vi "Auto_New.vi"() -> ()   [LabVIEW 2017]
uses:
  Control/Saurabh/prosucer_consumer_enum1.ctl
  Control/OUTPUT Cluster Indicator.ctl
  <vilib>/Utility/error.llb/DialogType.ctl
  <vilib>/addons/database/Connection.llb/DB Tools Open Connec (String).vi
  Global/DATA LOG.vi
  Global/Global 1.vi
  <vilib>/addons/database/NI_Database_API.lvlib
panel:
  out "SHIFT":string
  in  "BARCODE RECIPE":string(combo)
  out "PLC COM.":bool
  out "SHIFT_DATA":string[](array[string])
  out "stop":bool
  out "error out 2":errorcluster
  out "Shift 4":i32
  out "Time Stamp Out":timestamp[](array[timestamp]) format="%<%X>T"
  out "Time Stamp Out 4":timestamp[](array[timestamp]) format="%<%X>T"
  out "Shift_change":bool
  out "appended array":string[][](array[string])
  out "SHIFT_DATA 2":string[](array[string])
  in  "error in (no error)":errorcluster
  in  "Tab Control":T1(tab)
  out "OP 50":bool
  out "OP 40":bool
  out "OP 30":bool
  out "OP - 50":T2 {"RH Motor Screw" format="%#.2g N-m"; "LH Motor Screw" format="%#.2g N-m"; "Nut Torque" format="%#.2g N-m"}
  out "OP - 40":T3 {"Stack Load" format="%.2f kg"; "Dispalcement" format="%#.2g mm"; "LH Screw" format="%#.2g N-m"; "RH Screw" format="%#.2g N-m"}
  out "OP - 30":T4 {"Shaft Press Load" format="%#.2g kg"; "Displacement" format="%#.2g mm"}
  in  "stop 2":bool
  out "OP - 10":T5 {"Leak Rate" format="%#.2g SCCM"}
  in  "SIMULATE INPUT":bool[](array[boolean])=[FALSE, FALSE, FALSE, FALSE]
  out "OP - 20":T6 {"Top Load" format="%#.2g kg"; "Top Displace" format="%#.2g mm"; "Bottom Load" format="%#.2g kg"; "Bottom Displace" format="%#.2g mm"}
  out "OP 10 & 20":bool
  out "OP - 60":T7 {"Screw 6" format="%#.2g N-m"; "Screw 5" format="%#.2g N-m"; "Screw 4" format="%#.2g N-m"; "Screw 3" format="%#.2g N-m"; "Screw 2" format="%#.2g N-m"; "Screw 1" format="%#.2g N-m"}
  out "OP - 70":T8 {"Full Open" format="%#.4g V"; "Full Close" format="%#.4g V"}
  out "OP - 110":T9
  out "OP - 80":T10 {"Plug Press Load" format="%#.2f kg"}
  out "OP - 90":T11 {"Steam Leak" format="%#_g sccm"; "Seat Leak" format="%#_g LPM"}
  out "OP - 100":T12 {"Response Time REV" format="%#_g msec"; "Response time FWD" format="%#_g msec"; "Motor Full Open" format="%#.2f V"; "Motor Start Back" format="%#.2f V"; "Motor Full Close" format="%#.2f V"; "Motor Start Of Close" format="%#.2f V"; "Motor Peak" format="%#.2f A"; "Sensor O/P Full Close" format="%#.2f V"; "Sensor O/P Start Of Close" format="%#.2f V"; "Sensor O/P Open" format="%#.2f V"}
  out "OP 60":bool
  out "OP 70 & 80":bool
  out "OP 90 -100":bool
  out "OP 110":bool
  out "OP110 STATUS":dbl[](array[numeric])
  out "SCAN OP110":string[](array[string])
  out "OP100 STATUS":dbl[](array[numeric])
  out "SCAN OP100":string[](array[string])
  out "OP50 STATUS":dbl[](array[numeric])
  out "SCAN OP50":string[](array[string])
  out "OP90 STATUS":dbl[](array[numeric])
  out "SCAN OP90":string[](array[string])
  out "OP80 STATUS":dbl[](array[numeric])
  out "SCAN OP80":string[](array[string])
  out "OP70 STATUS":dbl[](array[numeric])
  out "SCAN OP70":string[](array[string])
  out "OP60 STATUS":dbl[](array[numeric])
  out "SCAN OP60":string[](array[string])
  out "OP40 STATUS":dbl[](array[numeric])
  out "SCAN OP40":string[](array[string])
  out "OP30 STATUS":dbl[](array[numeric])
  out "SCAN OP30":string[](array[string])
  out "OP20 STATUS":dbl[](array[numeric])
  out "SCAN OP20":string[](array[string])
  out "OP10 STATUS":dbl[](array[numeric])
  out "SCAN OP10":string[](array[string])
  out "resulting string":string
  out "PLC1 error":errorcluster
  out "PLC2 error":errorcluster
  out "PLC3 error":errorcluster
  out "PLC4 error":errorcluster
  out "PLC5 error":errorcluster
  out "PLC6 error":errorcluster
  out "PLC7 error":errorcluster
  out "PLC8 error":errorcluster
  # "Op10 20\nOp30\nOp 40\nOp50\nOp60\nOp70-80\nOp 90-100-110"
  # "SENSOR MIN VLTG"
  # "OP - 50"
  # "OP - 40"
  # "OP - 30"
  # "OP - 10"
  # "OP - 20"
  # "OP - 60"
  # "OP - 70"
  # "OP - 110"
  # "OP - 80"
  # "OP - 90"
  # "OP - 100"
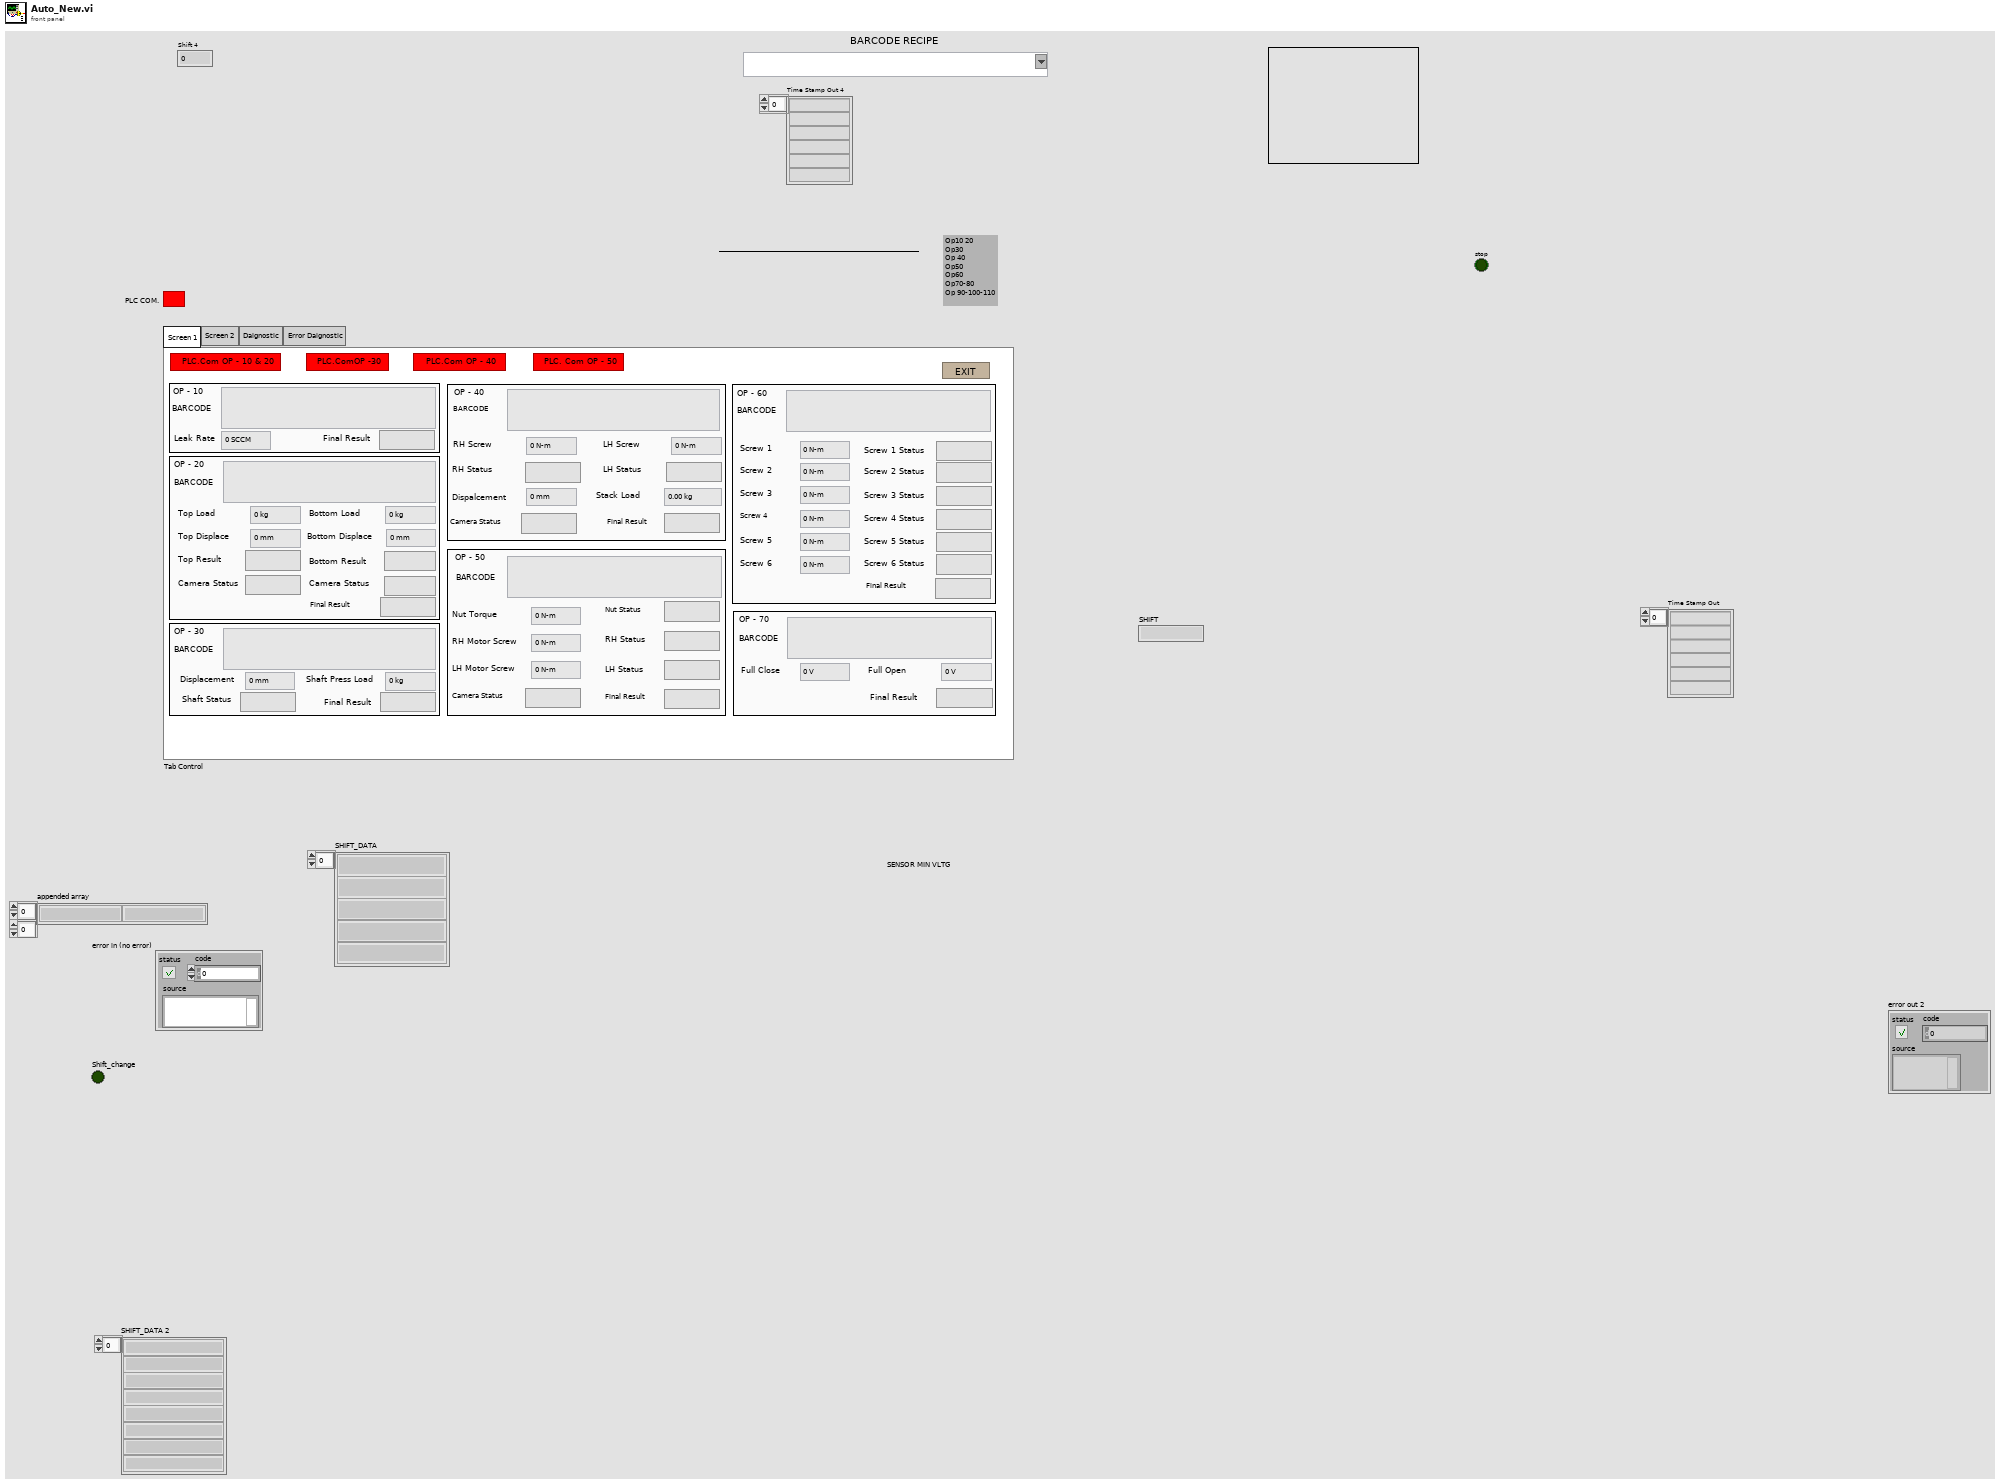
[diagram p1: front panel]
types:
  T1 = enum32{"Screen 1", "Screen 2", "Daignostic", "Error Daignostic"}
  T2 = cluster{"BARCODE":string, "Nut Torque":dbl, "LH Motor Screw":dbl, "LH Status":bool, "RH Status":bool, "RH Motor Screw":dbl, "Final Result":bool, "Nut Status":bool, "Camera Status":bool}
  T3 = cluster{"BARCODE":string, "RH Screw":dbl, "LH Screw ":dbl, "RH Status":bool, "LH Status":bool, "Dispalcement ":dbl, "Stack Load ":dbl, "Final Result":bool, "Camera Status":bool}
  T4 = cluster{"BARCODE":string, "Displacement":dbl, "Shaft Press Load":dbl, "Shaft Status":bool, "Final Result":bool}
  T5 = cluster{"BARCODE":string, "Leak Rate":dbl, "Final Result":bool}
  T6 = cluster{"BARCODE":string, "Bottom Displace":dbl, "Bottom Load":dbl, "Camera Status":bool, "Bottom Result":bool, "Top Displace":dbl, "Top Load ":dbl, "Camera Status":bool, "Top Result":bool, "Final Result":bool}
  T7 = cluster{"BARCODE":string, "Screw 1":dbl, "Screw 2":dbl, "Screw 1 Status":bool, "Screw 2 Status":bool, "Screw 3":dbl, "Final Result":bool, "Screw 3 Status":bool, "Screw 4":dbl, "Screw 5":dbl, "Screw 4 Status":bool, "Screw 5 Status":bool, "Screw 6":dbl, "Screw 6 Status":bool}
  T8 = cluster{"BARCODE":string, "Full Close":dbl, "Full Open":dbl, "Final Result":bool}
  T9 = cluster{"BARCODE":string, "BIN\nNumber":string, "PALLET\nNumber":string}
  T10 = cluster{"BARCODE":string, "Plug Press Load":dbl, "Final Result":bool, "Loctite Status":bool}
  T11 = cluster{"BARCODE":string, "Seat Leak":dbl, "Seat Status":bool, "Steam Leak":dbl, "Final Result":bool}
  T12 = cluster{"BARCODE":string, "Sensor O/P Open":dbl, "Sensor O/P Start Of Close":dbl, "Final Result":bool, "Sensor O/P Full Close":dbl, "Motor Peak":dbl, "Motor Start Of Close":dbl, "Motor Full Close":dbl, "Motor Start Back":dbl, "Motor Full Open":dbl, "Response time FWD":dbl, "Response Time REV":dbl, "Camera Status":bool}
  T13 = typedef "OUTPUT Cluster Indicator.ctl" = cluster{"OP - 10":cluster{"BARCODE":string, "LEAK RATE":dbl, "RESULT":bool}, "OP - 30":cluster{"BARCODE":string, "Displacement":dbl, "Load":dbl, "Middle Gear Shaft Status":bool, "Final Result":bool}, "OP - 60":cluster{"BARCODE":string, "Screw 1 Data":dbl, "Screw 2 data":dbl, "Screw 1 Status":bool, "Screw 2 Status":bool, "Screw3 Data":dbl, "Final Result":bool, "Screw3 Status":bool, "Screw4 Data":dbl, "Screw5 Data":dbl, "Screw4 Status":bool, "Screw5 Status":bool, "Screw6 Data":dbl, "Screw6 Status":bool}, "OP - 70":cluster{"BARCODE":string, "Sensor MIN Vltg":dbl, "Sensor MAX Vltg":dbl, "Final Result":bool}, "OP - 80":cluster{"BARCODE":string, "Load":dbl, "Final Result":bool, "Dispensing":bool}, "OP - 90":cluster{"BARCODE":string, "Seat LT Data":dbl, "Seat Status":bool, "Steam LT Data":dbl, "Final Result":bool}, "OP - 110":cluster{"BARCODE":string, "BIN\nNumber":string, "PALLET\nNumber":string}, "OP - 20":cluster{"BARCODE":string, "Bottom Displace":dbl, "Bottom Load":dbl, "Camera Status":bool, "Bottom Result":bool, "Top Displace":dbl, "Top Load ":dbl, "Camera Status":bool, "Top Result":bool, "Final Result":bool}, "OP - 50":cluster{"BARCODE":string, "Nut Torque":dbl, "LH Motor Screw":dbl, "LH Status":bool, "RH Status":bool, "RH Motor Screw":dbl, "Final Result":bool, "Nut Status":bool, "Camera Status":bool}, "OP - 100":cluster{"BARCODE":string, "Sensor O/P Open":dbl, "Sensor O/P Start Of Close":dbl, "Final Result":bool, "Sensor O/P Full Close":dbl, "Motor Peak":dbl, "Motor Start Of Close":dbl, "Motor Full Close":dbl, "Motor Start Back":dbl, "Motor Full Open":dbl, "Response time FWD":dbl, "Response Time REV":dbl, "Camera Status":bool}, "OP - 40":cluster{"BARCODE":string, "RH Screw":dbl, "LH Screw ":dbl, "RH Status":bool, "LH Status":bool, "Dispalcement ":dbl, "Stack Load ":dbl, "Final Result":bool, "Camera Status":bool}}
  T14 = cluster{"OP - 10":cluster{"BARCODE":string, "LEAK RATE":dbl, "RESULT":bool}, "OP - 30":cluster{"BARCODE":string, "Displacement":dbl, "Load":dbl, "Middle Gear Shaft Status":bool, "Final Result":bool}, "OP - 60":cluster{"BARCODE":string, "Screw 1 Data":dbl, "Screw 2 data":dbl, "Screw 1 Status":bool, "Screw 2 Status":bool, "Screw3 Data":dbl, "Final Result":bool, "Screw3 Status":bool, "Screw4 Data":dbl, "Screw5 Data":dbl, "Screw4 Status":bool, "Screw5 Status":bool, "Screw6 Data":dbl, "Screw6 Status":bool}, "OP - 70":cluster{"BARCODE":string, "Sensor MIN Vltg":dbl, "Sensor MAX Vltg":dbl, "Final Result":bool}, "OP - 80":cluster{"BARCODE":string, "Load":dbl, "Final Result":bool, "Dispensing":bool}, "OP - 90":cluster{"BARCODE":string, "Seat LT Data":dbl, "Seat Status":bool, "Steam LT Data":dbl, "Final Result":bool}, "OP - 110":cluster{"BARCODE":string}, "OP - 20":cluster{"BARCODE":string, "Bottom Displace":dbl, "Bottom Load":dbl, "Camera Status":bool, "Bottom Result":bool, "Top Displace":dbl, "Top Load ":dbl, "Camera Status":bool, "Top Result":bool, "Final Result":bool}, "OP - 40":cluster{"BARCODE":string, "RH Screw":dbl, "LH Screw ":dbl, "RH Status":bool, "LH Status":bool, "Dispalcement ":dbl, "Stack Load ":dbl, "Final Result":bool}, "OP - 50":cluster{"BARCODE":string, "Nut Torque":dbl, "LH Motor Screw":dbl, "LH Status":bool, "RH Status":bool, "RH Motor Screw":dbl, "Final Result":bool, "Nut Status":bool, "Camera Status":bool}, "OP - 100":cluster{"BARCODE":string, "Sensor O/P Open":dbl, "Sensor O/P Start Of Close":dbl, "Final Result":bool, "Sensor O/P Full Close":dbl, "Motor Peak":dbl, "Motor Start Of Close":dbl, "Motor Full Close":dbl, "Motor Start Back":dbl, "Motor Full Open":dbl, "Response time FWD":dbl, "Response Time REV":dbl, "Camera Status":bool}}
  T15 = typedef "prosucer_consumer_enum1.ctl" = enum16{"-1", "SCAN1", "SCAN2", "SCAN3", "SCAN4", "SCAN5", "SCAN6", "SCAN7", "SCAN8", "SCAN9", "SCAN10", "SCAN11", "STOP", "DATALOG1", "DATALOG2", "DATALOG3", "DATALOG4", "DATALOG5", "DATALOG6", "DATALOG7", "DATALOG8", "DATALOG9", "DATALOG10", "DATALOG11", "CYCLE_START1", "CYCLE_START2", "CYCLE_START3", "CYCLE_START4", "BARCODE RECIPE", "EMERGENCY STOP"}
  T16 = typedef "NI_Database_API.lvlib/Conn ObjectReference.ctl" = refnum<k1>
  T17 = typedef "DialogType.ctl" = u16
  T18 = cluster{"trimmed string":string, "SHIFT":string, "date/time string":string, string, "Input 2":string}
  T19 = cluster{"SHIFT":string, "date/time string":string, "Input 2":string, string}
  T20 = cluster{"date/time string":string, "Input 2":string, "Input 2":string, "Input 2":string, "Input 2":string, "Input 2":string, "Input 2":string, "Input 2":string, "Input 2":string, "Input 2":string, "Input 2":string}
  T21 = cluster{"date/time string":string, "SHIFT":string, "Input 2":string, "Input 2":string, "Input 2":string, "Input 2":string, "Input 2":string, "Input 2":string, "Input 2":string, "Input 2":string, "Input 2":string, "Input 2":string}
  T22 = cluster{"date/time string":string, "Input 2":string, "Input 2":string, "Input 2":string, "Input 2":string}
  T23 = cluster{"date/time string":string, "SHIFT":string, "Input 2":string, "Input 2":string, "Input 2":string, "Input 2":string}
  T24 = cluster{"date/time string":string, "Input 2":string, "Input 2":string, "Input 2":string, "Input 2":string, "Input 2":string, "Input 2":string, "Input 2":string, "Input 2":string}
  T25 = cluster{"date/time string":string, "SHIFT":string, "Input 2":string, "Input 2":string, "Input 2":string, "Input 2":string, "Input 2":string, "Input 2":string, "Input 2":string, "Input 2":string}
  T26 = cluster{"date/time string":string, "SHIFT":string, "Input 2":string, "Input 2":string, "Input 2":string, "Input 2":string, "Input 2":string, "Input 2":string}
  T27 = cluster{"date/time string":string, "Input 2":string, "Input 2":string, "Input 2":string, "Input 2":string, "Input 2":string, "Input 2":string, "Input 2":string, "Input 2":string, "Input 2":string, "Input 2":string, "Input 2":string, "Input 2":string, "Input 2":string}
  T28 = cluster{"date/time string":string, "SHIFT":string, "Input 2":string, "Input 2":string, "Input 2":string, "Input 2":string, "Input 2":string, "Input 2":string, "Input 2":string, "Input 2":string, "Input 2":string, "Input 2":string, "Input 2":string, "Input 2":string}
  T29 = cluster{"date/time string":string, "Input 2":string, "Input 2":string, "Input 2":string}
  T30 = cluster{"date/time string":string, "SHIFT":string, "Input 2":string, "Input 2":string, "Input 2":string}
  T31 = cluster{"Input 2":string, "SHIFT":string, "date/time string":string, "Input 2":string, "Input 2":string, "Input 2":string}
  T32 = cluster{"date/time string":string, "trimmed string":string, "trimmed string":string}
  T33 = cluster{"BARCODE":string, "Seat LT Data":dbl, "Seat Status":bool, "Steam LT Data":dbl, "Final Result":bool}
  T34 = cluster{"BARCODE":string, "LEAK RATE":dbl, "RESULT":bool}
  T35 = cluster{"BARCODE":string, "Displacement":dbl, "Load":dbl, "Middle Gear Shaft Status":bool, "Final Result":bool}
  T36 = cluster{"BARCODE":string, "Screw 1 Data":dbl, "Screw 2 data":dbl, "Screw 1 Status":bool, "Screw 2 Status":bool, "Screw3 Data":dbl, "Final Result":bool, "Screw3 Status":bool, "Screw4 Data":dbl, "Screw5 Data":dbl, "Screw4 Status":bool, "Screw5 Status":bool, "Screw6 Data":dbl, "Screw6 Status":bool}
  T37 = cluster{"BARCODE":string, "Sensor MIN Vltg":dbl, "Sensor MAX Vltg":dbl, "Final Result":bool}
  T38 = cluster{"BARCODE":string, "Load":dbl, "Final Result":bool, "Dispensing":bool}
  T39 = enum32{"invalid app kind", "Development System", "Run Time System", "Student Edition", "Embedded LabVIEW", "Evaluation", "Custom"}
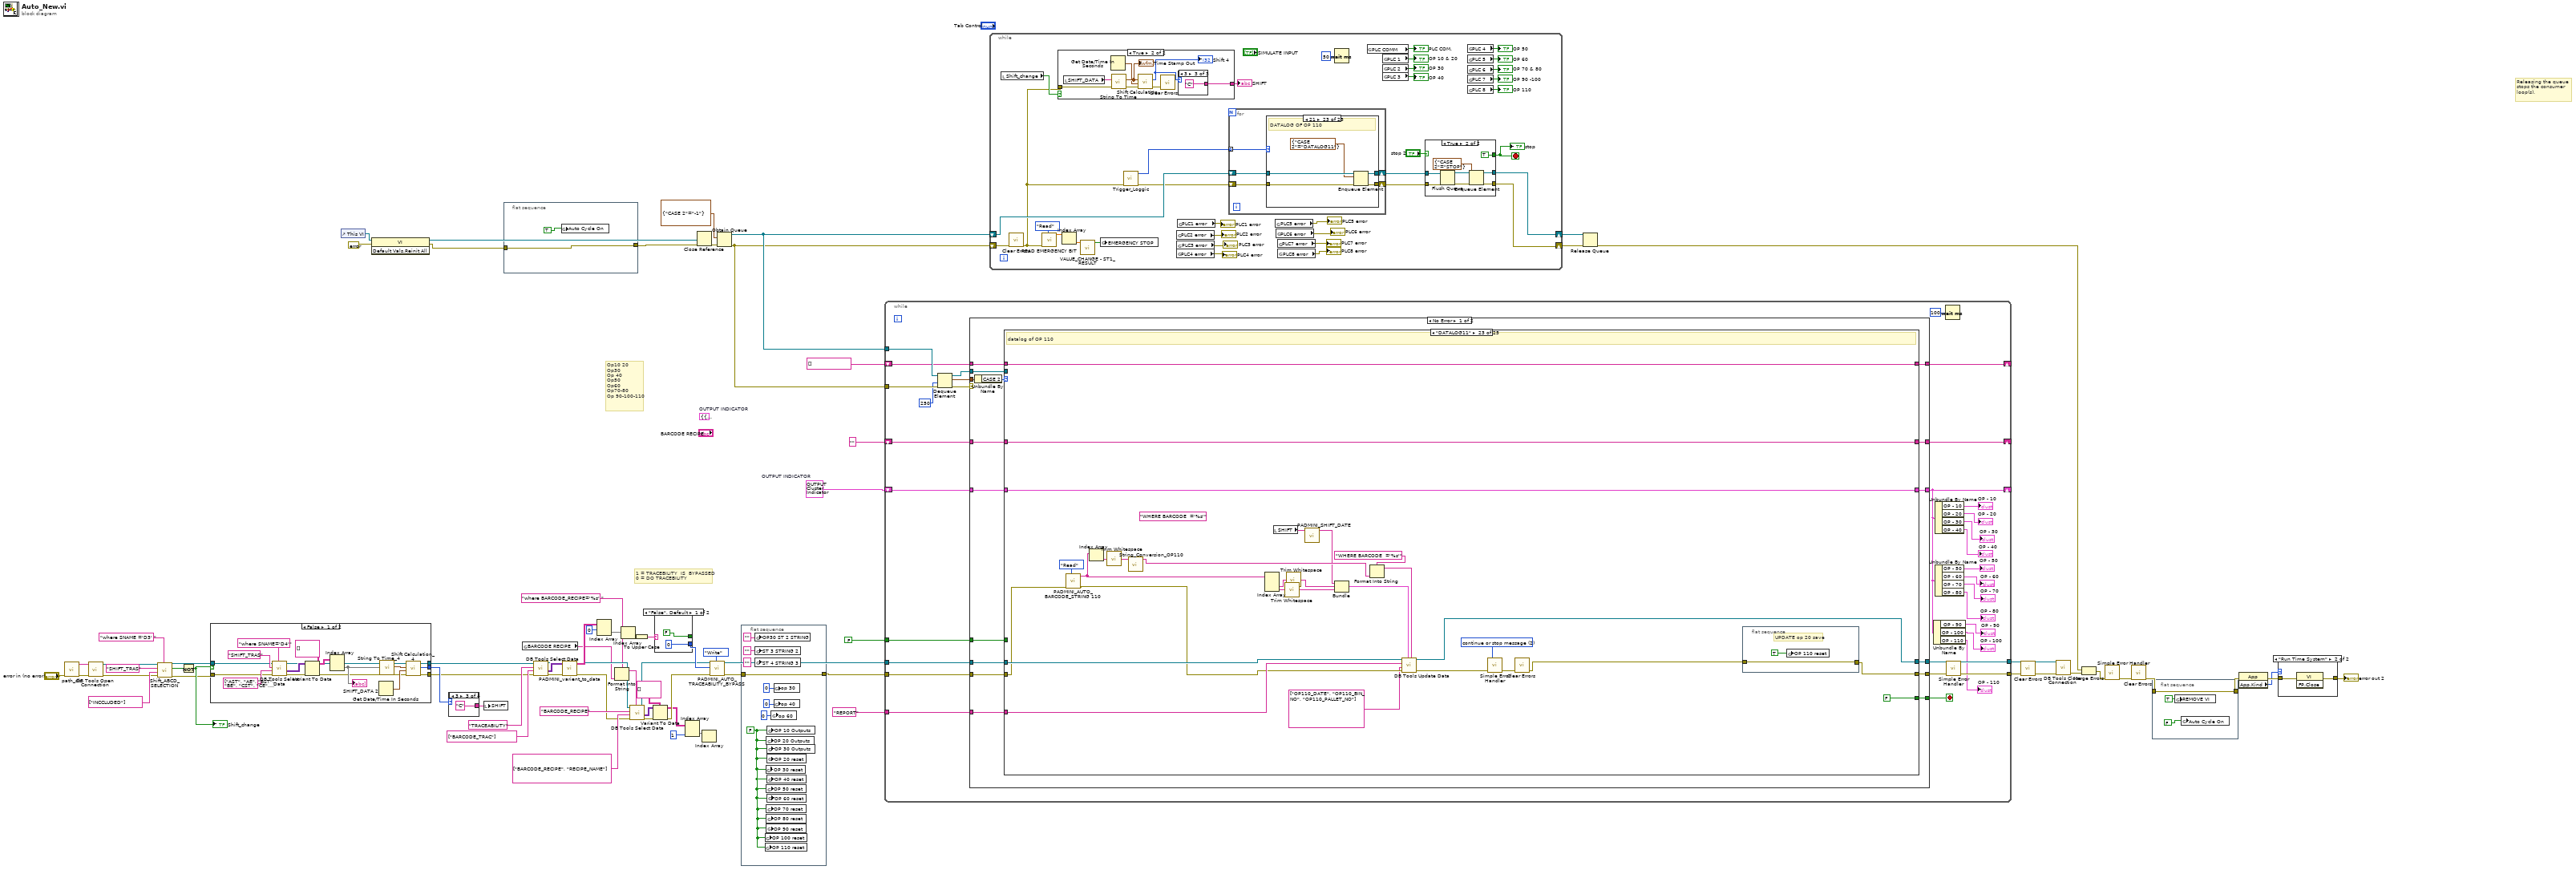
[diagram p0: block diagram]
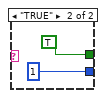
[diagram p2: hidden frame]
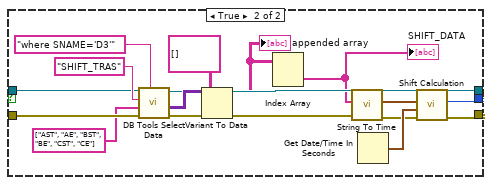
[diagram p3: hidden frame]
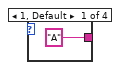
[diagram p4: hidden frame]
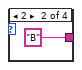
[diagram p5: hidden frame]
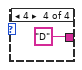
[diagram p6: hidden frame]
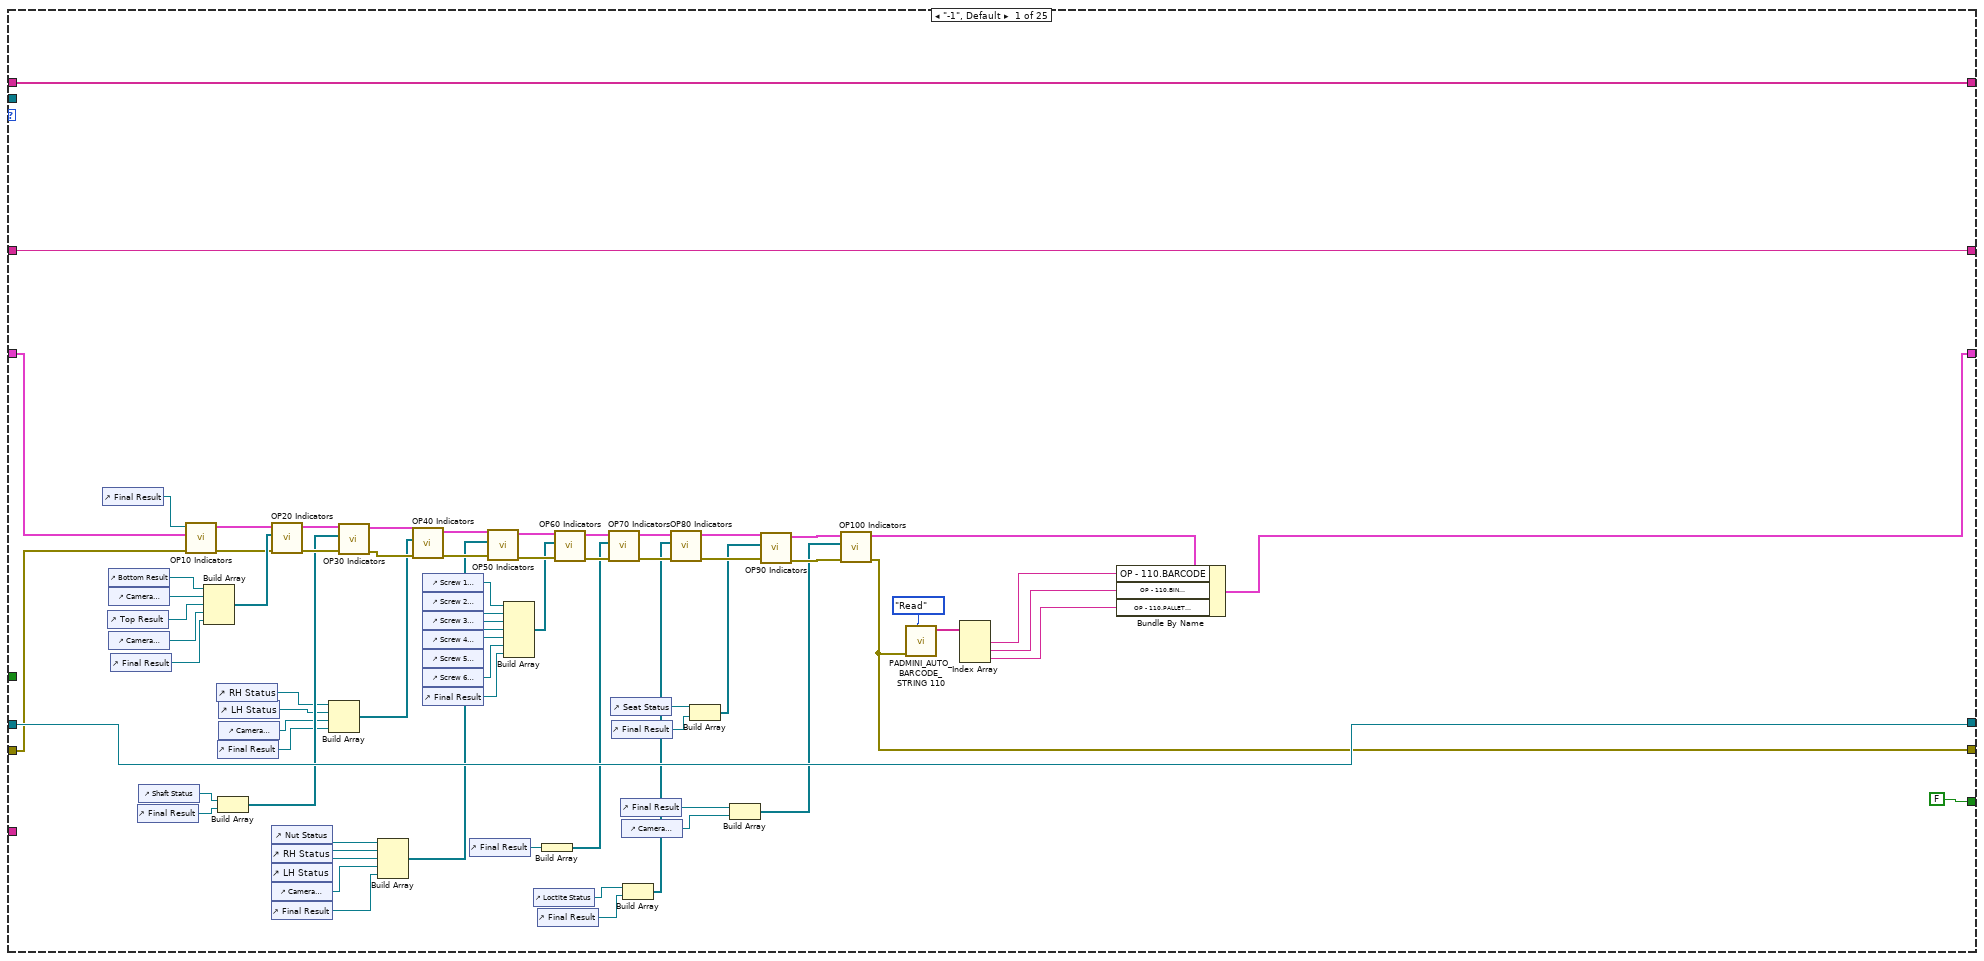
[diagram p7: hidden frame]
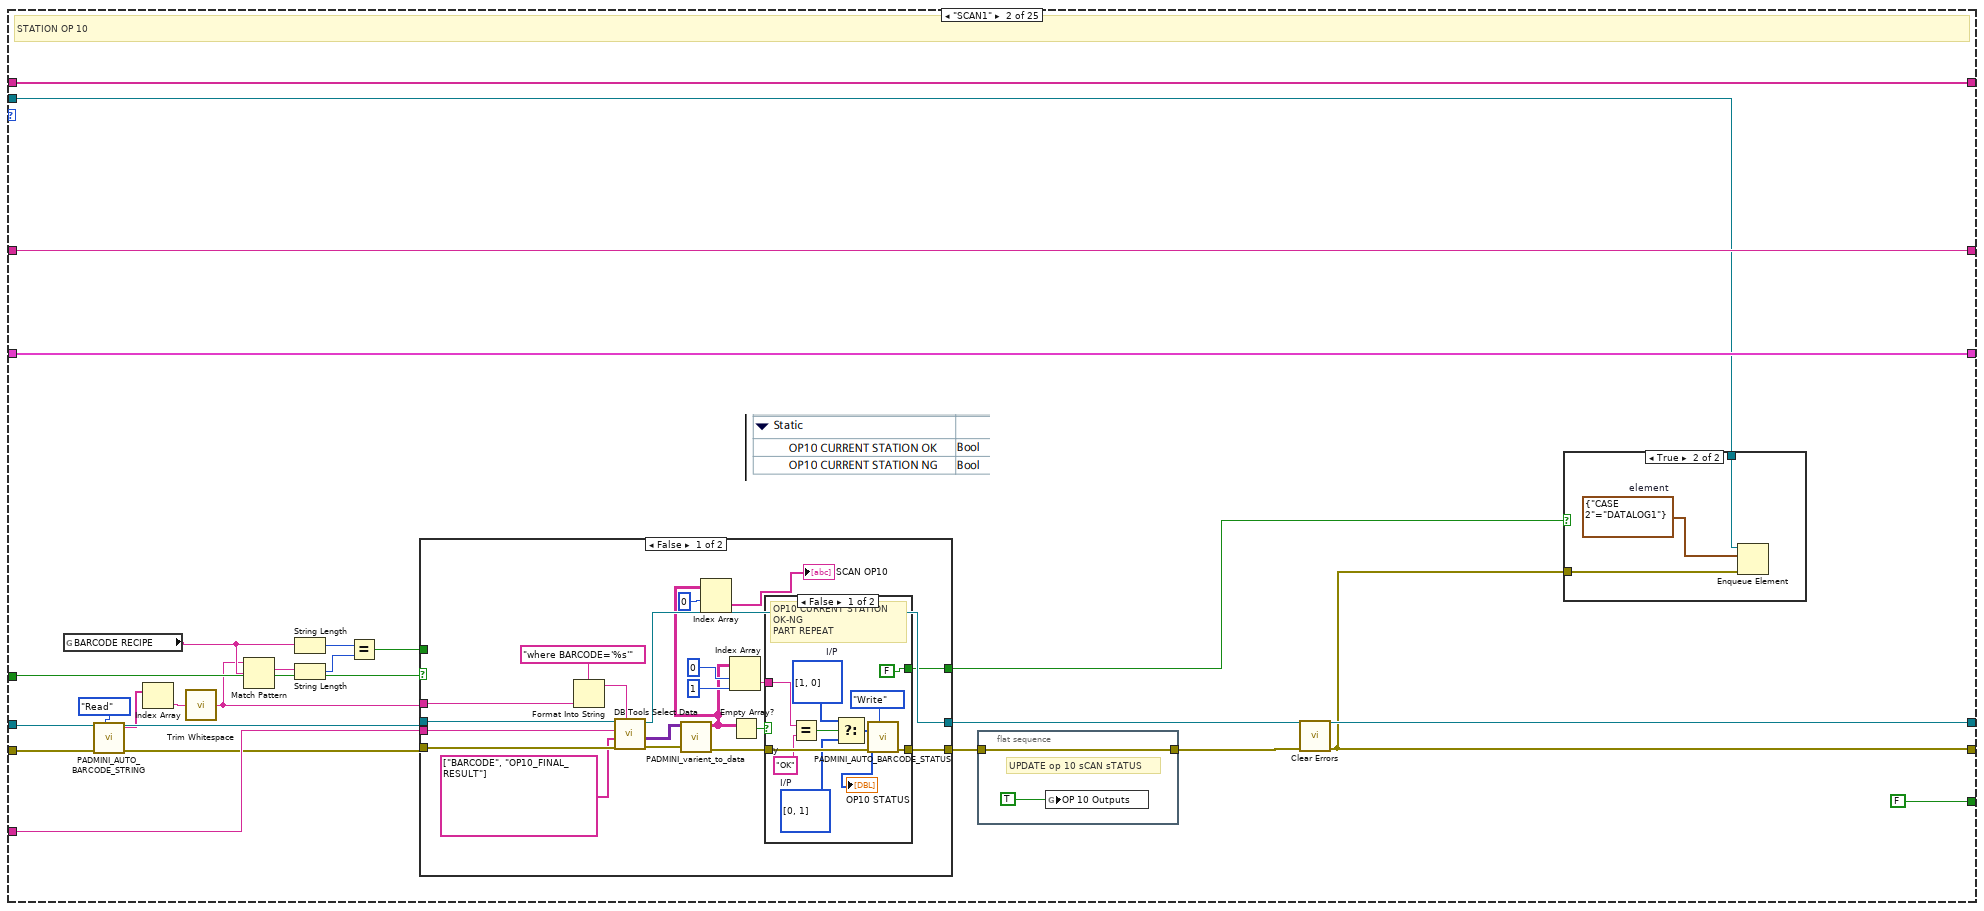
[diagram p8: hidden frame]
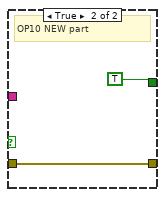
[diagram p10: hidden frame]
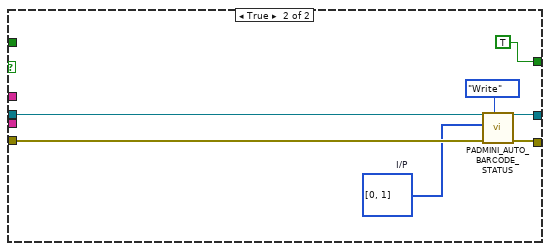
[diagram p11: hidden frame]
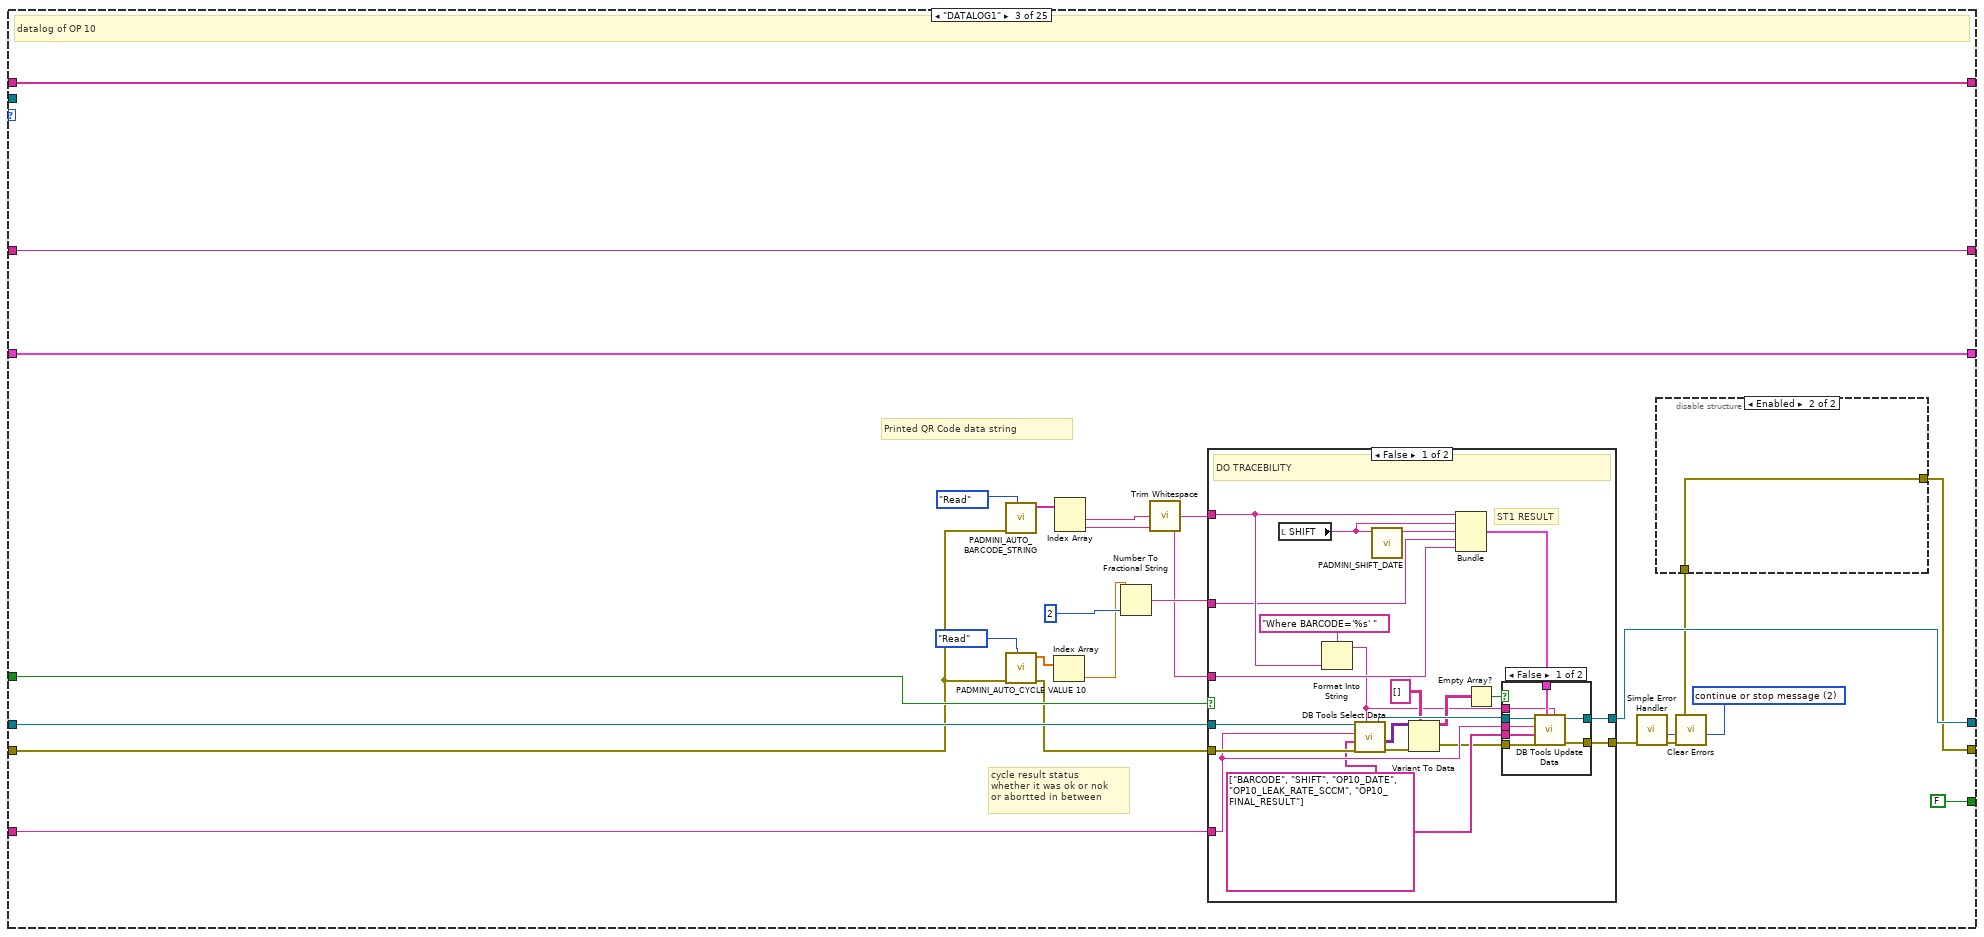
[diagram p12: hidden frame]
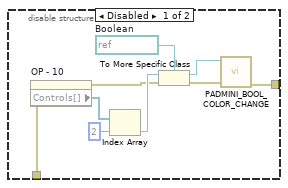
[diagram p13: hidden frame]
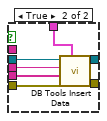
[diagram p14: hidden frame]
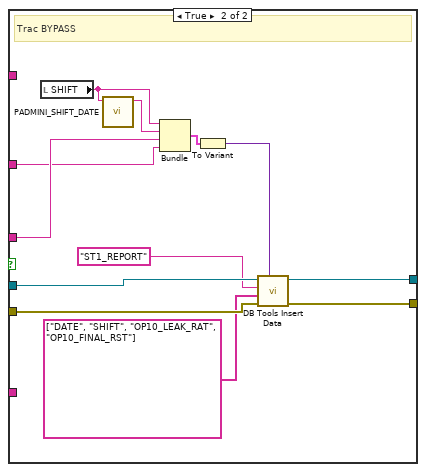
[diagram p15: hidden frame]
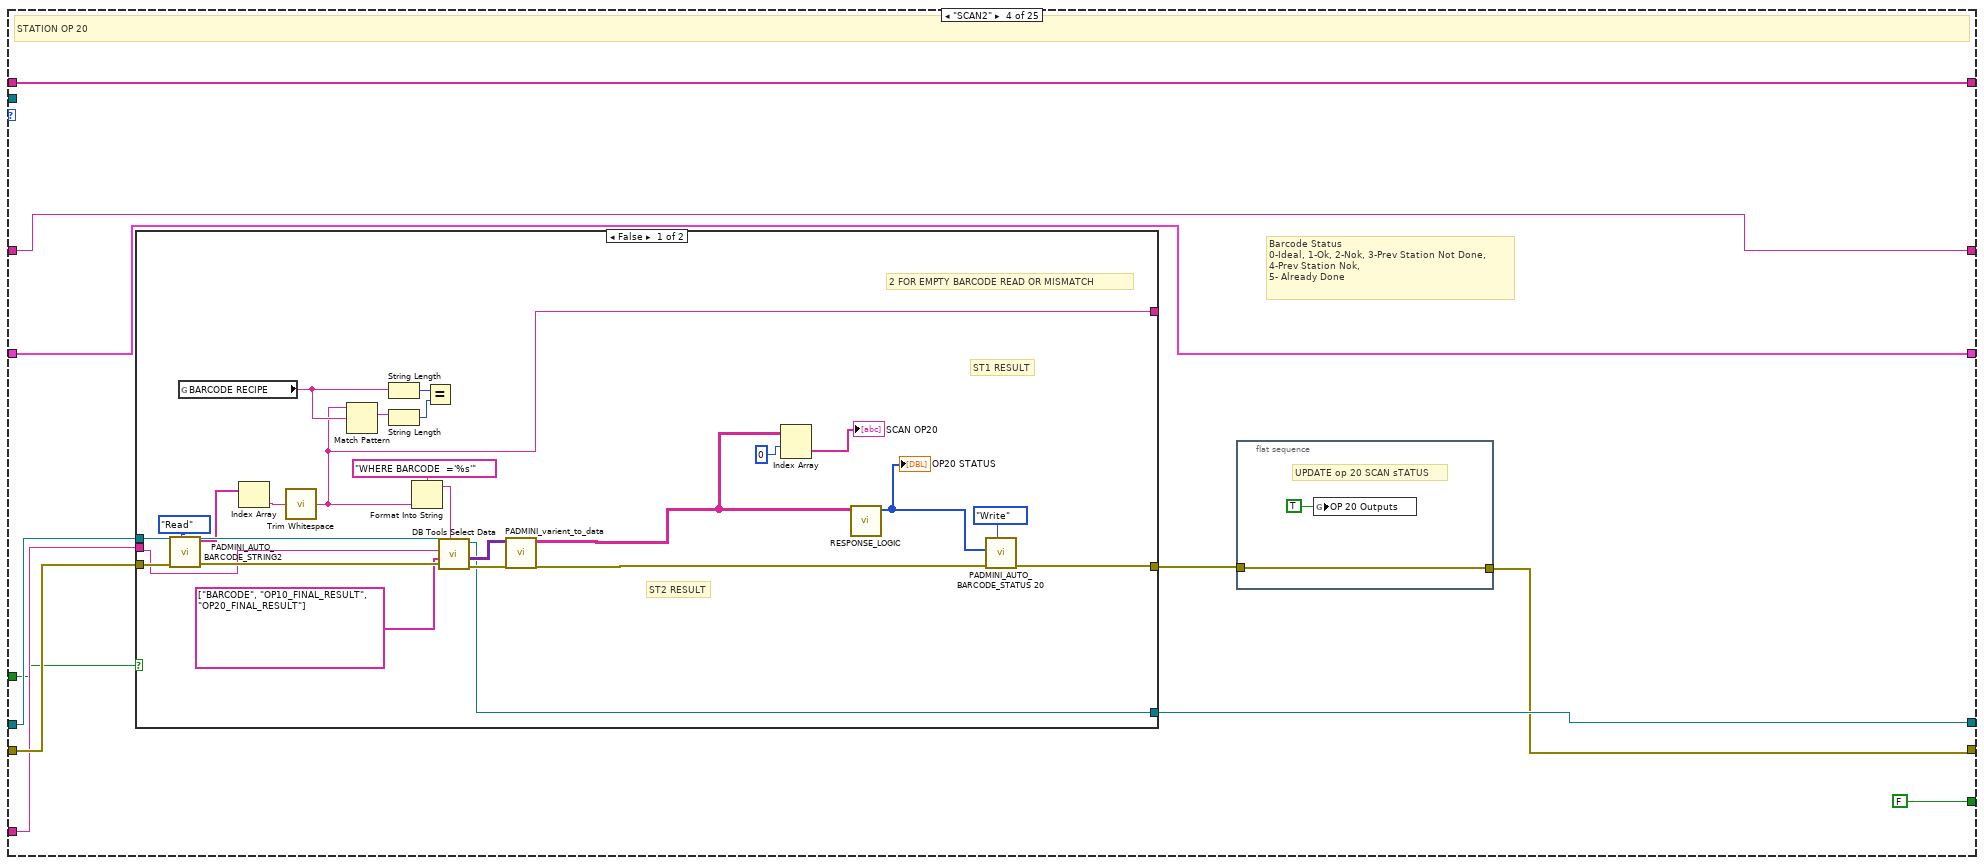
[diagram p16: hidden frame]
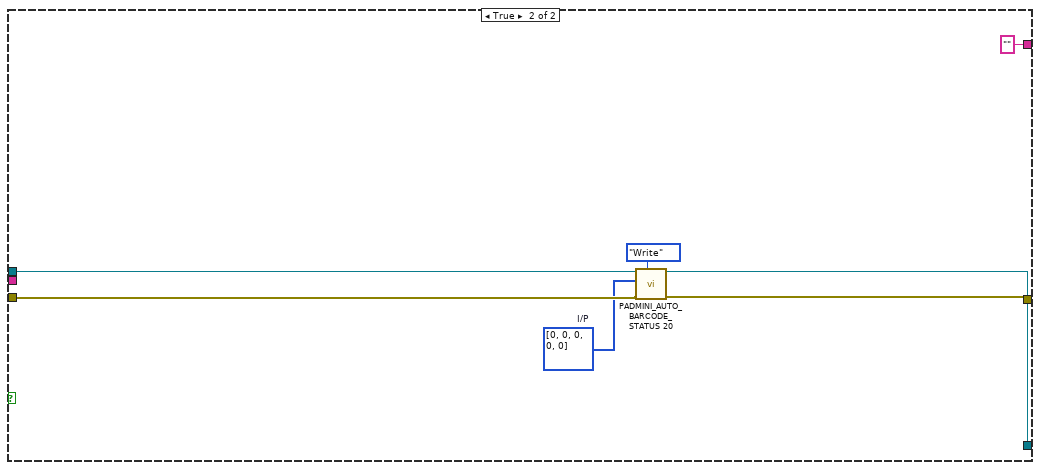
[diagram p17: hidden frame]
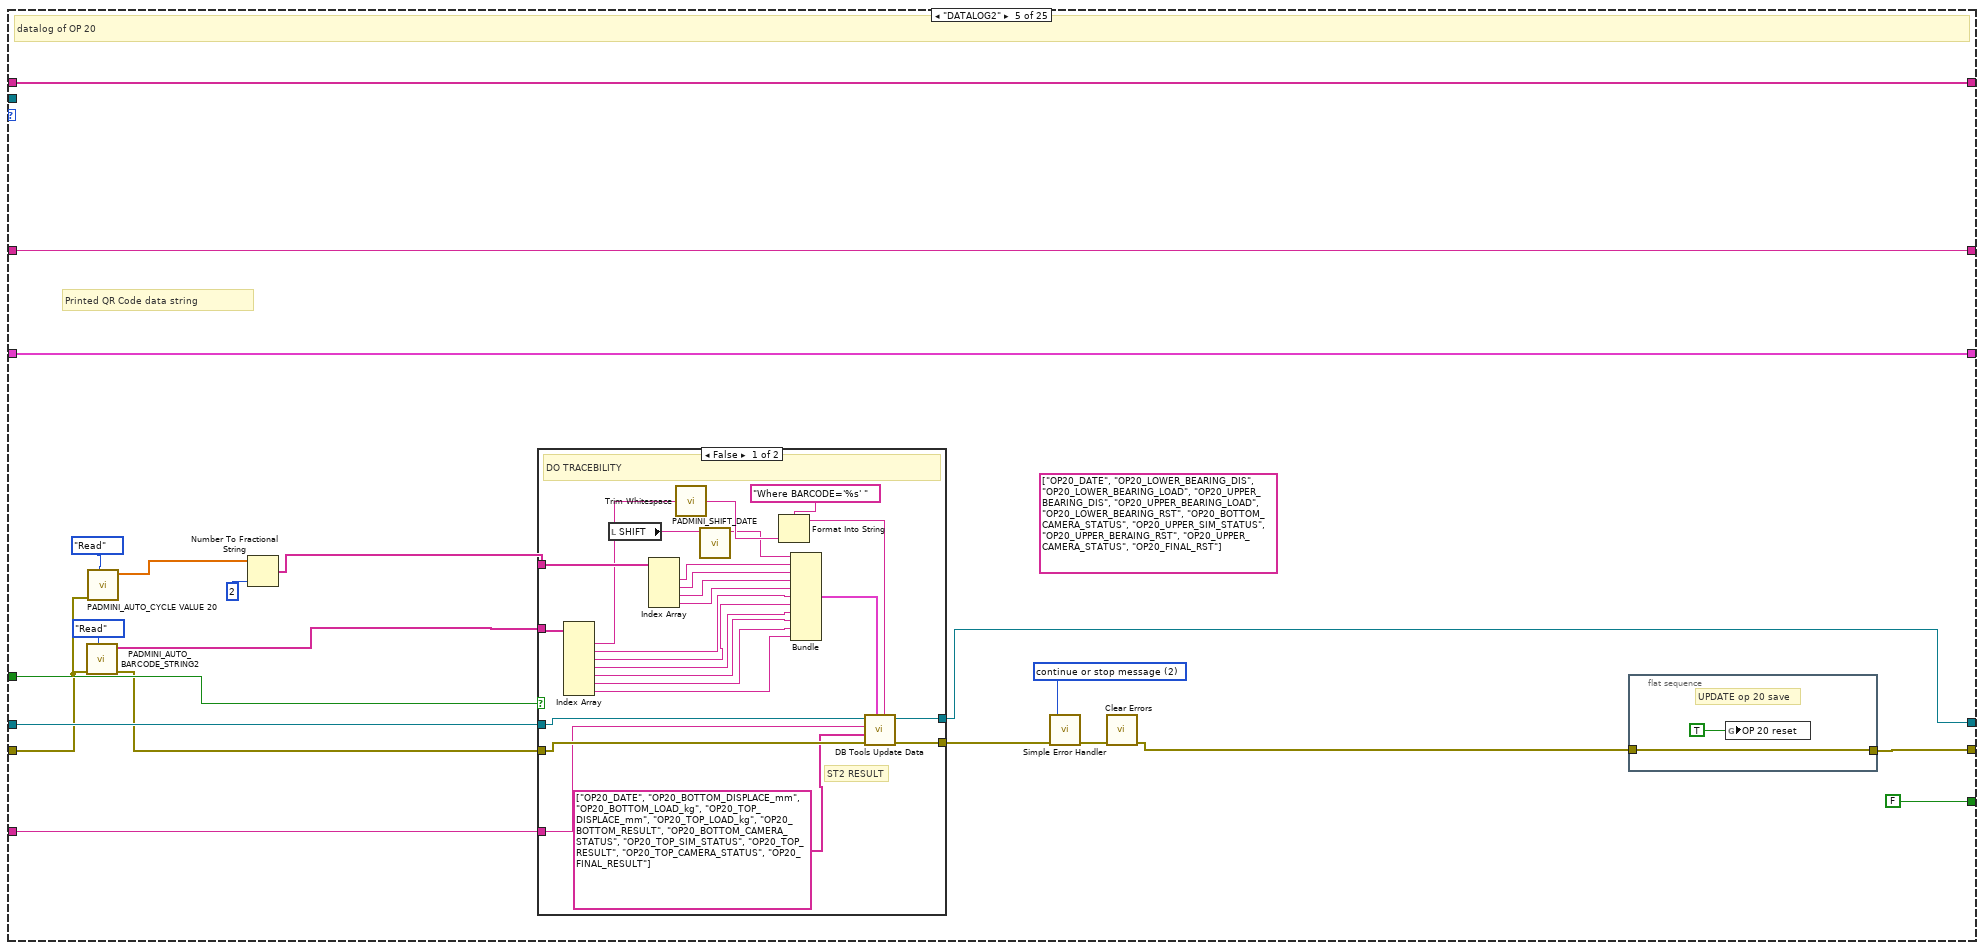
[diagram p18: hidden frame]
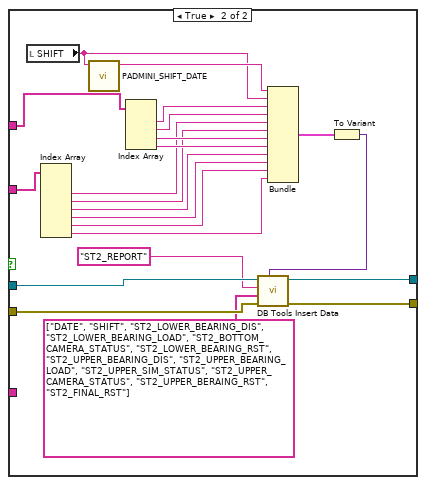
[diagram p19: hidden frame]
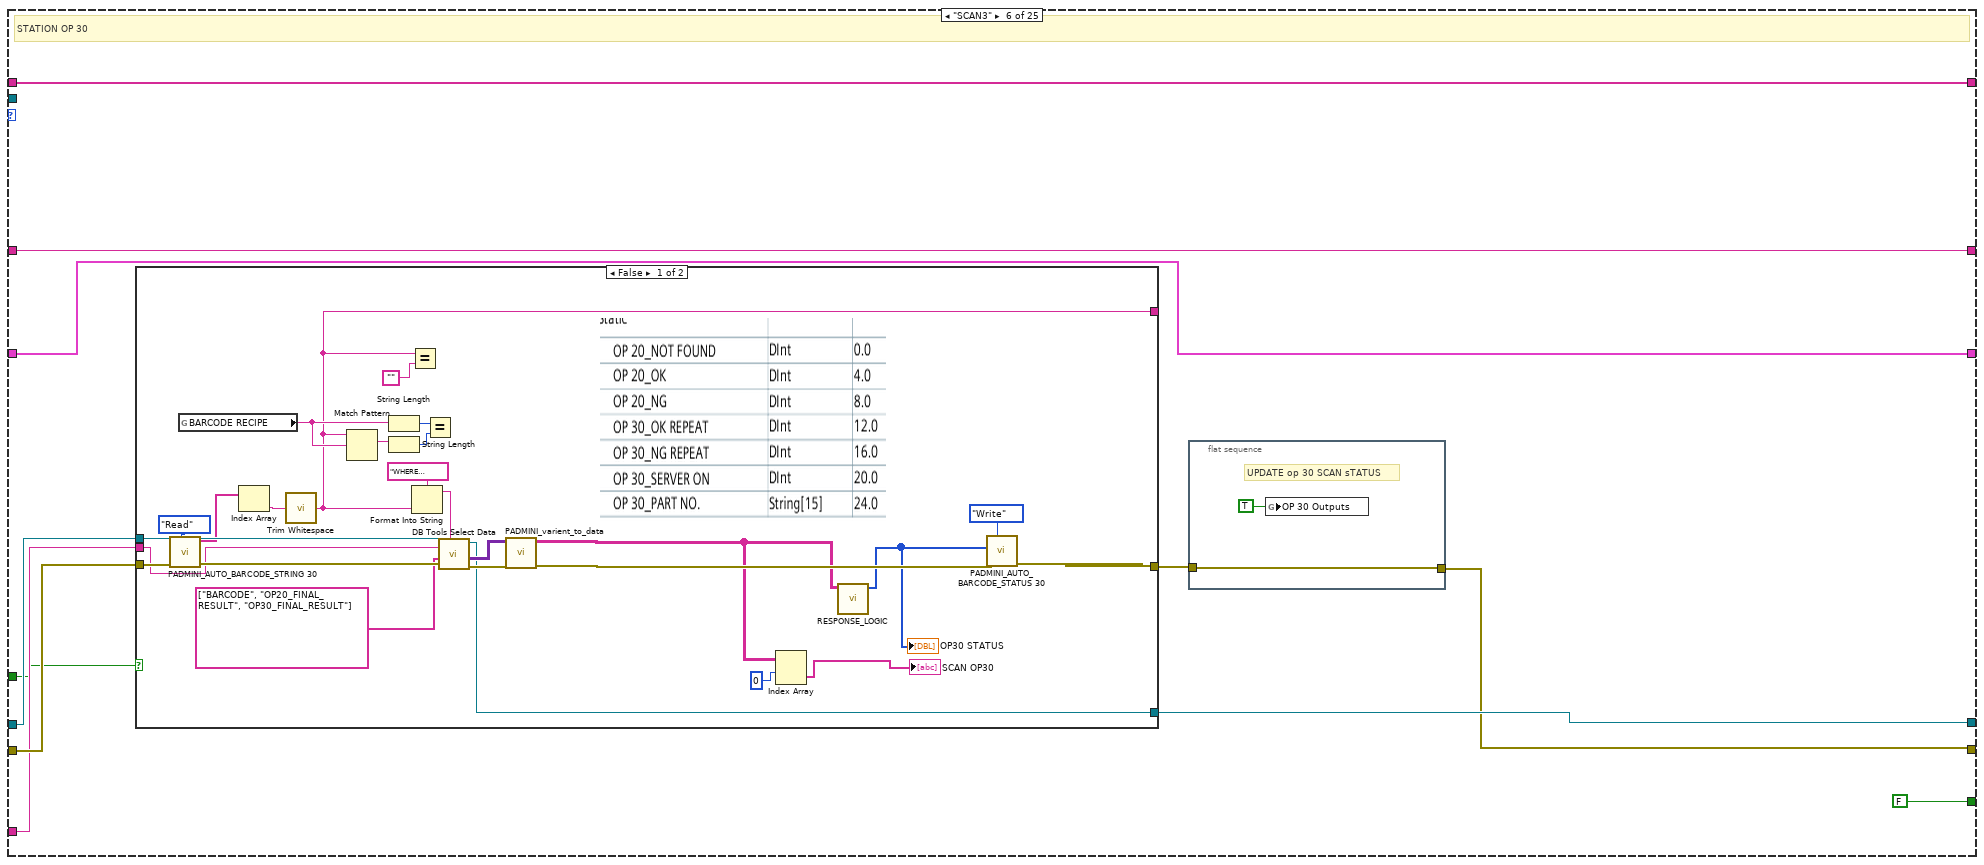
[diagram p20: hidden frame]
diagram:
  w1 = T13 {"OP - 10"={"BARCODE"="", "LEAK RATE"=0.0, "RESULT"=FALSE}, "OP - 30"={"BARCODE"="", "Displacement"=0.0, "Load"=0.0, "Middle Gear Shaft Status"=FALSE, "Final Result"=FALSE}, "OP - 60"={"BARCODE"="", "Screw 1 Data"=0.0, "Screw 2 data"=0.0, "Screw 1 Status"=FALSE, "Screw 2 Status"=FALSE, "Screw3 Data"=0.0, "Final Result"=FALSE, "Screw3 Status"=FALSE, "Screw4 Data"=0.0, "Screw5 Data"=0.0, "Screw4 Status"=FALSE, "Screw5 Status"=FALSE, "Screw6 Data"=0.0, "Screw6 Status"=FALSE}, "OP - 70"={"BARCODE"="", "Sensor MIN Vltg"=0.0, "Sensor MAX Vltg"=0.0, "Final Result"=FALSE}, "OP - 80"={"BARCODE"="", "Load"=0.0, "Final Result"=FALSE, "Dispensing"=FALSE}, "OP - 90"={"BARCODE"="", "Seat LT Data"=0.0, "Seat Status"=FALSE, "Steam LT Data"=0.0, "Final Result"=FALSE}, "OP - 110"={"BARCODE"="", "BIN\nNumber"="", "PALLET\nNumber"=""}, "OP - 20"={"BARCODE"="", "Bottom Displace"=0.0, "Bottom Load"=0.0, "Camera Status"=FALSE, "Bottom Result"=TRUE, "Top Displace"=0.0, "Top Load "=0.0, "Camera Status"=FALSE, "Top Result"=FALSE, "Final Result"=FALSE}, "OP - 50"={"BARCODE"="", "Nut Torque"=0.0, "LH Motor Screw"=0.0, "LH Status"=FALSE, "RH Status"=FALSE, "RH Motor Screw"=0.0, "Final Result"=FALSE, "Nut Status"=FALSE, "Camera Status"=FALSE}, "OP - 100"={"BARCODE"="", "Sensor O/P Open"=0.0, "Sensor O/P Start Of Close"=0.0, "Final Result"=FALSE, "Sensor O/P Full Close"=0.0, "Motor Peak"=0.0, "Motor Start Of Close"=0.0, "Motor Full Close"=0.0, "Motor Start Back"=0.0, "Motor Full Open"=0.0, "Response time FWD"=0.0, "Response Time REV"=0.0, "Camera Status"=FALSE}, "OP - 40"={"BARCODE"="", "RH Screw"=0.0, "LH Screw "=0.0, "RH Status"=FALSE, "LH Status"=FALSE, "Dispalcement "=0.0, "Stack Load "=0.0, "Final Result"=FALSE, "Camera Status"=TRUE}}  # OUTPUT INDICATOR
  (unwired) T14 {"OP - 10"={"BARCODE"="", "LEAK RATE"=0.0, "RESULT"=FALSE}, "OP - 30"={"BARCODE"="", "Displacement"=0.0, "Load"=0.0, "Middle Gear Shaft Status"=FALSE, "Final Result"=FALSE}, "OP - 60"={"BARCODE"="", "Screw 1 Data"=0.0, "Screw 2 data"=0.0, "Screw 1 Status"=FALSE, "Screw 2 Status"=FALSE, "Screw3 Data"=0.0, "Final Result"=FALSE, "Screw3 Status"=FALSE, "Screw4 Data"=0.0, "Screw5 Data"=0.0, "Screw4 Status"=FALSE, "Screw5 Status"=FALSE, "Screw6 Data"=0.0, "Screw6 Status"=FALSE}, "OP - 70"={"BARCODE"="", "Sensor MIN Vltg"=0.0, "Sensor MAX Vltg"=0.0, "Final Result"=FALSE}, "OP - 80"={"BARCODE"="", "Load"=0.0, "Final Result"=FALSE, "Dispensing"=FALSE}, "OP - 90"={"BARCODE"="", "Seat LT Data"=0.0, "Seat Status"=FALSE, "Steam LT Data"=0.0, "Final Result"=FALSE}, "OP - 110"={"BARCODE"=""}, "OP - 20"={"BARCODE"="", "Bottom Displace"=0.0, "Bottom Load"=0.0, "Camera Status"=FALSE, "Bottom Result"=TRUE, "Top Displace"=0.0, "Top Load "=0.0, "Camera Status"=FALSE, "Top Result"=FALSE, "Final Result"=FALSE}, "OP - 40"={"BARCODE"="", "RH Screw"=0.0, "LH Screw "=0.0, "RH Status"=FALSE, "LH Status"=FALSE, "Dispalcement "=0.0, "Stack Load "=0.0, "Final Result"=FALSE}, "OP - 50"={"BARCODE"="", "Nut Torque"=0.0, "LH Motor Screw"=0.0, "LH Status"=FALSE, "RH Status"=FALSE, "RH Motor Screw"=0.0, "Final Result"=FALSE, "Nut Status"=FALSE, "Camera Status"=FALSE}, "OP - 100"={"BARCODE"="", "Sensor O/P Open"=0.0, "Sensor O/P Start Of Close"=0.0, "Final Result"=FALSE, "Sensor O/P Full Close"=0.0, "Motor Peak"=0.0, "Motor Start Of Close"=0.0, "Motor Full Close"=0.0, "Motor Start Back"=0.0, "Motor Full Open"=0.0, "Response time FWD"=0.0, "Response Time REV"=0.0, "Camera Status"=FALSE}}  # OUTPUT INDICATOR
  # "Op10 20\nOp30\nOp 40\nOp50\nOp60\nOp70-80\nOp 90-100-110"
  # "1 = TRACEBILITY  IS  BYPASSED\n0 = DO TRACEBILITY"
  # "Releasing the queue stops the consumer loop(s)."
  n1 = call "path_db.vi"("error in"="error in (no error)") -> ("error out"=w48:errorcluster, "resulting string"=w69:string)  [unwired: 9 in]
  n2 = call-poly <vilib>:"DB Tools Open Connection.vi"("error in (no error)"=w48, "connection information"=w69) -> ("error out"=w47:errorcluster, "connection reference"=w41:T16)  [unwired: 6 in]
  n3 = call "Shift_ABCD_SELECTION.vi"("Where"="where SNAME ='D3' ", "error in (no error)"=w47, "Array"=string[] ["INCCLUDED"], "table"="SHIFT_TRAS", "Refnum in"=w41) -> ("error out"=w5:errorcluster, "Boolean"=w60:bool, "Refnum out"=w61:T16)  [unwired: 4 in]
  n4 = Not(x=w60) -> (.not. x?=w59:bool)
  "Shift_change" <- w59
  n5 = case shown="False" w59 {
    tunnel: [w74 w98] -> w65
    tunnel: w61 -> [w77 w96]
    tunnel: w5 -> [w76 w95]
    tunnel: [w75 w94] -> w30
    tunnel: [w73 w88] -> w29
    frame False {
      n6 = call <vilib>:"DB Tools Select Data.vi"("condition"="where SNAME='D4'", "error in (no error)"=w76, "columns"=string[] ["AST", "AE", "BST", "BE", "CST", "CE", "DST", "DE"], "table"="SHIFT_TRAS", "connection reference"=w77) -> ("error out"=w83:errorcluster, "data"=w87:variant[][], "connection reference out"=w75:T16)  [unwired: 1 in]
      n7 = Variant To Data(error in=w83, type=string[][] [], Variant=w87) -> (data=w80:string[][], error out=w73:errorcluster)
      n8 = Index Array(array=w80) -> (element=w79:string[])  [unwired: 2 in]
      "SHIFT_DATA 2" <- w79
      n9 = Get Date/Time In Seconds() -> (seconds since 1Jan1904=w82:timestamp)
      n10 = call "String To Time_4.vi"("String Array In"=w79) -> ("Time Stamp Out"=w78:timestamp[])  [unwired: 9 in, 1 out]
      n11 = call "Shift Calculation_4.vi"("Current Time"=w82, "Time Stamp Out"=w78) -> ("Shift"=w74:i32)  [unwired: 8 in, 1 out]
    }
    frame True {
      n12 = call <vilib>:"DB Tools Select Data.vi"("condition"="where SNAME='D3'", "error in (no error)"=w95, "columns"=string[] ["AST", "AE", "BST", "BE", "CST", "CE"], "table"="SHIFT_TRAS", "connection reference"=w96) -> ("error out"=w100:errorcluster, "data"=w104:variant[][], "connection reference out"=w94:T16)  [unwired: 1 in]
      n13 = Variant To Data(error in=w100, type=string[][] [], Variant=w104) -> (data=w92:string[][], error out=w90:errorcluster)
      "appended array" <- w92
      n14 = Index Array(array=w92) -> (element=w91:string[])  [unwired: 2 in]
      "SHIFT_DATA" <- w91
      n15 = call "String To Time.vi"("error in (no error)"=w90, "String Array In"=w91) -> ("error out"=w89:errorcluster, "Time Stamp Out"=w97:timestamp[])  [unwired: 8 in]
      n16 = Get Date/Time In Seconds() -> (seconds since 1Jan1904=w99:timestamp)
      n17 = call "Shift Calculation.vi"("error in (no error)"=w89, "Current Time"=w99, "Time Stamp Out"=w97) -> ("error out"=w88:errorcluster, "Shift"=w98:i32)  [unwired: 7 in]
    }
  }
  n18 = control-ref of="This VI"() -> (w45:refnum<vi>)
  n19 = invoke class="VI" method="Default Vals.Reinit All"(reference=w45, error in=errorcluster {"status"=FALSE, "code"=0, "source"=""} ("error in (no error)")) -> (reference out=w44:refnum<vi>, error out=w2:errorcluster)  [unwired: 1 in, 1 out]
  n20 = case shown="3" w65 {
    tunnel: ["A" "B" "C" "D"] -> w58
    frame 1, Default {
    }
    frame 2 {
    }
    frame 3 {
    }
    frame 4 {
    }
  }
  n21 = local write "SHIFT"(w58) -> ()
  n22 = flat-sequence {
    tunnel: [w110] -> w3
    tunnel: w2 -> [w110]
    frame #0 {
      n23 = global write "DATA LOG.vi" "Auto Cycle On"(TRUE) -> ()
    }
  }
  n24 = global read "Global 1.vi" "BARCODE RECIPE"() -> (w11:string)
  n25 = call <vilib>:"DB Tools Select Data.vi"("error in (no error)"=w29, "columns"=string[] ["BARCODE_TRAC"], "table"="TRACEABILITY", "connection reference"=w30) -> ("error out"=w39:errorcluster, "data"=w38:variant[][], "connection reference out"=w17:T16)  [unwired: 2 in]
  n26 = call "PADMINI_varient_to_data.vi"("error in (no error)"=w39, "data"=w38) -> ("error out"=w15:errorcluster, "Array"=w37:string[][])  [unwired: 8 in]
  n27 = Index Array(array=w37, index (row)=0 ("disabled index (col)")) -> (element=w36:string[])  [unwired: 1 in]
  n28 = Format Into String(format string="where BARCODE_RECIPE='%s' ", w11) -> (resulting string=w9:string)  [unwired: 2 in, 1 out]
  n29 = Index Array(array=w36) -> (element=w32:string)  [unwired: 1 in]
  n30 = call <vilib>:"DB Tools Select Data.vi"("condition"=w9, "error in (no error)"=w15, "columns"=string[] ["BARCODE_RECIPE", "RECIPE_NAME"], "table"="BARCODE_RECIPE", "connection reference"=w17) -> ("error out"=w19:errorcluster, "data"=w18:variant[][], "connection reference out"=w16:T16)  [unwired: 1 in]
  n31 = To Upper Case(1:w32) -> (0:w31:string)
  n32 = Variant To Data(error in=w19, type=string[][] [], Variant=w18) -> (data=w12:string[][], error out=w14:errorcluster)
  n33 = case shown="\"False\", Default" w31 {
    tunnel: [FALSE ("BARCODE TRACEABILITY") TRUE ("BARCODE TRACEABILITY")] -> _
    tunnel: [0 1] -> w27
    frame "False", Default {
    }
    frame "TRUE" {
    }
  }
  n34 = Index Array(array=w12, index (col)=1 ("disabled index (col)")) -> (element=w7:string[])  [unwired: 1 in]
  n35 = Close Reference(reference=w44, error in (no error)=w3) -> (error out=w42:errorcluster)
  n36 = Index Array(array=w7) -> ()  [unwired: 1 in, 1 out]
  n37 = call "PADMINI_AUTO_TRACEABILITY_BYPASS.vi"("Enum"=enum16{"Read", "Write"}."Write", "error in (no error)"=w14, "I/P"=w27) -> ("error out"=w25:errorcluster)  [unwired: 7 in, 1 out]
  n38 = Obtain Queue(element data type=cluster{"CASE 2":T15} {"CASE 2"=enum."-1"}, error in (no error)=w42) -> (queue out=w70:refnum<queue>, error out=w22:errorcluster)  [unwired: 3 in, 1 out]
  n39 = flat-sequence {
    tunnel: w25 -> [w119]
    tunnel: [w119] -> w24
    frame #0 {
      w115 = FALSE
      n40 = global write "DATA LOG.vi" "OP30 ST 2 STRING"("" ("OP30 ST 2 STRING")) -> ()
      n41 = global write "DATA LOG.vi" "ST 3 STRING 2"("" ("ST 3 STRING 2")) -> ()
      n42 = global write "DATA LOG.vi" "ST 4 STRING 3"("" ("ST 4 STRING 3")) -> ()
      n43 = global write "DATA LOG.vi" "OP 100 reset"(w115) -> ()
      n44 = global write "DATA LOG.vi" "OP 110 reset"(w115) -> ()
      n45 = global write "DATA LOG.vi" "OP 30 reset"(w115) -> ()
      n46 = global write "DATA LOG.vi" "OP 20 Outputs"(w115) -> ()
      n47 = global write "DATA LOG.vi" "OP 50 reset"(w115) -> ()
      n48 = global write "DATA LOG.vi" "OP 70 reset"(w115) -> ()
      n49 = global write "DATA LOG.vi" "OP 80 reset"(w115) -> ()
      n50 = global write "DATA LOG.vi" "OP 90 reset"(w115) -> ()
      n51 = global write "DATA LOG.vi" "OP 10 Outputs"(w115) -> ()
      n52 = global write "DATA LOG.vi" "OP 30 Outputs"(w115) -> ()
      n53 = global write "DATA LOG.vi" "OP 20 reset"(w115) -> ()
      n54 = global write "DATA LOG.vi" "OP 40 reset"(w115) -> ()
      n55 = global write "DATA LOG.vi" "OP 60 reset"(w115) -> ()
      n56 = global write "DATA LOG.vi" "op 60"(0 ("op 30")) -> ()
      n57 = global write "DATA LOG.vi" "op 30"(0 ("op 30")) -> ()
      n58 = global write "DATA LOG.vi" "op 40"(0 ("op 30")) -> ()
    }
  }
  n59 = while {
    tunnel: w70 -> [w154]
    tunnel: w22 -> [w150]
    tunnel: w24 -> [w149]
    tunnel: w16 -> [w148]
    tunnel: [w124] -> w68
    tunnel: [w147] -> w67
    tunnel: FALSE -> [w146]
    tunnel: "REPORT" -> [w145]
    shift-right: [w143] -> _
    shift-left: string[] [] -> [w144]
    shift-right: [w142] -> _
    shift-left: "" ("trimmed string") -> [w141]
    shift-right: [w130] -> _
    shift-left: w1 -> [w139]
    stop <- w151 stop-if-true
    n60 = Dequeue Element(queue=w154, timeout in ms (-1)=250, error in (no error)=w150) -> (queue out=w127:refnum<queue>, element=w152:cluster{"CASE 2":T15}, error out=w153:errorcluster)  [unwired: 1 out]
    n61 = case shown="No Error" w153 {
      tunnel: w152 -> [w170 _]
      tunnel: [w166 TRUE] -> w151
      tunnel: w149 -> [w167 w1460]
      tunnel: w148 -> [w168 w1459]
      tunnel: [w164 w1460] -> w125
      tunnel: [w165 w1459] -> w147
      tunnel: w146 -> [w163 _]
      tunnel: w145 -> [w162 _]
      tunnel: w144 -> [w161 w1458]
      tunnel: [w160 w1458] -> w143
      tunnel: [w159 w1457] -> w142
      tunnel: w141 -> [w158 w1457]
      tunnel: w139 -> [w157 w1456]
      tunnel: [w156 w1456] -> w130
      tunnel: w127 -> [w155 _]
      frame No Error {
        n62 = Unbundle By Name(w170) -> ("CASE 2"=w169:T15)
        n63 = case shown="\"DATALOG11\"" w169 {
          tunnel: w168 -> [w241 w265 w333 w403 w456 w517 w571 w620 w669 w726 w775 w830 w879 w945 w991 w1038 w1087 w1135 w1184 w1233 w1273 w1353 w1434 w1443 w1451]
          tunnel: w167 -> [w238 w261 w310 w402 w443 w516 w557 w619 w655 w725 w762 w829 w865 w944 w980 w1037 w1074 w1134 w1170 w1232 w1272 w1335 w1420 w1442 w1453]
          tunnel: [FALSE FALSE FALSE FALSE FALSE FALSE FALSE FALSE FALSE FALSE FALSE FALSE FALSE FALSE FALSE FALSE FALSE FALSE FALSE FALSE FALSE FALSE FALSE FALSE TRUE] -> w166
          tunnel: [w241 w263 w330 w400 w453 w514 w568 w617 w666 w723 w772 w827 w876 w942 w988 w1035 w1085 w1132 w1181 w1230 w1270 w1350 w1432 w1443 w1450] -> w165
          tunnel: [w176 w243 w329 w397 w438 w511 w552 w614 w650 w720 w757 w824 w860 w939 w975 w1032 w1069 w1129 w1165 w1227 w1267 w1334 w1424 w1442 w1452] -> w164
          tunnel: w163 -> [_ w258 w332 w399 w455 w513 w570 w616 w668 w722 w774 w826 w878 w941 w990 w1034 w1068 w1131 w1183 w1229 w1269 w1352 _ _ _]
          tunnel: w162 -> [_ w264 w331 w401 w454 w515 w569 w618 w667 w724 w773 w828 w877 w943 w989 w1036 w1086 w1133 w1182 w1231 w1271 w1351 w1433 _ _]
          tunnel: w161 -> [w240 w262 w326 w394 w452 w509 w567 w612 w665 w718 w771 w822 w875 w937 w987 w1030 w1084 w1127 w1180 w1225 w1265 w1349 w1431 w1440 w1454]
          tunnel: [w240 w262 w326 w394 w452 w509 w567 w612 w665 w718 w771 w822 w875 w937 w987 w1030 w1084 w1127 w1180 w1225 w1265 w1349 w1431 w1440 w1454] -> w160
          tunnel: [w239 w257 w322 w395 w448 w508 w563 w611 w661 w717 w767 w821 w871 w936 w985 w1029 w1080 w1126 w1176 w1224 w1264 w1345 w1427 w1439 w1445] -> w159
          tunnel: w158 -> [w239 w257 w322 w395 w448 w508 w563 w611 w661 w717 w767 w821 w871 w936 w985 w1029 w1080 w1126 w1176 w1224 w1264 w1345 w1427 w1439 w1445]
          tunnel: w157 -> [w237 w251 w320 w393 w437 w507 w561 w610 w659 w716 w756 w820 w869 w935 w984 w1028 w1078 w1125 w1174 w1223 w1263 w1343 w1425 w1438 w1444]
          tunnel: [w180 w251 w320 w393 w437 w507 w561 w610 w659 w716 w756 w820 w869 w935 w984 w1028 w1078 w1125 w1174 w1223 w1263 w1343 w1425 w1438 w1444] -> w156
          tunnel: w155 -> [_ w245 _ _ _ _ _ _ _ _ _ _ _ _ _ _ _ _ _ _ _ _ _ _ _]
          frame "-1", Default {
            n64 = control-ref of="Final Result"() -> (w228:refnum<vi>)
            n65 = control-ref of="Top Result"() -> (w232:refnum<vi>)
            n66 = control-ref of="Bottom Result"() -> (w234:refnum<vi>)
            n67 = control-ref of="Camera Status"() -> (w233:refnum<vi>)
            n68 = control-ref of="Camera Status"() -> (w231:refnum<vi>)
            n69 = control-ref of="Final Result"() -> (w230:refnum<vi>)
            n70 = control-ref of="Final Result"() -> (w224:refnum<vi>)
            n71 = control-ref of="Shaft Status"() -> (w225:refnum<vi>)
            n72 = call "OP10 Indicators.vi"("error in (no error)"=w238, "OUTPUT INDICATOR"=w237, "Boolean in"=w228) -> ("error out"=w227:errorcluster, "OUTPUT INDICATOR"=w236:T13)  [unwired: 7 in]
            n73 = Build Array(w234, w233, w232, w231, w230) -> (w229:refnum<vi>[])
            n74 = control-ref of="RH Status"() -> (w220:refnum<vi>)
            n75 = control-ref of="Final Result"() -> (w174:refnum<vi>)
            n76 = Build Array(w225, w224) -> (w223:refnum<vi>[])
            n77 = control-ref of="LH Status"() -> (w219:refnum<vi>)
            n78 = control-ref of="Camera Status"() -> (w173:refnum<vi>)
            n79 = call "OP20 Indicators.vi"("error in (no error)"=w227, "Array"=w229, "OUTPUT INDICATOR"=w236) -> ("error out"=w226:errorcluster, "OUTPUT INDICATOR"=w235:T13)  [unwired: 7 in]
            n80 = control-ref of="Nut Status"() -> (w215:refnum<vi>)
            n81 = control-ref of="RH Status"() -> (w214:refnum<vi>)
            n82 = control-ref of="LH Status"() -> (w213:refnum<vi>)
            n83 = control-ref of="Camera Status"() -> (w212:refnum<vi>)
            n84 = control-ref of="Final Result"() -> (w211:refnum<vi>)
            n85 = Build Array(w220, w219, w173, w174) -> (w218:refnum<vi>[])
            n86 = call "OP30 Indicators.vi"("error in (no error)"=w226, "Array"=w223, "OUTPUT INDICATOR"=w235) -> ("error out"=w221:errorcluster, "OUTPUT INDICATOR"=w222:T13)  [unwired: 7 in]
            n87 = Build Array(w215, w214, w213, w212, w211) -> (w210:refnum<vi>[])
            n88 = call "OP40 Indicators.vi"("error in (no error)"=w221, "Array"=w218, "OUTPUT INDICATOR"=w222) -> ("error out"=w217:errorcluster, "OUTPUT INDICATOR"=w216:T13)  [unwired: 7 in]
            n89 = control-ref of="Screw 1 Status"() -> (w206:refnum<vi>)
            n90 = control-ref of="Screw 2 Status"() -> (w205:refnum<vi>)
            n91 = control-ref of="Screw 3 Status"() -> (w204:refnum<vi>)
            n92 = control-ref of="Screw 4 Status"() -> (w203:refnum<vi>)
            n93 = control-ref of="Screw 5 Status"() -> (w202:refnum<vi>)
            n94 = control-ref of="Screw 6 Status"() -> (w201:refnum<vi>)
            n95 = control-ref of="Final Result"() -> (w200:refnum<vi>)
            n96 = control-ref of="Final Result"() -> (w197:refnum<vi>)
            n97 = call "OP50 Indicators.vi"("error in (no error)"=w217, "Array"=w210, "OUTPUT INDICATOR"=w216) -> ("error out"=w209:errorcluster, "OUTPUT INDICATOR"=w208:T13)  [unwired: 7 in]
            n98 = Build Array(w206, w205, w204, w203, w202, w201, w200) -> (w207:refnum<vi>[])
            n99 = control-ref of="Loctite Status"() -> (w193:refnum<vi>)
            n100 = control-ref of="Final Result"() -> (w192:refnum<vi>)
            n101 = Build Array(w197) -> (w196:refnum<vi>[])
            n102 = call "OP60 Indicators.vi"("error in (no error)"=w209, "Array"=w207, "OUTPUT INDICATOR"=w208) -> ("error out"=w199:errorcluster, "OUTPUT INDICATOR"=w198:T13)  [unwired: 7 in]
            n103 = call "OP70 Indicators.vi"("error in (no error)"=w199, "Array"=w196, "OUTPUT INDICATOR"=w198) -> ("error out"=w195:errorcluster, "OUTPUT INDICATOR"=w194:T13)  [unwired: 7 in]
            n104 = control-ref of="Seat Status"() -> (w188:refnum<vi>)
            n105 = control-ref of="Final Result"() -> (w187:refnum<vi>)
            n106 = control-ref of="Final Result"() -> (w183:refnum<vi>)
            n107 = control-ref of="Camera Status"() -> (w175:refnum<vi>)
            n108 = Build Array(w193, w192) -> (w191:refnum<vi>[])
            n109 = call "OP80 Indicators.vi"("error in (no error)"=w195, "Array"=w191, "OUTPUT INDICATOR"=w194) -> ("error out"=w189:errorcluster, "OUTPUT INDICATOR"=w190:T13)  [unwired: 7 in]
            n110 = Build Array(w188, w187) -> (w186:refnum<vi>[])
            n111 = Build Array(w183, w175) -> (w182:refnum<vi>[])
            n112 = call "OP90 Indicators.vi"("error in (no error)"=w189, "Array"=w186, "OUTPUT INDICATOR"=w190) -> ("error out"=w185:errorcluster, "OUTPUT INDICATOR"=w184:T13)  [unwired: 7 in]
            n113 = call "OP100 Indicators.vi"("error in (no error)"=w185, "Array"=w182, "OUTPUT INDICATOR"=w184) -> ("error out"=w176:errorcluster, "OUTPUT INDICATOR"=w181:T13)  [unwired: 7 in]
            n114 = call "PADMINI_AUTO_BARCODE_STRING 110.vi"("Enum"=enum16{"Read", "Write"}."Read", "error in (no error)"=w176) -> ("Input 2"=w178:string[])  [unwired: 8 in, 1 out]
            n115 = Index Array(array=w178) -> (element #1=w179:string, element #2=w172:string, element #3=w171:string)  [unwired: 3 in]
            n116 = Bundle By Name(cluster=w181, "OP - 110.BARCODE"=w179, "OP - 110.BIN\nNumber"=w172, "OP - 110.PALLET\nNumber"=w171) -> (w180:T13)
          }
          frame "SCAN1" {
            # "STATION OP 10"
            n117 = global read "Global 1.vi" "BARCODE RECIPE"() -> (w252:string)
            n118 = call "PADMINI_AUTO_BARCODE_STRING.vi"("Enum"=enum16{"Read", "Write"}."Read", "error in (no error)"=w261) -> ("error out"=w260:errorcluster, "Input 2"=w248:string[])  [unwired: 8 in]
            n119 = Index Array(array=w248) -> (element=w247:string)  [unwired: 1 in]
            n120 = call <vilib>:"Trim Whitespace.vi"("string"=w247) -> ("trimmed string"=w246:string)  [unwired: 1 in]
            n121 = Match Pattern(string=w246, regular expression=w252) -> (match substring=w255:string)  [unwired: 1 in, 3 out]
            n122 = String Length(string=w252) -> (length=w254:i32)
            n123 = String Length(string=w255) -> (length=w253:i32)
            n124 = Equal?(x=w254, y=w253) -> (x = y?=w259:bool)
            n125 = case shown="False" w258 {
              tunnel: w265 -> [w291 w309]
              tunnel: w260 -> [w290 w307]
              tunnel: w264 -> [w289 _]
              tunnel: [w288 w306] -> w250
              tunnel: [w287 w309] -> w263
              tunnel: w259 -> [_ _]
              tunnel: w246 -> [w286 _]
              tunnel: [w285 TRUE] -> w244
              frame False {
                n126 = Format Into String(format string="where BARCODE='%s'", w286) -> (resulting string=w282:string)  [unwired: 2 in, 1 out]
                n127 = call <vilib>:"DB Tools Select Data.vi"("condition"=w282, "error in (no error)"=w290, "columns"=string[] ["BARCODE", "OP10_FINAL_RESULT"], "table"=w289, "connection reference"=w291) -> ("error out"=w281:errorcluster, "data"=w280:variant[][], "connection reference out"=w287:T16)  [unwired: 1 in]
                n128 = call "PADMINI_varient_to_data.vi"("error in (no error)"=w281, "data"=w280) -> ("error out"=w278:errorcluster, "Array"=w274:string[][])  [unwired: 8 in]
                n129 = Index Array(array=w274, index (row)=0) -> (element=→"SCAN OP10":string[])  [unwired: 1 in]
                n130 = Index Array(array=w274, index (row)=0, index (col)=1 ("index (row)")) -> (element=w275:string)
                n131 = Empty Array?(array=w274) -> (empty?=w279:bool)
                n132 = case shown="False" w279 {
                  tunnel: w278 -> [w301 w303]
                  tunnel: [w300 w303] -> w288
                  tunnel: [FALSE TRUE] -> w285
                  tunnel: w275 -> [w295 _]
                  frame False {
                    w294 = "OK"  # y
                    w297 = i32[] [1, 0]  # I/P
                    w296 = i32[] [0, 1]  # I/P
                    # "OP10 CURRENT STATION OK-NG\nPART REPEAT"
                    n133 = Equal?(x=w295, y=w294) -> (x = y?=w293:bool)
                    n134 = Select(t=w297, s=w293, f=w296) -> (s? t:f=w292:i32[])
                    "OP10 STATUS" <- w292
                    n135 = call "PADMINI_AUTO_BARCODE_STATUS.vi"("Enum"=enum16{"Read", "Write"}."Write", "error in (no error)"=w301, "I/P"=w292) -> ("error out"=w300:errorcluster)  [unwired: 7 in, 1 out]
                  }
                  frame True {
                    # "OP10 NEW part"
                  }
                }
              }
              frame True {
                w305 = i32[] [0, 1]  # I/P
                n136 = call "PADMINI_AUTO_BARCODE_STATUS.vi"("Enum"=enum16{"Read", "Write"}."Write", "error in (no error)"=w307, "I/P"=w305) -> ("error out"=w306:errorcluster)  [unwired: 7 in, 1 out]
              }
            }
            n137 = flat-sequence {
              tunnel: [w271] -> w249
              tunnel: w250 -> [w271]
              frame #0 {
                # "UPDATE op 10 sCAN sTATUS"
                n138 = global write "DATA LOG.vi" "OP 10 Outputs"(TRUE) -> ()
              }
            }
            n139 = call <vilib>:"Clear Errors.vi"("error in (no error)"=w249) -> ("error out"=w243:errorcluster)  [unwired: 5 in, 1 out]
            n140 = case shown="True" w244 {
              tunnel: w245 -> [_ w269]
              tunnel: w243 -> [_ w267]
              frame False {
              }
              frame True {
                w268 = cluster{"CASE 2":T15} {"CASE 2"=enum."DATALOG1"}  # element
                n141 = Enqueue Element(queue=w269, element=w268, error in (no error)=w267) -> ()  [unwired: 1 in, 3 out]
              }
            }
          }
          frame "DATALOG1" {
            w324 = T17 2 items=["no dialog", "OK message", "continue or stop message", "OK message + warnings", "continue/stop + warnings"] ("type of dialog (OK msg:1)")
            # "cycle result status\nwhether it was ok or nok\nor abortted in between"
            # "Printed QR Code data string"
            # "datalog of OP 10"
            n142 = call "PADMINI_AUTO_BARCODE_STRING.vi"("Enum"=enum16{"Read", "Write"}."Read", "error in (no error)"=w310) -> ("Input 2"=w317:string[])  [unwired: 8 in, 1 out]
            n143 = call "PADMINI_AUTO_CYCLE VALUE 10.vi"("Enum"=enum16{"Read", "Write"}."Read", "error in (no error)"=w310) -> ("error out"=w313:errorcluster, "Input 2"=w312:sgl[])  [unwired: 8 in]
            n144 = Index Array(array=w312) -> (element=w311:sgl)  [unwired: 1 in]
            n145 = Index Array(array=w317) -> (element #1=w316:string, element #2=w315:string)  [unwired: 2 in]
            n146 = Number To Fractional String(number=w311, precision (6)=i16 2) -> (F-format string=w318:string)  [unwired: 2 in]
            n147 = call <vilib>:"Trim Whitespace.vi"("string"=w316) -> ("trimmed string"=w327:string)  [unwired: 1 in]
            n148 = case shown="False" w332 {
              tunnel: w333 -> [w357 w392]
              tunnel: w313 -> [w359 w391]
              tunnel: [w365 w390] -> w330
              tunnel: [w364 w389] -> w325
              tunnel: w331 -> [w354 _]
              tunnel: w327 -> [w351 _]
              tunnel: w315 -> [w361 w382]
              tunnel: w318 -> [w345 w381]
              frame False {
                w353 = string[] ["BARCODE", "SHIFT", "OP10_DATE", "OP10_LEAK_RATE_SCCM", "OP10_FINAL_RESULT"]
                # "ST1 RESULT"
                # "DO TRACEBILITY"
                n149 = local read "SHIFT"() -> (w363:string)
                n150 = Format Into String(format string="Where BARCODE='%s' ", w351) -> (resulting string=w346:string)  [unwired: 2 in, 1 out]
                n151 = call <vilib>:"DB Tools Select Data.vi"("condition"=w346, "error in (no error)"=w359, "columns"=w353, "table"=w354, "connection reference"=w357) -> ("error out"=w355:errorcluster, "data"=w358:variant[][], "connection reference out"=w356:T16)  [unwired: 1 in]
                n152 = call "PADMINI_SHIFT_DATE.vi"("SHIFT"=w363) -> ("date/time string"=w362:string)  [unwired: 10 in]
                n153 = Variant To Data(error in=w355, type=string[][] [], Variant=w358) -> (data=w349:string[][], error out=w347:errorcluster)
                n154 = Bundle("trimmed string"=w351, "SHIFT"=w363, "date/time string"=w362, w345, "Input 2"=w361) -> (w360:T18)  [unwired: 1 in]
                n155 = Empty Array?(array=w349) -> (empty?=w348:bool)
                n156 = case shown="False" w348 {
                  tunnel: w356 -> [w370 w380]
                  tunnel: w347 -> [w369 w379]
                  tunnel: [w373 w378] -> w365
                  tunnel: [w372 w377] -> w364
                  tunnel: w353 -> [w367 w376]
                  tunnel: w354 -> [w368 w375]
                  tunnel: w360 -> [w371 w374]
                  tunnel: w346 -> [w366 _]
                  frame False {
                    n157 = call <vilib>:"DB Tools Update Data.vi"("condition"=w366, "data"=w371, "error in (no error)"=w369, "columns"=w367, "table"=w368, "connection reference"=w370) -> ("error out"=w372:errorcluster, "connection reference out"=w373:T16)  [unwired: 4 in]
                  }
                  frame True {
                    n158 = call <vilib>:"DB Tools Insert Data.vi"("data"=w374, "error in (no error)"=w379, "columns"=w376, "table"=w375, "connection reference"=w380) -> ("error out"=w377:errorcluster, "connection reference out"=w378:T16)  [unwired: 5 in]
                  }
                }
              }
              frame True {
                # "Trac BYPASS"
                n159 = local read "SHIFT"() -> (w387:string)
                n160 = call "PADMINI_SHIFT_DATE.vi"("SHIFT"=w387) -> ("date/time string"=w386:string)  [unwired: 10 in]
                n161 = Bundle("SHIFT"=w387, "date/time string"=w386, "Input 2"=w382, w381) -> (w385:T19)  [unwired: 1 in]
                n162 = To Variant(anything=w385) -> (Variant=w384:variant)
                n163 = call <vilib>:"DB Tools Insert Data.vi"("data"=w384, "error in (no error)"=w391, "columns"=string[] ["DATE", "SHIFT", "OP10_LEAK_RAT", "OP10_FINAL_RST"], "table"="ST1_REPORT", "connection reference"=w392) -> ("error out"=w389:errorcluster, "connection reference out"=w390:T16)  [unwired: 5 in]
              }
            }
            n164 = call <vilib>:"Simple Error Handler.vi"("type of dialog (OK msg:1)"=w324, "error in (no error)"=w325) -> ("error out"=w323:errorcluster)  [unwired: 3 in, 4 out]
            n165 = call <vilib>:"Clear Errors.vi"("error in (no error)"=w323) -> ("error out"=w321:errorcluster)  [unwired: 5 in, 1 out]
            n166 = disable-structure shown="Enabled" {
              disable-tunnel: [w343 w344] -> w329
              disable-tunnel: w321 -> [w342 w344]
              frame Disabled {
                w337 = refnum<vi> refnum  # Boolean
                n167 = property on="OP - 10" class="Clust"(error in=w342) -> (error out=w336:errorcluster, "Controls[]"=w340:refnum<vi>[])  [unwired: 1 in, 1 out]
                n168 = Index Array(array=w340, index=2) -> (element=w338:refnum<vi>)
                n169 = To More Specific Class(target class=w337, reference=w338, error in=w336) -> (specific class reference=w341:refnum<vi>, error out=w335:errorcluster)
                n170 = call "PADMINI_BOOL_COLOR_CHANGE.vi"("error in (no error)"=w335, "Boolean in"=w341) -> ("error out"=w343:errorcluster)  [unwired: 9 in]
              }
              frame Enabled {
              }
            }
          }
          frame "SCAN2" {
            # "Barcode Status\n0-Ideal, 1-Ok, 2-Nok, 3-Prev Station Not Done,\n4-Prev Station Nok,\n5- Already Done"
            # "STATION OP 20"
            n171 = case shown="False" w399 {
              tunnel: w403 -> [w428 w434]
              tunnel: w402 -> [w421 w432]
              tunnel: w401 -> [w409 _]
              tunnel: [w423 w431] -> w398
              tunnel: [w422 w434] -> w400
              tunnel: [w410 "" ("trimmed string")] -> _
              frame False {
                # "ST2 RESULT"
                # "ST1 RESULT"
                # "2 FOR EMPTY BARCODE READ OR MISMATCH"
                n172 = call "PADMINI_AUTO_BARCODE_STRING2.vi"("Enum"=enum16{"Read", "Write"}."Read", "error in (no error)"=w421) -> ("error out"=w420:errorcluster, "Input 2"=w412:string[])  [unwired: 8 in]
                n173 = global read "Global 1.vi" "BARCODE RECIPE"() -> (w413:string)
                n174 = Index Array(array=w412) -> (element=w411:string)  [unwired: 1 in]
                n175 = call <vilib>:"Trim Whitespace.vi"("string"=w411) -> ("trimmed string"=w410:string)  [unwired: 1 in]
                n176 = Match Pattern(string=w410, regular expression=w413) -> (match substring=w414:string)  [unwired: 1 in, 3 out]
                n177 = String Length(string=w413) -> (length=w416:i32)
                n178 = String Length(string=w414) -> (length=w415:i32)
                n179 = Format Into String(format string="WHERE BARCODE  ='%s'", w410) -> (resulting string=w417:string)  [unwired: 2 in, 1 out]
                n180 = Equal?(x=w416, y=w415) -> ()  [unwired: 1 out]
                n181 = call <vilib>:"DB Tools Select Data.vi"("condition"=w417, "error in (no error)"=w420, "columns"=string[] ["BARCODE", "OP10_FINAL_RESULT", "OP20_FINAL_RESULT"], "table"=w409, "connection reference"=w428) -> ("error out"=w426:errorcluster, "data"=w425:variant[][], "connection reference out"=w422:T16)  [unwired: 1 in]
                n182 = call "PADMINI_varient_to_data.vi"("error in (no error)"=w426, "data"=w425) -> ("error out"=w424:errorcluster, "Array"=w406:string[][])  [unwired: 8 in]
                n183 = Index Array(array=w406, index (row)=0 ("disabled index (col)")) -> (element=→"SCAN OP20":string[])  [unwired: 1 in]
                n184 = call "RESPONSE_LOGIC.vi"("Array"=w406) -> ("Not Found"=w404:i32[])  [unwired: 10 in]
                "OP20 STATUS" <- w404
                n185 = call "PADMINI_AUTO_BARCODE_STATUS 20.vi"("Enum"=enum16{"Read", "Write"}."Write", "error in (no error)"=w424, "I/P"=w404) -> ("error out"=w423:errorcluster)  [unwired: 7 in, 1 out]
              }
              frame True {
                w429 = i32[] [0, 0, 0, 0, 0]  # I/P
                n186 = call "PADMINI_AUTO_BARCODE_STATUS 20.vi"("Enum"=enum16{"Read", "Write"}."Write", "error in (no error)"=w432, "I/P"=w429) -> ("error out"=w431:errorcluster)  [unwired: 7 in, 1 out]
              }
            }
            n187 = flat-sequence {
              tunnel: [w436] -> w397
              tunnel: w398 -> [w436]
              frame #0 {
                # "UPDATE op 20 SCAN sTATUS"
                n188 = global write "DATA LOG.vi" "OP 20 Outputs"(TRUE) -> ()
              }
            }
          }
          frame "DATALOG2" {
            (unwired) string[] ["OP20_DATE", "OP20_LOWER_BEARING_DIS", "OP20_LOWER_BEARING_LOAD", "OP20_UPPER_BEARING_DIS", "OP20_UPPER_BEARING_LOAD", "OP20_LOWER_BEARING_RST", "OP20_BOTTOM_CAMERA_STATUS", "OP20_UPPER_SIM_STATUS", "OP20_UPPER_BERAING_RST", "OP20_UPPER_CAMERA_STATUS", "OP20_FINAL_RST"]
            w450 = T17 2 items=["no dialog", "OK message", "continue or stop message", "OK message + warnings", "continue/stop + warnings"] ("type of dialog (OK msg:1)")
            # "Printed QR Code data string"
            # "datalog of OP 20"
            n189 = call "PADMINI_AUTO_BARCODE_STRING2.vi"("Enum"=enum16{"Read", "Write"}."Read", "error in (no error)"=w443) -> ("error out"=w445:errorcluster, "Input 2"=w439:string[])  [unwired: 8 in]
            n190 = call "PADMINI_AUTO_CYCLE VALUE 20.vi"("Enum"=enum16{"Read", "Write"}."Read", "error in (no error)"=w443) -> ("Input 2"=w441:sgl[])  [unwired: 8 in, 1 out]
            n191 = Number To Fractional String(number=w441, precision (6)=i16 2) -> (F-format string=w440:string[])  [unwired: 2 in]
            n192 = case shown="False" w455 {
              tunnel: w456 -> [w480 w506]
              tunnel: w445 -> [w481 w505]
              tunnel: [w484 w504] -> w453
              tunnel: [w483 w503] -> w451
              tunnel: w454 -> [w479 _]
              tunnel: w440 -> [w476 w488]
              tunnel: w439 -> [w470 w489]
              frame False {
                # "ST2 RESULT"
                # "DO TRACEBILITY"
                n193 = Index Array(array=w470) -> (element #1=w471:string, element #2=w466:string, element #3=w465:string, element #4=w464:string, element #5=w463:string, element #6=w462:string, element #7=w461:string)  [unwired: 7 in]
                n194 = local read "SHIFT"() -> (w482:string)
                n195 = Index Array(array=w476) -> (element #1=w475:string, element #2=w474:string, element #3=w468:string, element #4=w467:string)  [unwired: 4 in]
                n196 = call <vilib>:"Trim Whitespace.vi"("string"=w471) -> ("trimmed string"=w472:string)  [unwired: 1 in]
                n197 = call "PADMINI_SHIFT_DATE.vi"("SHIFT"=w482) -> ("date/time string"=w469:string)  [unwired: 10 in]
                n198 = Format Into String(format string="Where BARCODE='%s' ", w472) -> (resulting string=w477:string)  [unwired: 2 in, 1 out]
                n199 = Bundle("date/time string"=w469, "Input 2"=w475, "Input 2"=w474, "Input 2"=w468, "Input 2"=w467, "Input 2"=w466, "Input 2"=w465, "Input 2"=w464, "Input 2"=w463, "Input 2"=w462, "Input 2"=w461) -> (w473:T20)  [unwired: 1 in]
                n200 = call <vilib>:"DB Tools Update Data.vi"("condition"=w477, "data"=w473, "error in (no error)"=w481, "columns"=string[] ["OP20_DATE", "OP20_BOTTOM_DISPLACE_mm", "OP20_BOTTOM_LOAD_kg", "OP20_TOP_DISPLACE_mm", "OP20_TOP_LOAD_kg", "OP20_BOTTOM_RESULT", "OP20_BOTTOM_CAMERA_STATUS", "OP20_TOP_SIM_STATUS", "OP20_TOP_RESULT", "OP20_TOP_CAMERA_STATUS", "OP20_FINAL_RESULT"], "table"=w479, "connection reference"=w480) -> ("error out"=w483:errorcluster, "connection reference out"=w484:T16)  [unwired: 4 in]
              }
              frame True {
                n201 = local read "SHIFT"() -> (w486:string)
                n202 = Index Array(array=w489) -> (element #2=w495:string, element #3=w494:string, element #4=w493:string, element #5=w492:string, element #6=w491:string, element #7=w485:string)  [unwired: 7 in, 1 out]
                n203 = call "PADMINI_SHIFT_DATE.vi"("SHIFT"=w486) -> ("date/time string"=w487:string)  [unwired: 10 in]
                n204 = Index Array(array=w488) -> (element #1=w499:string, element #2=w498:string, element #3=w497:string, element #4=w496:string)  [unwired: 4 in]
                n205 = Bundle("date/time string"=w487, "SHIFT"=w486, "Input 2"=w499, "Input 2"=w498, "Input 2"=w495, "Input 2"=w494, "Input 2"=w497, "Input 2"=w496, "Input 2"=w493, "Input 2"=w492, "Input 2"=w491, "Input 2"=w485) -> (w490:T21)  [unwired: 1 in]
                n206 = To Variant(anything=w490) -> (Variant=w501:variant)
                n207 = call <vilib>:"DB Tools Insert Data.vi"("data"=w501, "error in (no error)"=w505, "columns"=string[] ["DATE", "SHIFT", "ST2_LOWER_BEARING_DIS", "ST2_LOWER_BEARING_LOAD", "ST2_BOTTOM_CAMERA_STATUS", "ST2_LOWER_BEARING_RST", "ST2_UPPER_BEARING_DIS", "ST2_UPPER_BEARING_LOAD", "ST2_UPPER_SIM_STATUS", "ST2_UPPER_CAMERA_STATUS", "ST2_UPPER_BERAING_RST", "ST2_FINAL_RST"], "table"="ST2_REPORT", "connection reference"=w506) -> ("error out"=w503:errorcluster, "connection reference out"=w504:T16)  [unwired: 5 in]
              }
            }
            n208 = call <vilib>:"Simple Error Handler.vi"("type of dialog (OK msg:1)"=w450, "error in (no error)"=w451) -> ("error out"=w449:errorcluster)  [unwired: 3 in, 4 out]
            n209 = call <vilib>:"Clear Errors.vi"("error in (no error)"=w449) -> ("error out"=w447:errorcluster)  [unwired: 5 in, 1 out]
            n210 = flat-sequence {
              tunnel: [w459] -> w438
              tunnel: w447 -> [w459]
              frame #0 {
                # "UPDATE op 20 save"
                n211 = global write "DATA LOG.vi" "OP 20 reset"(TRUE) -> ()
              }
            }
          }
          frame "SCAN3" {
            # "STATION OP 30"
            n212 = case shown="False" w513 {
              tunnel: w517 -> [w543 w549]
              tunnel: w516 -> [w536 w547]
              tunnel: w515 -> [w523 _]
              tunnel: [w538 w546] -> w512
              tunnel: [w537 w549] -> w514
              tunnel: [w524 "" ("trimmed string")] -> _
              frame False {
                n213 = call "PADMINI_AUTO_BARCODE_STRING 30.vi"("Enum"=enum16{"Read", "Write"}."Read", "error in (no error)"=w536) -> ("error out"=w535:errorcluster, "Input 2"=w526:string[])  [unwired: 8 in]
                n214 = global read "Global 1.vi" "BARCODE RECIPE"() -> (w527:string)
                n215 = Index Array(array=w526) -> (element=w525:string)  [unwired: 1 in]
                n216 = call <vilib>:"Trim Whitespace.vi"("string"=w525) -> ("trimmed string"=w524:string)  [unwired: 1 in]
                n217 = Match Pattern(string=w524, regular expression=w527) -> (match substring=w528:string)  [unwired: 1 in, 3 out]
                n218 = String Length(string=w527) -> (length=w530:i32)
                n219 = String Length(string=w528) -> (length=w529:i32)
                n220 = Equal?(x=w524, y="") -> ()  [unwired: 1 out]
                n221 = Format Into String(format string="WHERE BARCODE  ='%s'", w524) -> (resulting string=w532:string)  [unwired: 2 in, 1 out]
                n222 = Equal?(x=w530, y=w529) -> ()  [unwired: 1 out]
                n223 = call <vilib>:"DB Tools Select Data.vi"("condition"=w532, "error in (no error)"=w535, "columns"=string[] ["BARCODE", "OP20_FINAL_RESULT", "OP30_FINAL_RESULT"], "table"=w523, "connection reference"=w543) -> ("error out"=w541:errorcluster, "data"=w540:variant[][], "connection reference out"=w537:T16)  [unwired: 1 in]
                n224 = call "PADMINI_varient_to_data.vi"("error in (no error)"=w541, "data"=w540) -> ("error out"=w539:errorcluster, "Array"=w520:string[][])  [unwired: 8 in]
                n225 = Index Array(array=w520, index (row)=0 ("disabled index (col)")) -> (element=→"SCAN OP30":string[])  [unwired: 1 in]
                n226 = call "RESPONSE_LOGIC.vi"("Array"=w520) -> ("Not Found"=w518:i32[])  [unwired: 10 in]
                "OP30 STATUS" <- w518
                n227 = call "PADMINI_AUTO_BARCODE_STATUS 30.vi"("Enum"=enum16{"Read", "Write"}."Write", "error in (no error)"=w539, "I/P"=w518) -> ("error out"=w538:errorcluster)  [unwired: 7 in, 1 out]
              }
              frame True {
                w544 = i32[] [0, 0, 0, 0, 0]  # I/P
                n228 = call "PADMINI_AUTO_BARCODE_STATUS 30.vi"("Enum"=enum16{"Read", "Write"}."Write", "error in (no error)"=w547, "I/P"=w544) -> ("error out"=w546:errorcluster)  [unwired: 7 in, 1 out]
              }
            }
            n229 = flat-sequence {
              tunnel: [w551] -> w511
              tunnel: w512 -> [w551]
              frame #0 {
                # "UPDATE op 30 SCAN sTATUS"
                n230 = global write "DATA LOG.vi" "OP 30 Outputs"(TRUE) -> ()
              }
            }
          }
          frame "DATALOG3" {
            (unwired) string[] ["OP30_DATE", "OP30_DISPLACEMENT", "OP30_SHAFT_PRESS_LOAD", "OP30_SHAFT_STATUS", "OP30_FINAL_RST"]
            w565 = T17 2 items=["no dialog", "OK message", "continue or stop message", "OK message + warnings", "continue/stop + warnings"] ("type of dialog (OK msg:1)")
            # "Printed QR Code data string"
            # "datalog of OP 30"
            n231 = call "PADMINI_AUTO_BARCODE_STRING 30.vi"("Enum"=enum16{"Read", "Write"}."Read", "error in (no error)"=w557) -> ("error out"=w559:errorcluster, "Input 2"=w553:string[])  [unwired: 8 in]
            n232 = call "PADMINI_AUTO_CYCLE VALUE 30.vi"("Enum"=enum16{"Read", "Write"}."Read", "error in (no error)"=w557) -> ("Input 2"=w555:sgl[])  [unwired: 8 in, 1 out]
            n233 = Number To Fractional String(number=w555, precision (6)=i16 2) -> (F-format string=w554:string[])  [unwired: 2 in]
            n234 = case shown="False" w570 {
              tunnel: w571 -> [w589 w609]
              tunnel: w559 -> [w590 w608]
              tunnel: [w593 w607] -> w568
              tunnel: [w592 w606] -> w566
              tunnel: w569 -> [w588 _]
              tunnel: w554 -> [w585 w594]
              tunnel: w553 -> [w579 w595]
              frame False {
                # "DO TRACEBILITY"
                n235 = Index Array(array=w579) -> (element #1=w580:string, element #2=w578:string, element #3=w577:string)  [unwired: 3 in]
                n236 = local read "SHIFT"() -> (w591:string)
                n237 = Index Array(array=w585) -> (element #1=w584:string, element #2=w583:string)  [unwired: 2 in]
                n238 = call <vilib>:"Trim Whitespace.vi"("string"=w580) -> ("trimmed string"=w581:string)  [unwired: 1 in]
                n239 = call "PADMINI_SHIFT_DATE.vi"("SHIFT"=w591) -> ("date/time string"=w576:string)  [unwired: 10 in]
                n240 = Format Into String(format string="Where BARCODE='%s' ", w581) -> (resulting string=w586:string)  [unwired: 2 in, 1 out]
                n241 = Bundle("date/time string"=w576, "Input 2"=w584, "Input 2"=w583, "Input 2"=w578, "Input 2"=w577) -> (w582:T22)  [unwired: 1 in]
                n242 = call <vilib>:"DB Tools Update Data.vi"("condition"=w586, "data"=w582, "error in (no error)"=w590, "columns"=string[] ["OP30_DATE", "OP30_DISPLACEMENT_mm", "OP30_SHAFT_PRESS_LOAD_kg", "OP30_SHAFT_STATUS", "OP30_FINAL_RESULT"], "table"=w588, "connection reference"=w589) -> ("error out"=w592:errorcluster, "connection reference out"=w593:T16)  [unwired: 4 in]
              }
              frame True {
                # "TRAC BYPASS"
                n243 = local read "SHIFT"() -> (w596:string)
                n244 = call "PADMINI_SHIFT_DATE.vi"("SHIFT"=w596) -> ("date/time string"=w597:string)  [unwired: 10 in]
                n245 = Index Array(array=w595) -> (element #2=w601:string, element #3=w600:string)  [unwired: 3 in, 1 out]
                n246 = Index Array(array=w594) -> (element #1=w603:string, element #2=w602:string)  [unwired: 2 in]
                n247 = Bundle("date/time string"=w597, "SHIFT"=w596, "Input 2"=w603, "Input 2"=w602, "Input 2"=w601, "Input 2"=w600) -> (w598:T23)  [unwired: 1 in]
                n248 = To Variant(anything=w598) -> (Variant=w599:variant)
                n249 = call <vilib>:"DB Tools Insert Data.vi"("data"=w599, "error in (no error)"=w608, "columns"=string[] ["DATE", "SHIFT", "ST3_DISPLACEMENT", "ST3_LOAD", "ST3_MIDDLE_GEAR_SHAFT_STATUS", "ST3_FINAL_RST"], "table"="ST3_REPORT", "connection reference"=w609) -> ("error out"=w606:errorcluster, "connection reference out"=w607:T16)  [unwired: 5 in]
              }
            }
            n250 = call <vilib>:"Simple Error Handler.vi"("type of dialog (OK msg:1)"=w565, "error in (no error)"=w566) -> ("error out"=w564:errorcluster)  [unwired: 3 in, 4 out]
            n251 = call <vilib>:"Clear Errors.vi"("error in (no error)"=w564) -> ("error out"=w562:errorcluster)  [unwired: 5 in, 1 out]
            n252 = flat-sequence {
              tunnel: [w574] -> w552
              tunnel: w562 -> [w574]
              frame #0 {
                # "UPDATE op 20 save"
                n253 = global write "DATA LOG.vi" "OP 30 reset"(TRUE) -> ()
              }
            }
          }
          frame "SCAN4" {
            # "STATION OP 40"
            n254 = case shown="False" w616 {
              tunnel: w620 -> [w641 w647]
              tunnel: w619 -> [w634 w646]
              tunnel: w618 -> [w626 _]
              tunnel: [w636 w645] -> w615
              tunnel: [w635 w647] -> w617
              tunnel: [w627 "" ("trimmed string")] -> _
              frame False {
                n255 = call "PADMINI_AUTO_BARCODE_STRING 40.vi"("Enum"=enum16{"Read", "Write"}."Read", "error in (no error)"=w634) -> ("error out"=w633:errorcluster, "Input 2"=w629:string[])  [unwired: 8 in]
                n256 = Index Array(array=w629) -> (element=w628:string)  [unwired: 1 in]
                n257 = call <vilib>:"Trim Whitespace.vi"("string"=w628) -> ("trimmed string"=w627:string)  [unwired: 1 in]
                n258 = Format Into String(format string="WHERE BARCODE  ='%s'", w627) -> (resulting string=w630:string)  [unwired: 2 in, 1 out]
                n259 = call <vilib>:"DB Tools Select Data.vi"("condition"=w630, "error in (no error)"=w633, "columns"=string[] ["BARCODE", "OP30_FINAL_RESULT", "OP40_FINAL_RESULT"], "table"=w626, "connection reference"=w641) -> ("error out"=w639:errorcluster, "data"=w638:variant[][], "connection reference out"=w635:T16)  [unwired: 1 in]
                n260 = call "PADMINI_varient_to_data.vi"("error in (no error)"=w639, "data"=w638) -> ("error out"=w637:errorcluster, "Array"=w623:string[][])  [unwired: 8 in]
                n261 = call "RESPONSE_LOGIC.vi"("Array"=w623) -> ("Not Found"=w621:i32[])  [unwired: 10 in]
                "OP40 STATUS" <- w621
                n262 = Index Array(array=w623, index (row)=0 ("disabled index (col)")) -> (element=→"SCAN OP40":string[])  [unwired: 1 in]
                n263 = call "PADMINI_AUTO_BARCODE_STATUS 40.vi"("Enum"=enum16{"Read", "Write"}."Write", "error in (no error)"=w637, "I/P"=w621) -> ("error out"=w636:errorcluster)  [unwired: 7 in, 1 out]
              }
              frame True {
                w642 = i32[] [0, 0, 0, 0, 0]  # I/P
                n264 = call "PADMINI_AUTO_BARCODE_STATUS 40.vi"("Enum"=enum16{"Read", "Write"}."Write", "error in (no error)"=w646, "I/P"=w642) -> ("error out"=w645:errorcluster)  [unwired: 7 in, 1 out]
              }
            }
            n265 = flat-sequence {
              tunnel: [w649] -> w614
              tunnel: w615 -> [w649]
              frame #0 {
                # "UPDATE op 40 SCAN sTATUS"
                n266 = global write "DATA LOG.vi" "OP 40 Outputs"(TRUE) -> ()
              }
            }
          }
          frame "DATALOG4" {
            w663 = T17 2 items=["no dialog", "OK message", "continue or stop message", "OK message + warnings", "continue/stop + warnings"] ("type of dialog (OK msg:1)")
            # "datalog of OP 40"
            n267 = call "PADMINI_AUTO_BARCODE_STRING 40.vi"("Enum"=enum16{"Read", "Write"}."Read", "error in (no error)"=w655) -> ("error out"=w657:errorcluster, "Input 2"=w651:string[])  [unwired: 8 in]
            n268 = call "PADMINI_AUTO_CYCLE VALUE 40.vi"("Enum"=enum16{"Read", "Write"}."Read", "error in (no error)"=w655) -> ("Input 2"=w653:sgl[])  [unwired: 8 in, 1 out]
            n269 = Number To Fractional String(number=w653, precision (6)=i16 2) -> (F-format string=w652:string[])  [unwired: 2 in]
            n270 = case shown="False" w668 {
              tunnel: w669 -> [w691 w715]
              tunnel: w657 -> [w692 w714]
              tunnel: [w695 w713] -> w666
              tunnel: [w694 w712] -> w664
              tunnel: w667 -> [w690 _]
              tunnel: w652 -> [w686 w697]
              tunnel: w651 -> [w681 w696]
              frame False {
                # "DO TRACEBILITY"
                n271 = Index Array(array=w681) -> (element #1=w682:string, element #2=w677:string, element #3=w676:string, element #4=w674:string, element #5=w673:string)  [unwired: 5 in]
                n272 = local read "SHIFT"() -> (w693:string)
                n273 = Index Array(array=w686) -> (element #1=w685:string, element #2=w680:string, element #3=w679:string, element #4=w678:string)  [unwired: 4 in]
                n274 = call <vilib>:"Trim Whitespace.vi"("string"=w682) -> ("trimmed string"=w683:string)  [unwired: 1 in]
                n275 = call "PADMINI_SHIFT_DATE.vi"("SHIFT"=w693) -> ("date/time string"=w675:string)  [unwired: 10 in]
                n276 = Format Into String(format string="Where BARCODE='%s' ", w683) -> (resulting string=w688:string)  [unwired: 2 in, 1 out]
                n277 = Bundle("date/time string"=w675, "Input 2"=w685, "Input 2"=w677, "Input 2"=w680, "Input 2"=w676, "Input 2"=w679, "Input 2"=w678, "Input 2"=w674, "Input 2"=w673) -> (w684:T24)  [unwired: 1 in]
                n278 = call <vilib>:"DB Tools Update Data.vi"("condition"=w688, "data"=w684, "error in (no error)"=w692, "columns"=string[] ["OP40_DATE", "OP40_RH_SCREW_Nm", "OP40_RH_STATUS", "OP40_LH_SCREW_Nm", "OP40_LH_STATUS", "OP40_DISPLACEMENT_mm", "OP40_STACK_LOAD_kg", "OP40_TOP_BEARING_CAMERA_STAUS", "OP40_FINAL_RESULT"], "table"=w690, "connection reference"=w691) -> ("error out"=w694:errorcluster, "connection reference out"=w695:T16)  [unwired: 4 in]
              }
              frame True {
                # "TRAC BYPASS"
                n279 = local read "SHIFT"() -> (w698:string)
                n280 = Index Array(array=w696) -> (element #2=w706:string, element #3=w705:string, element #4=w704:string, element #5=w703:string)  [unwired: 5 in, 1 out]
                n281 = call "PADMINI_SHIFT_DATE.vi"("SHIFT"=w698) -> ("date/time string"=w699:string)  [unwired: 10 in]
                n282 = Index Array(array=w697) -> (element #1=w700:string, element #2=w709:string, element #3=w708:string, element #4=w707:string)  [unwired: 4 in]
                n283 = Bundle("date/time string"=w699, "SHIFT"=w698, "Input 2"=w700, "Input 2"=w706, "Input 2"=w709, "Input 2"=w705, "Input 2"=w708, "Input 2"=w707, "Input 2"=w703, "Input 2"=w704) -> (w702:T25)  [unwired: 1 in]
                n284 = To Variant(anything=w702) -> (Variant=w701:variant)
                n285 = call <vilib>:"DB Tools Insert Data.vi"("data"=w701, "error in (no error)"=w714, "columns"=string[] ["DATE", "SHIFT", "ST4_SCREW1_DATA", "ST4_SCREW1_STATUS", "ST4_SCREW2_DATA", "ST4_SCREW2_STATUS", "ST4_DISPLACEMENT", "ST4_LOAD", "ST4_TOP_BEARING_CAMERA_STAUS", "ST4_FINAL_RST"], "table"="ST4_REPORT", "connection reference"=w715) -> ("error out"=w712:errorcluster, "connection reference out"=w713:T16)  [unwired: 5 in]
              }
            }
            n286 = call <vilib>:"Simple Error Handler.vi"("type of dialog (OK msg:1)"=w663, "error in (no error)"=w664) -> ("error out"=w662:errorcluster)  [unwired: 3 in, 4 out]
            n287 = call <vilib>:"Clear Errors.vi"("error in (no error)"=w662) -> ("error out"=w660:errorcluster)  [unwired: 5 in, 1 out]
            n288 = flat-sequence {
              tunnel: [w672] -> w650
              tunnel: w660 -> [w672]
              frame #0 {
                # "UPDATE op 20 save"
                n289 = global write "DATA LOG.vi" "OP 40 reset"(TRUE) -> ()
              }
            }
          }
          frame "SCAN5" {
            # "STATION OP 50"
            n290 = case shown="False" w722 {
              tunnel: w726 -> [w747 w753]
              tunnel: w725 -> [w740 w752]
              tunnel: w724 -> [w732 _]
              tunnel: [w742 w751] -> w721
              tunnel: [w741 w753] -> w723
              tunnel: [w733 "" ("trimmed string")] -> _
              frame False {
                n291 = call "PADMINI_AUTO_BARCODE_STRING 50.vi"("Enum"=enum16{"Read", "Write"}."Read", "error in (no error)"=w740) -> ("error out"=w739:errorcluster, "Input 2"=w735:string[])  [unwired: 8 in]
                n292 = Index Array(array=w735) -> (element=w734:string)  [unwired: 1 in]
                n293 = call <vilib>:"Trim Whitespace.vi"("string"=w734) -> ("trimmed string"=w733:string)  [unwired: 1 in]
                n294 = Format Into String(format string="WHERE BARCODE  ='%s'", w733) -> (resulting string=w736:string)  [unwired: 2 in, 1 out]
                n295 = call <vilib>:"DB Tools Select Data.vi"("condition"=w736, "error in (no error)"=w739, "columns"=string[] ["BARCODE", "OP40_FINAL_RESULT", "OP50_FINAL_RESULT"], "table"=w732, "connection reference"=w747) -> ("error out"=w745:errorcluster, "data"=w744:variant[][], "connection reference out"=w741:T16)  [unwired: 1 in]
                n296 = call "PADMINI_varient_to_data.vi"("error in (no error)"=w745, "data"=w744) -> ("error out"=w743:errorcluster, "Array"=w729:string[][])  [unwired: 8 in]
                n297 = Index Array(array=w729, index (row)=0 ("disabled index (col)")) -> (element=→"SCAN OP50":string[])  [unwired: 1 in]
                n298 = call "RESPONSE_LOGIC.vi"("Array"=w729) -> ("Not Found"=w728:i32[])  [unwired: 10 in]
                "OP50 STATUS" <- w728
                n299 = call "PADMINI_AUTO_BARCODE_STATUS 50.vi"("Enum"=enum16{"Read", "Write"}."Write", "error in (no error)"=w743, "I/P"=w728) -> ("error out"=w742:errorcluster)  [unwired: 7 in, 1 out]
              }
              frame True {
                w748 = i32[] [0, 0, 0, 0, 0]  # I/P
                n300 = call "PADMINI_AUTO_BARCODE_STATUS 50.vi"("Enum"=enum16{"Read", "Write"}."Write", "error in (no error)"=w752, "I/P"=w748) -> ("error out"=w751:errorcluster)  [unwired: 7 in, 1 out]
              }
            }
            n301 = flat-sequence {
              tunnel: [w755] -> w720
              tunnel: w721 -> [w755]
              frame #0 {
                # "UPDATE op 50 SCAN sTATUS"
                n302 = global write "DATA LOG.vi" "OP 50 Outputs"(TRUE) -> ()
              }
            }
          }
          frame "DATALOG5" {
            (unwired) string[] ["OP50_DATE", "OP50_NUT_TORQUE_Nm", "OP50_NUT_STATUS", "OP50_LH_MOTOR_SCREW_Nm", "OP50_LH_STATUS", "OP50_RH_MOTOR_SCREW_Nm", "OP50_RH_STATUS", "OP50_CAMERA_STATUS", "OP50_FINAL_RESULT"]
            w769 = T17 2 items=["no dialog", "OK message", "continue or stop message", "OK message + warnings", "continue/stop + warnings"] ("type of dialog (OK msg:1)")
            # "datalog of OP 50"
            n303 = call "PADMINI_AUTO_BARCODE_STRING 50.vi"("Enum"=enum16{"Read", "Write"}."Read", "error in (no error)"=w762) -> ("error out"=w764:errorcluster, "Input 2"=w758:string[])  [unwired: 8 in]
            n304 = call "PADMINI_AUTO_CYCLE VALUE 50.vi"("Enum"=enum16{"Read", "Write"}."Read", "error in (no error)"=w762) -> ("Input 2"=w760:sgl[])  [unwired: 8 in, 1 out]
            n305 = Number To Fractional String(number=w760, precision (6)=i16 2) -> (F-format string=w759:string[])  [unwired: 2 in]
            n306 = case shown="False" w774 {
              tunnel: w775 -> [w797 w819]
              tunnel: w764 -> [w798 w818]
              tunnel: [w801 w817] -> w772
              tunnel: [w800 w816] -> w770
              tunnel: w773 -> [w796 _]
              tunnel: w759 -> [w793 w803]
              tunnel: w758 -> [w789 w802]
              frame False {
                # "DO TRACEBILITY"
                n307 = Index Array(array=w789) -> (element #1=w790:string, element #2=w785:string, element #3=w783:string, element #4=w781:string, element #5=w780:string, element #6=w779:string)  [unwired: 6 in]
                n308 = local read "SHIFT"() -> (w799:string)
                n309 = Index Array(array=w793) -> (element #1=w786:string, element #2=w784:string, element #3=w782:string)  [unwired: 3 in]
                n310 = call <vilib>:"Trim Whitespace.vi"("string"=w790) -> ("trimmed string"=w791:string)  [unwired: 1 in]
                n311 = call "PADMINI_SHIFT_DATE.vi"("SHIFT"=w799) -> ("date/time string"=w788:string)  [unwired: 10 in]
                n312 = Format Into String(format string="Where BARCODE='%s' ", w791) -> (resulting string=w794:string)  [unwired: 2 in, 1 out]
                n313 = Bundle("date/time string"=w788, "Input 2"=w786, "Input 2"=w785, "Input 2"=w784, "Input 2"=w783, "Input 2"=w782, "Input 2"=w781, "Input 2"=w780, "Input 2"=w779) -> (w792:T24)  [unwired: 1 in]
                n314 = call <vilib>:"DB Tools Update Data.vi"("condition"=w794, "data"=w792, "error in (no error)"=w798, "columns"=string[] ["OP50_DATE", "OP50_NUT_TORQUE_Nm", "OP50_NUT_STATUS", "OP50_RH_MOTOR_SCREW_Nm", "OP50_RH_STATUS", "OP50_LH_MOTOR_SCREW_Nm", "OP50_LH_STATUS", "OP50_CAMERA_STATUS", "OP50_FINAL_RESULT"], "table"=w796, "connection reference"=w797) -> ("error out"=w800:errorcluster, "connection reference out"=w801:T16)  [unwired: 4 in]
              }
              frame True {
                # "TRAC BYPASS"
                n315 = local read "SHIFT"() -> (w804:string)
                n316 = Index Array(array=w802) -> (element #2=w808:string, element #3=w807:string, element #4=w812:string)  [unwired: 4 in, 1 out]
                n317 = Index Array(array=w803) -> (element #1=w811:string, element #2=w810:string, element #3=w809:string)  [unwired: 3 in]
                n318 = call "PADMINI_SHIFT_DATE.vi"("SHIFT"=w804) -> ("date/time string"=w805:string)  [unwired: 10 in]
                n319 = Bundle("date/time string"=w805, "SHIFT"=w804, "Input 2"=w811, "Input 2"=w808, "Input 2"=w810, "Input 2"=w807, "Input 2"=w809, "Input 2"=w812) -> (w806:T26)  [unwired: 1 in]
                n320 = To Variant(anything=w806) -> (Variant=w815:variant)
                n321 = call <vilib>:"DB Tools Insert Data.vi"("data"=w815, "error in (no error)"=w818, "columns"=string[] ["DATE", "SHIFT", "ST5_SCREW1_DATA", "ST5_SCREW1_STATUS", "ST5_SCREW2_DATA", "ST5_SCREW2_STATUS", "ST5_SCREW3_DATA", "ST5_FINAL_RST"], "table"="ST5_REPORT", "connection reference"=w819) -> ("error out"=w816:errorcluster, "connection reference out"=w817:T16)  [unwired: 5 in]
              }
            }
            n322 = call <vilib>:"Simple Error Handler.vi"("type of dialog (OK msg:1)"=w769, "error in (no error)"=w770) -> ("error out"=w768:errorcluster)  [unwired: 3 in, 4 out]
            n323 = call <vilib>:"Clear Errors.vi"("error in (no error)"=w768) -> ("error out"=w766:errorcluster)  [unwired: 5 in, 1 out]
            n324 = flat-sequence {
              tunnel: [w778] -> w757
              tunnel: w766 -> [w778]
              frame #0 {
                # "UPDATE op 20 save"
                n325 = global write "DATA LOG.vi" "OP 50 reset"(TRUE) -> ()
              }
            }
          }
          frame "SCAN6" {
            # "STATION OP 60"
            n326 = case shown="False" w826 {
              tunnel: w830 -> [w851 w857]
              tunnel: w829 -> [w844 w856]
              tunnel: w828 -> [_ _]
              tunnel: [w846 w855] -> w825
              tunnel: [w845 w857] -> w827
              tunnel: [w836 "" ("trimmed string")] -> _
              frame False {
                n327 = call "PADMINI_AUTO_BARCODE_STRING 60.vi"("Enum"=enum16{"Read", "Write"}."Read", "error in (no error)"=w844) -> ("error out"=w843:errorcluster, "Input 2"=w838:string[])  [unwired: 8 in]
                n328 = Index Array(array=w838) -> (element=w837:string)  [unwired: 1 in]
                n329 = call <vilib>:"Trim Whitespace.vi"("string"=w837) -> ("trimmed string"=w836:string)  [unwired: 1 in]
                n330 = Format Into String(format string="WHERE BARCODE  ='%s'", w836) -> (resulting string=w839:string)  [unwired: 2 in, 1 out]
                n331 = call <vilib>:"DB Tools Select Data.vi"("condition"=w839, "error in (no error)"=w843, "columns"=string[] ["BARCODE", "OP50_FINAL_RESULT", "OP60_FINAL_RESULT"], "table"="REPORT", "connection reference"=w851) -> ("error out"=w849:errorcluster, "data"=w848:variant[][], "connection reference out"=w845:T16)  [unwired: 1 in]
                n332 = call "PADMINI_varient_to_data.vi"("error in (no error)"=w849, "data"=w848) -> ("error out"=w847:errorcluster, "Array"=w833:string[][])  [unwired: 8 in]
                n333 = Index Array(array=w833, index (row)=0 ("disabled index (col)")) -> (element=→"SCAN OP60":string[])  [unwired: 1 in]
                n334 = call "RESPONSE_LOGIC.vi"("Array"=w833) -> ("Not Found"=w831:i32[])  [unwired: 10 in]
                "OP60 STATUS" <- w831
                n335 = call "PADMINI_AUTO_BARCODE_STATUS 60.vi"("Enum"=enum16{"Read", "Write"}."Write", "error in (no error)"=w847, "I/P"=w831) -> ("error out"=w846:errorcluster)  [unwired: 7 in, 1 out]
              }
              frame True {
                w852 = i32[] [0, 0, 0, 0, 0]  # I/P
                n336 = call "PADMINI_AUTO_BARCODE_STATUS 60.vi"("Enum"=enum16{"Read", "Write"}."Write", "error in (no error)"=w856, "I/P"=w852) -> ("error out"=w855:errorcluster)  [unwired: 7 in, 1 out]
              }
            }
            n337 = flat-sequence {
              tunnel: [w859] -> w824
              tunnel: w825 -> [w859]
              frame #0 {
                # "UPDATE op 60 SCAN sTATUS"
                n338 = global write "DATA LOG.vi" "OP 60 Outputs"(TRUE) -> ()
              }
            }
          }
          frame "DATALOG6" {
            w873 = T17 2 items=["no dialog", "OK message", "continue or stop message", "OK message + warnings", "continue/stop + warnings"] ("type of dialog (OK msg:1)")
            # "datalog of OP 60"
            n339 = call "PADMINI_AUTO_BARCODE_STRING 60.vi"("Enum"=enum16{"Read", "Write"}."Read", "error in (no error)"=w865) -> ("error out"=w867:errorcluster, "Input 2"=w861:string[])  [unwired: 8 in]
            n340 = call "PADMINI_AUTO_CYCLE VALUE 60.vi"("Enum"=enum16{"Read", "Write"}."Read", "error in (no error)"=w865) -> ("Input 2"=w863:sgl[])  [unwired: 8 in, 1 out]
            n341 = Number To Fractional String(number=w863, precision (6)=i16 2) -> (F-format string=w862:string[])  [unwired: 2 in]
            n342 = case shown="False" w878 {
              tunnel: w879 -> [w906 w934]
              tunnel: w867 -> [w907 w933]
              tunnel: [w910 w932] -> w876
              tunnel: [w909 w931] -> w874
              tunnel: w877 -> [w905 _]
              tunnel: w862 -> [w901 w914]
              tunnel: w861 -> [w897 w913]
              frame False {
                # "DO TRACEBILITY"
                n343 = Index Array(array=w897) -> (element #1=w898:string, element #2=w889:string, element #3=w888:string, element #4=w887:string, element #5=w886:string, element #6=w885:string, element #7=w884:string, element #8=w883:string)  [unwired: 8 in]
                n344 = local read "SHIFT"() -> (w908:string)
                n345 = Index Array(array=w901) -> (element #1=w895:string, element #2=w894:string, element #3=w893:string, element #4=w892:string, element #5=w891:string, element #6=w890:string)  [unwired: 6 in]
                n346 = call <vilib>:"Trim Whitespace.vi"("string"=w898) -> ("trimmed string"=w899:string)  [unwired: 1 in]
                n347 = call "PADMINI_SHIFT_DATE.vi"("SHIFT"=w908) -> ("date/time string"=w896:string)  [unwired: 10 in]
                n348 = Format Into String(format string="Where BARCODE='%s' ", w899) -> (resulting string=w903:string)  [unwired: 2 in, 1 out]
                n349 = Bundle("date/time string"=w896, "Input 2"=w895, "Input 2"=w889, "Input 2"=w894, "Input 2"=w888, "Input 2"=w893, "Input 2"=w887, "Input 2"=w892, "Input 2"=w886, "Input 2"=w891, "Input 2"=w885, "Input 2"=w890, "Input 2"=w884, "Input 2"=w883) -> (w900:T27)  [unwired: 1 in]
                n350 = call <vilib>:"DB Tools Update Data.vi"("condition"=w903, "data"=w900, "error in (no error)"=w907, "columns"=string[] ["OP60_DATE", "OP60_SCREW1_DATA_Nm", "OP60_SCREW1_STATUS", "OP60_SCREW2_DATA_Nm", "OP60_SCREW2_STATUS", "OP60_SCREW3_DATA_Nm", "OP60_SCREW3_STATUS", "OP60_SCREW4_DATA_Nm", "OP60_SCREW4_STATUS", "OP60_SCREW5_DATA_Nm", "OP60_SCREW5_STATUS", "OP60_SCREW6_DATA_Nm", "OP60_SCREW6_STATUS", "OP60_FINAL_RESULT"], "table"=w905, "connection reference"=w906) -> ("error out"=w909:errorcluster, "connection reference out"=w910:T16)  [unwired: 4 in]
              }
              frame True {
                # "TRAC BYPASS"
                n351 = local read "SHIFT"() -> (w911:string)
                n352 = call "PADMINI_SHIFT_DATE.vi"("SHIFT"=w911) -> ("date/time string"=w912:string)  [unwired: 10 in]
                n353 = Index Array(array=w913) -> (element #2=w922:string, element #3=w921:string, element #4=w920:string, element #5=w918:string, element #6=w926:string, element #7=w927:string)  [unwired: 7 in, 1 out]
                n354 = Index Array(array=w914) -> (element #1=w925:string, element #2=w924:string, element #3=w923:string, element #4=w919:string, element #5=w917:string, element #6=w916:string)  [unwired: 6 in]
                n355 = Bundle("date/time string"=w912, "SHIFT"=w911, "Input 2"=w925, "Input 2"=w922, "Input 2"=w924, "Input 2"=w921, "Input 2"=w923, "Input 2"=w920, "Input 2"=w919, "Input 2"=w918, "Input 2"=w917, "Input 2"=w916, "Input 2"=w926, "Input 2"=w927) -> (w915:T28)  [unwired: 1 in]
                n356 = To Variant(anything=w915) -> (Variant=w930:variant)
                n357 = call <vilib>:"DB Tools Insert Data.vi"("data"=w930, "error in (no error)"=w933, "columns"=string[] ["DATE", "SHIFT", "ST6_SCREW1_DATA", "ST6_SCREW1_STATUS", "ST6_SCREW2_DATA", "ST6_SCREW2_STATUS", "ST6_SCREW3_DATA", "ST6_SCREW3_STATUS", "ST6_SCREW4_DATA", "ST6_SCREW4_STATUS", "ST6_SCREW5_DATA", "ST6_SCREW5_STATUS", "ST6_SCREW6_DATA", "ST6_SCREW6_STATUS", "ST6_FINAL_RST"], "table"="ST6_REPORT", "connection reference"=w934) -> ("error out"=w931:errorcluster, "connection reference out"=w932:T16)  [unwired: 5 in]
              }
            }
            n358 = call <vilib>:"Simple Error Handler.vi"("type of dialog (OK msg:1)"=w873, "error in (no error)"=w874) -> ("error out"=w872:errorcluster)  [unwired: 3 in, 4 out]
            n359 = call <vilib>:"Clear Errors.vi"("error in (no error)"=w872) -> ("error out"=w870:errorcluster)  [unwired: 5 in, 1 out]
            n360 = flat-sequence {
              tunnel: [w882] -> w860
              tunnel: w870 -> [w882]
              frame #0 {
                # "UPDATE op 20 save"
                n361 = global write "DATA LOG.vi" "OP 60 reset"(TRUE) -> ()
              }
            }
          }
          frame "SCAN7" {
            # "STATION OP 70"
            n362 = case shown="False" w941 {
              tunnel: w945 -> [w966 w972]
              tunnel: w944 -> [w959 w971]
              tunnel: w943 -> [w951 _]
              tunnel: [w961 w970] -> w940
              tunnel: [w960 w972] -> w942
              tunnel: [w952 "" ("trimmed string")] -> _
              frame False {
                n363 = call "PADMINI_AUTO_BARCODE_STRING 70.vi"("Enum"=enum16{"Read", "Write"}."Read", "error in (no error)"=w959) -> ("error out"=w958:errorcluster, "Input 2"=w954:string[])  [unwired: 8 in]
                n364 = Index Array(array=w954) -> (element=w953:string)  [unwired: 1 in]
                n365 = call <vilib>:"Trim Whitespace.vi"("string"=w953) -> ("trimmed string"=w952:string)  [unwired: 1 in]
                n366 = Format Into String(format string="WHERE BARCODE  ='%s'", w952) -> (resulting string=w955:string)  [unwired: 2 in, 1 out]
                n367 = call <vilib>:"DB Tools Select Data.vi"("condition"=w955, "error in (no error)"=w958, "columns"=string[] ["BARCODE", "OP60_FINAL_RESULT", "OP70_FINAL_RESULT"], "table"=w951, "connection reference"=w966) -> ("error out"=w964:errorcluster, "data"=w963:variant[][], "connection reference out"=w960:T16)  [unwired: 1 in]
                n368 = call "PADMINI_varient_to_data.vi"("error in (no error)"=w964, "data"=w963) -> ("error out"=w962:errorcluster, "Array"=w948:string[][])  [unwired: 8 in]
                n369 = Index Array(array=w948, index (row)=0 ("disabled index (col)")) -> (element=→"SCAN OP70":string[])  [unwired: 1 in]
                n370 = call "RESPONSE_LOGIC.vi"("Array"=w948) -> ("Not Found"=w946:i32[])  [unwired: 10 in]
                "OP70 STATUS" <- w946
                n371 = call "PADMINI_AUTO_BARCODE_STATUS 70.vi"("Enum"=enum16{"Read", "Write"}."Write", "error in (no error)"=w962, "I/P"=w946) -> ("error out"=w961:errorcluster)  [unwired: 7 in, 1 out]
              }
              frame True {
                w967 = i32[] [0, 0, 0, 0, 0]  # I/P
                n372 = call "PADMINI_AUTO_BARCODE_STATUS 70.vi"("Enum"=enum16{"Read", "Write"}."Write", "error in (no error)"=w971, "I/P"=w967) -> ("error out"=w970:errorcluster)  [unwired: 7 in, 1 out]
              }
            }
            n373 = flat-sequence {
              tunnel: [w974] -> w939
              tunnel: w940 -> [w974]
              frame #0 {
                # "UPDATE op 70 SCAN sTATUS"
                n374 = global write "DATA LOG.vi" "OP 70 Outputs"(TRUE) -> ()
              }
            }
          }
          frame "DATALOG7" {
            # "datalog of OP 70"
            n375 = call "PADMINI_AUTO_BARCODE_STRING 70.vi"("Enum"=enum16{"Read", "Write"}."Read", "error in (no error)"=w980) -> ("error out"=w982:errorcluster, "Input 2"=w976:string[])  [unwired: 8 in]
            n376 = call "PADMINI_AUTO_CYCLE VALUE 70.vi"("Enum"=enum16{"Read", "Write"}."Read", "error in (no error)"=w980) -> ("Input 2"=w978:sgl[])  [unwired: 8 in, 1 out]
            n377 = Number To Fractional String(number=w978, precision (6)=i16 4) -> (F-format string=w977:string[])  [unwired: 2 in]
            n378 = case shown="False" w990 {
              tunnel: w991 -> [w1009 w1027]
              tunnel: w982 -> [w1010 w1026]
              tunnel: [w1012 w1025] -> w988
              tunnel: [w1011 w1024] -> w986
              tunnel: w989 -> [w1008 _]
              tunnel: w977 -> [w1004 w1014]
              tunnel: w976 -> [w999 w1013]
              frame False {
                # "DO TRACEBILITY"
                n379 = Index Array(array=w999) -> (element #1=w1000:string, element #2=w998:string)  [unwired: 2 in]
                n380 = call <vilib>:"Trim Whitespace.vi"("string"=w1000) -> ("trimmed string"=w1001:string)  [unwired: 1 in]
                n381 = local read "SHIFT"() -> (w996:string)
                n382 = Index Array(array=w1004) -> (element #1=w1003:string, element #2=w997:string)  [unwired: 2 in]
                n383 = call "PADMINI_SHIFT_DATE.vi"("SHIFT"=w996) -> ("date/time string"=w995:string)  [unwired: 10 in]
                n384 = Bundle("date/time string"=w995, "Input 2"=w1003, "Input 2"=w997, "Input 2"=w998) -> (w1002:T29)  [unwired: 1 in]
                n385 = Format Into String(format string="Where BARCODE='%s' ", w1001) -> (resulting string=w1006:string)  [unwired: 2 in, 1 out]
                n386 = call <vilib>:"DB Tools Update Data.vi"("condition"=w1006, "data"=w1002, "error in (no error)"=w1010, "columns"=string[] ["OP70_DATE", "OP70_FULL_OPEN", "OP70_FULL_CLOSE", "OP70_FINAL_RESULT"], "table"=w1008, "connection reference"=w1009) -> ("error out"=w1011:errorcluster, "connection reference out"=w1012:T16)  [unwired: 4 in]
              }
              frame True {
                # "TRAC BYPASS"
                n387 = local read "SHIFT"() -> (w1015:string)
                n388 = call "PADMINI_SHIFT_DATE.vi"("SHIFT"=w1015) -> ("date/time string"=w1016:string)  [unwired: 10 in]
                n389 = Index Array(array=w1013) -> (element #2=w1019:string)  [unwired: 2 in, 1 out]
                n390 = Index Array(array=w1014) -> (element #1=w1020:string, element #2=w1018:string)  [unwired: 2 in]
                n391 = Bundle("date/time string"=w1016, "SHIFT"=w1015, "Input 2"=w1020, "Input 2"=w1018, "Input 2"=w1019) -> (w1017:T30)  [unwired: 1 in]
                n392 = To Variant(anything=w1017) -> (Variant=w1023:variant)
                n393 = call <vilib>:"DB Tools Insert Data.vi"("data"=w1023, "error in (no error)"=w1026, "columns"=string[] ["DATE_OP70", "SHIFT", "OP70_FULL_OPEN", "OP70_FULL_CLOSE", "OP70_FINAL_RST"], "table"="ST7_REPORT", "connection reference"=w1027) -> ("error out"=w1024:errorcluster, "connection reference out"=w1025:T16)  [unwired: 5 in]
              }
            }
            n394 = flat-sequence {
              tunnel: [w994] -> w975
              tunnel: w986 -> [w994]
              frame #0 {
                # "UPDATE op 20 save"
                n395 = global write "DATA LOG.vi" "OP 70 reset"(TRUE) -> ()
              }
            }
          }
          frame "SCAN8" {
            # "STATION OP 80"
            n396 = case shown="False" w1034 {
              tunnel: w1038 -> [w1059 w1065]
              tunnel: w1037 -> [w1052 w1064]
              tunnel: w1036 -> [w1044 _]
              tunnel: [w1054 w1063] -> w1033
              tunnel: [w1053 w1065] -> w1035
              tunnel: [w1045 "" ("trimmed string")] -> _
              frame False {
                (unwired) "REPORT"
                n397 = call "PADMINI_AUTO_BARCODE_STRING 80.vi"("Enum"=enum16{"Read", "Write"}."Read", "error in (no error)"=w1052) -> ("error out"=w1051:errorcluster, "Input 2"=w1047:string[])  [unwired: 8 in]
                n398 = Index Array(array=w1047) -> (element=w1046:string)  [unwired: 1 in]
                n399 = call <vilib>:"Trim Whitespace.vi"("string"=w1046) -> ("trimmed string"=w1045:string)  [unwired: 1 in]
                n400 = Format Into String(format string="WHERE BARCODE  ='%s'", w1045) -> (resulting string=w1048:string)  [unwired: 2 in, 1 out]
                n401 = call <vilib>:"DB Tools Select Data.vi"("condition"=w1048, "error in (no error)"=w1051, "columns"=string[] ["BARCODE", "OP70_FINAL_RESULT", "OP80_FINAL_RESULT"], "table"=w1044, "connection reference"=w1059) -> ("error out"=w1057:errorcluster, "data"=w1056:variant[][], "connection reference out"=w1053:T16)  [unwired: 1 in]
                n402 = call "PADMINI_varient_to_data.vi"("error in (no error)"=w1057, "data"=w1056) -> ("error out"=w1055:errorcluster, "Array"=w1041:string[][])  [unwired: 8 in]
                n403 = Index Array(array=w1041, index (row)=0 ("disabled index (col)")) -> (element=→"SCAN OP80":string[])  [unwired: 1 in]
                n404 = call "RESPONSE_LOGIC.vi"("Array"=w1041) -> ("Not Found"=w1040:i32[])  [unwired: 10 in]
                "OP80 STATUS" <- w1040
                n405 = call "PADMINI_AUTO_BARCODE_STATUS 80.vi"("Enum"=enum16{"Read", "Write"}."Write", "error in (no error)"=w1055, "I/P"=w1040) -> ("error out"=w1054:errorcluster)  [unwired: 7 in, 1 out]
              }
              frame True {
                w1060 = i32[] [0, 0, 0, 0, 0]  # I/P
                n406 = call "PADMINI_AUTO_BARCODE_STATUS 80.vi"("Enum"=enum16{"Read", "Write"}."Write", "error in (no error)"=w1064, "I/P"=w1060) -> ("error out"=w1063:errorcluster)  [unwired: 7 in, 1 out]
              }
            }
            n407 = flat-sequence {
              tunnel: [w1067] -> w1032
              tunnel: w1033 -> [w1067]
              frame #0 {
                # "UPDATE op 80 SCAN sTATUS"
                n408 = global write "DATA LOG.vi" "OP 80 Outputs"(TRUE) -> ()
              }
            }
          }
          frame "DATALOG8" {
            w1082 = T17 2 items=["no dialog", "OK message", "continue or stop message", "OK message + warnings", "continue/stop + warnings"] ("type of dialog (OK msg:1)")
            # "datalog of OP 80"
            n409 = call "PADMINI_AUTO_BARCODE_STRING 80.vi"("Enum"=enum16{"Read", "Write"}."Read", "error in (no error)"=w1074) -> ("error out"=w1076:errorcluster, "Input 2"=w1070:string[])  [unwired: 8 in]
            n410 = call "PADMINI_AUTO_CYCLE VALUE 80.vi"("Enum"=enum16{"Read", "Write"}."Read", "error in (no error)"=w1074) -> ("Input 2"=w1072:sgl[])  [unwired: 8 in, 1 out]
            n411 = Number To Fractional String(number=w1072, precision (6)=i16 2) -> (F-format string=w1071:string[])  [unwired: 2 in]
            n412 = case shown="True" w1068 {
              tunnel: w1087 -> [w1105 w1124]
              tunnel: w1076 -> [w1106 w1123]
              tunnel: [w1108 w1122] -> w1085
              tunnel: [w1107 w1121] -> w1083
              tunnel: w1086 -> [w1104 w1109]
              tunnel: w1071 -> [w1100 w1114]
              tunnel: w1070 -> [w1096 w1115]
              frame False {
                # "DO TRACEBILITY"
                n413 = Index Array(array=w1096) -> (element #1=w1097:string, element #2=w1092:string, element #3=w1091:string)  [unwired: 3 in]
                n414 = call <vilib>:"Trim Whitespace.vi"("string"=w1097) -> ("trimmed string"=w1098:string)  [unwired: 1 in]
                n415 = local read "SHIFT"() -> (w1095:string)
                n416 = Index Array(array=w1100) -> (element=w1093:string)  [unwired: 1 in]
                n417 = call "PADMINI_SHIFT_DATE.vi"("SHIFT"=w1095) -> ("date/time string"=w1094:string)  [unwired: 10 in]
                n418 = Bundle("date/time string"=w1094, "Input 2"=w1092, "Input 2"=w1093, "Input 2"=w1091) -> (w1099:T29)  [unwired: 1 in]
                n419 = Format Into String(format string="Where BARCODE='%s' ", w1098) -> (resulting string=w1102:string)  [unwired: 2 in, 1 out]
                n420 = call <vilib>:"DB Tools Update Data.vi"("condition"=w1102, "data"=w1099, "error in (no error)"=w1106, "columns"=string[] ["OP80_DATE", "OP80_LOCTITE_STATUS", "OP80_PLUG_PRESS_LOAD_kg", "OP80_FINAL_RESULT"], "table"=w1104, "connection reference"=w1105) -> ("error out"=w1107:errorcluster, "connection reference out"=w1108:T16)  [unwired: 4 in]
              }
              frame True {
                (unwired) "ST8_REPORT"
                # "TRAC BYPASS"
                n421 = local read "SHIFT"() -> (w1111:string)
                n422 = call "PADMINI_SHIFT_DATE.vi"("SHIFT"=w1111) -> ("date/time string"=w1110:string)  [unwired: 10 in]
                n423 = Index Array(array=w1115) -> (element #1=w1112:string, element #2=w1119:string, element #3=w1118:string)  [unwired: 3 in]
                n424 = Index Array(array=w1114) -> (element=w1117:string)  [unwired: 1 in]
                n425 = Bundle("Input 2"=w1112, "SHIFT"=w1111, "date/time string"=w1110, "Input 2"=w1117, "Input 2"=w1119, "Input 2"=w1118) -> (w1116:T31)  [unwired: 1 in]
                n426 = To Variant(anything=w1116) -> (Variant=w1120:variant)
                n427 = call <vilib>:"DB Tools Insert Data.vi"("data"=w1120, "error in (no error)"=w1123, "columns"=string[] ["BARCODE", "SHIFT", "OP80_DATE", "OP80_LOCTITE_STATUS", "OP80_PLUG_PRESS_LOAD_kg", "OP80_FINAL_RESULT"], "table"=w1109, "connection reference"=w1124) -> ("error out"=w1121:errorcluster, "connection reference out"=w1122:T16)  [unwired: 5 in]
              }
            }
            n428 = call <vilib>:"Simple Error Handler.vi"("type of dialog (OK msg:1)"=w1082, "error in (no error)"=w1083) -> ("error out"=w1081:errorcluster)  [unwired: 3 in, 4 out]
            n429 = call <vilib>:"Clear Errors.vi"("error in (no error)"=w1081) -> ("error out"=w1079:errorcluster)  [unwired: 5 in, 1 out]
            n430 = flat-sequence {
              tunnel: [w1090] -> w1069
              tunnel: w1079 -> [w1090]
              frame #0 {
                # "UPDATE op 20 save"
                n431 = global write "DATA LOG.vi" "OP 80 reset"(TRUE) -> ()
              }
            }
          }
          frame "SCAN9" {
            # "STATION OP 90"
            n432 = case shown="False" w1131 {
              tunnel: w1135 -> [w1156 w1162]
              tunnel: w1134 -> [w1149 w1161]
              tunnel: w1133 -> [w1141 _]
              tunnel: [w1151 w1160] -> w1130
              tunnel: [w1150 w1162] -> w1132
              tunnel: [w1142 "" ("trimmed string")] -> _
              frame False {
                (unwired) "REPORT"
                n433 = call "PADMINI_AUTO_BARCODE_STRING 90.vi"("Enum"=enum16{"Read", "Write"}."Read", "error in (no error)"=w1149) -> ("error out"=w1148:errorcluster, "Input 2"=w1144:string[])  [unwired: 8 in]
                n434 = Index Array(array=w1144) -> (element=w1143:string)  [unwired: 1 in]
                n435 = call <vilib>:"Trim Whitespace.vi"("string"=w1143) -> ("trimmed string"=w1142:string)  [unwired: 1 in]
                n436 = Format Into String(format string="WHERE BARCODE  ='%s'", w1142) -> (resulting string=w1145:string)  [unwired: 2 in, 1 out]
                n437 = call <vilib>:"DB Tools Select Data.vi"("condition"=w1145, "error in (no error)"=w1148, "columns"=string[] ["BARCODE", "OP80_FINAL_RESULT", "OP90_FINAL_RESULT"], "table"=w1141, "connection reference"=w1156) -> ("error out"=w1154:errorcluster, "data"=w1153:variant[][], "connection reference out"=w1150:T16)  [unwired: 1 in]
                n438 = call "PADMINI_varient_to_data.vi"("error in (no error)"=w1154, "data"=w1153) -> ("error out"=w1152:errorcluster, "Array"=w1138:string[][])  [unwired: 8 in]
                n439 = Index Array(array=w1138, index (row)=0 ("disabled index (col)")) -> (element=→"SCAN OP90":string[])  [unwired: 1 in]
                n440 = call "RESPONSE_LOGIC.vi"("Array"=w1138) -> ("Not Found"=w1136:i32[])  [unwired: 10 in]
                "OP90 STATUS" <- w1136
                n441 = call "PADMINI_AUTO_BARCODE_STATUS 90.vi"("Enum"=enum16{"Read", "Write"}."Write", "error in (no error)"=w1152, "I/P"=w1136) -> ("error out"=w1151:errorcluster)  [unwired: 7 in, 1 out]
              }
              frame True {
                w1157 = i32[] [0, 0, 0, 0, 0]  # I/P
                n442 = call "PADMINI_AUTO_BARCODE_STATUS 90.vi"("Enum"=enum16{"Read", "Write"}."Write", "error in (no error)"=w1161, "I/P"=w1157) -> ("error out"=w1160:errorcluster)  [unwired: 7 in, 1 out]
              }
            }
            n443 = flat-sequence {
              tunnel: [w1164] -> w1129
              tunnel: w1130 -> [w1164]
              frame #0 {
                # "UPDATE op 90 SCAN sTATUS"
                n444 = global write "DATA LOG.vi" "OP 90 Outputs"(TRUE) -> ()
              }
            }
          }
          frame "DATALOG9" {
            w1178 = T17 2 items=["no dialog", "OK message", "continue or stop message", "OK message + warnings", "continue/stop + warnings"] ("type of dialog (OK msg:1)")
            # "datalog of OP 90"
            n445 = call "PADMINI_AUTO_BARCODE_STRING 90.vi"("Enum"=enum16{"Read", "Write"}."Read", "error in (no error)"=w1170) -> ("error out"=w1172:errorcluster, "Input 2"=w1167:string[])  [unwired: 8 in]
            n446 = call "PADMINI_AUTO_CYCLE VALUE 90.vi"("Enum"=enum16{"Read", "Write"}."Read", "error in (no error)"=w1170) -> ("Input 2"=w1166:sgl[])  [unwired: 8 in, 1 out]
            n447 = Number To Fractional String(number=w1166, precision (6)=i16 2) -> (F-format string=w1168:string[])  [unwired: 2 in]
            n448 = case shown="False" w1183 {
              tunnel: w1184 -> [w1203 w1222]
              tunnel: w1172 -> [w1204 w1221]
              tunnel: [w1206 w1220] -> w1181
              tunnel: [w1205 w1219] -> w1179
              tunnel: w1182 -> [w1202 _]
              tunnel: w1168 -> [w1198 w1211]
              tunnel: w1167 -> [w1194 w1210]
              frame False {
                # "DO TRACEBILITY"
                n449 = Index Array(array=w1194) -> (element #1=w1195:string, element #2=w1192:string, element #3=w1190:string)  [unwired: 3 in]
                n450 = call <vilib>:"Trim Whitespace.vi"("string"=w1195) -> ("trimmed string"=w1196:string)  [unwired: 1 in]
                n451 = local read "SHIFT"() -> (w1189:string)
                n452 = Index Array(array=w1198) -> (element #1=w1193:string, element #2=w1191:string)  [unwired: 2 in]
                n453 = call "PADMINI_SHIFT_DATE.vi"("SHIFT"=w1189) -> ("date/time string"=w1188:string)  [unwired: 10 in]
                n454 = Bundle("date/time string"=w1188, "Input 2"=w1193, "Input 2"=w1192, "Input 2"=w1191, "Input 2"=w1190) -> (w1197:T22)  [unwired: 1 in]
                n455 = Format Into String(format string="Where BARCODE='%s' ", w1196) -> (resulting string=w1200:string)  [unwired: 2 in, 1 out]
                n456 = call <vilib>:"DB Tools Update Data.vi"("condition"=w1200, "data"=w1197, "error in (no error)"=w1204, "columns"=string[] ["OP90_DATE", "OP90_SEAT_LEAK_LP", "OP90_SEAT_STATUS", "OP90_STEAM_LEAK_sccm", "OP90_FINAL_RESULT"], "table"=w1202, "connection reference"=w1203) -> ("error out"=w1205:errorcluster, "connection reference out"=w1206:T16)  [unwired: 4 in]
              }
              frame True {
                # "TRAC BYPASS"
                n457 = local read "SHIFT"() -> (w1207:string)
                n458 = call "PADMINI_SHIFT_DATE.vi"("SHIFT"=w1207) -> ("date/time string"=w1208:string)  [unwired: 10 in]
                n459 = Index Array(array=w1210) -> (element #2=w1215:string, element #3=w1213:string)  [unwired: 3 in, 1 out]
                n460 = Index Array(array=w1211) -> (element #1=w1216:string, element #2=w1214:string)  [unwired: 2 in]
                n461 = Bundle("date/time string"=w1208, "SHIFT"=w1207, "Input 2"=w1216, "Input 2"=w1215, "Input 2"=w1214, "Input 2"=w1213) -> (w1212:T23)  [unwired: 1 in]
                n462 = To Variant(anything=w1212) -> (Variant=w1218:variant)
                n463 = call <vilib>:"DB Tools Insert Data.vi"("data"=w1218, "error in (no error)"=w1221, "columns"=string[] ["DATE", "SHIFT", "ST9_SEAT_LT_DATA", "ST9_SEAT_STATUS", "ST9_STEAM_LT_DATA", "ST9_FINAL_RST"], "table"="ST9_REPORT", "connection reference"=w1222) -> ("error out"=w1219:errorcluster, "connection reference out"=w1220:T16)  [unwired: 5 in]
              }
            }
            n464 = call <vilib>:"Simple Error Handler.vi"("type of dialog (OK msg:1)"=w1178, "error in (no error)"=w1179) -> ("error out"=w1177:errorcluster)  [unwired: 3 in, 4 out]
            n465 = call <vilib>:"Clear Errors.vi"("error in (no error)"=w1177) -> ("error out"=w1175:errorcluster)  [unwired: 5 in, 1 out]
            n466 = flat-sequence {
              tunnel: [w1187] -> w1165
              tunnel: w1175 -> [w1187]
              frame #0 {
                # "UPDATE op 20 save"
                n467 = global write "DATA LOG.vi" "OP 90 reset"(TRUE) -> ()
              }
            }
          }
          frame "SCAN10" {
            # "STATION OP 10"
            n468 = case shown="False" w1229 {
              tunnel: w1233 -> [w1254 w1260]
              tunnel: w1232 -> [w1248 w1259]
              tunnel: w1231 -> [w1240 _]
              tunnel: [w1238 w1258] -> w1228
              tunnel: [w1249 w1260] -> w1230
              tunnel: [w1241 "" ("trimmed string")] -> _
              frame False {
                (unwired) "REPORT"
                n469 = call "PADMINI_AUTO_BARCODE_STRING 100.vi"("Enum"=enum16{"Read", "Write"}."Read", "error in (no error)"=w1248) -> ("error out"=w1247:errorcluster, "Input 2"=w1243:string[])  [unwired: 8 in]
                n470 = Index Array(array=w1243) -> (element=w1242:string)  [unwired: 1 in]
                n471 = call <vilib>:"Trim Whitespace.vi"("string"=w1242) -> ("trimmed string"=w1241:string)  [unwired: 1 in]
                n472 = Format Into String(format string="WHERE BARCODE  ='%s'", w1241) -> (resulting string=w1244:string)  [unwired: 2 in, 1 out]
                n473 = call <vilib>:"DB Tools Select Data.vi"("condition"=w1244, "error in (no error)"=w1247, "columns"=string[] ["BARCODE", "OP90_FINAL_RESULT", "OP100_FINAL_RESULT"], "table"=w1240, "connection reference"=w1254) -> ("error out"=w1252:errorcluster, "data"=w1251:variant[][], "connection reference out"=w1249:T16)  [unwired: 1 in]
                n474 = call "PADMINI_varient_to_data.vi"("error in (no error)"=w1252, "data"=w1251) -> ("error out"=w1250:errorcluster, "Array"=w1236:string[][])  [unwired: 8 in]
                n475 = Index Array(array=w1236, index (row)=0 ("disabled index (col)")) -> (element=→"SCAN OP100":string[])  [unwired: 1 in]
                n476 = call "RESPONSE_LOGIC.vi"("Array"=w1236) -> ("Not Found"=w1234:i32[])  [unwired: 10 in]
                "OP100 STATUS" <- w1234
                n477 = call "PADMINI_AUTO_BARCODE_STATUS 100.vi"("Enum"=enum16{"Read", "Write"}."Write", "error in (no error)"=w1250, "I/P"=w1234) -> ("error out"=w1238:errorcluster)  [unwired: 7 in, 1 out]
              }
              frame True {
                w1255 = i32[] [0, 0, 0, 0, 0]  # I/P
                n478 = call "PADMINI_AUTO_BARCODE_STATUS 100.vi"("Enum"=enum16{"Read", "Write"}."Write", "error in (no error)"=w1259, "I/P"=w1255) -> ("error out"=w1258:errorcluster)  [unwired: 7 in, 1 out]
              }
            }
            n479 = flat-sequence {
              tunnel: [w1262] -> w1227
              tunnel: w1228 -> [w1262]
              frame #0 {
                # "UPDATE op 100 SCAN sTATUS"
                n480 = global write "DATA LOG.vi" "OP 100 Outputs"(TRUE) -> ()
              }
            }
          }
          frame "SCAN11" {
            # "STATION OP 110"
            n481 = case shown="False" w1269 {
              tunnel: w1273 -> [w1306 w1331]
              tunnel: w1272 -> [w1280 w1330]
              tunnel: w1271 -> [w1283 _]
              tunnel: [w1303 w1329] -> w1268
              tunnel: [w1285 w1331] -> w1270
              frame False {
                (unwired) "P5314216;S07122024020102;VA1105000100"
                # "OP100 OK\nOP 100 NG"
                n482 = call "PADMINI_AUTO_BARCODE_STRING 110.vi"("Enum"=enum16{"Read", "Write"}."Read", "error in (no error)"=w1280) -> ("error out"=w1281:errorcluster, "Input 2"=w1279:string[])  [unwired: 8 in]
                n483 = Index Array(array=w1279) -> (element=w1300:string)  [unwired: 1 in]
                n484 = call <vilib>:"Trim Whitespace.vi"("string"=w1300) -> ("trimmed string"=w1277:string)  [unwired: 1 in]
                n485 = call "String_Conversion_OP110.vi"("String in"=w1277) -> ("String out"=w1278:string)  [unwired: 9 in, 1 out]
                n486 = Format Into String(format string="WHERE BARCODE  ='%s'", w1278) -> (resulting string=w1284:string)  [unwired: 2 in, 1 out]
                "resulting string" <- w1284
                n487 = call <vilib>:"DB Tools Select Data.vi"("condition"=w1284, "error in (no error)"=w1281, "columns"=string[] ["BARCODE", "OP100_FINAL_RESULT", "OP110_BIN_NO"], "table"=w1283, "connection reference"=w1306) -> ("error out"=w1305:errorcluster, "data"=w1304:variant[][], "connection reference out"=w1286:T16)  [unwired: 1 in]
                n488 = call "PADMINI_varient_to_data.vi"("error in (no error)"=w1305, "data"=w1304) -> ("error out"=w1287:errorcluster, "Array"=w1291:string[][])  [unwired: 8 in]
                n489 = Index Array(array=w1291, index (row)=0 ("disabled index (col)")) -> (element=w1290:string[])  [unwired: 1 in]
                "SCAN OP110" <- w1290
                n490 = Index Array(array=w1290) -> (element #1=w1298:string, element #2=w1295:string, element #3=w1275:string)  [unwired: 3 in]
                n491 = Equal?(x=w1275, y="") -> (x = y?=w1274:bool)
                n492 = Equal?(x="", y=w1298) -> (x = y?=w1297:bool)
                n493 = Equal?(x=w1295, y="OK") -> (x = y?=w1296:bool)
                n494 = case shown="False" w1297 {
                  tunnel: w1296 -> [w1313 _]
                  tunnel: [w1314 w1326] -> w1289
                  tunnel: [w1312 w1325] -> w1288
                  tunnel: w1287 -> [w1311 w1325]
                  tunnel: w1286 -> [w1310 w1324]
                  tunnel: [w1309 w1324] -> w1285
                  tunnel: w1283 -> [w1308 _]
                  tunnel: w1274 -> [w1307 _]
                  frame False {
                    # "BARCODE FOUND"
                    n495 = case shown="True" w1313 {
                      tunnel: [w1317 w1319] -> w1314
                      tunnel: [w1316 w1323] -> w1312
                      tunnel: w1311 -> [w1316 w1323]
                      tunnel: w1310 -> [w1315 w1322]
                      tunnel: [w1315 w1322] -> w1309
                      tunnel: w1308 -> [_ _]
                      tunnel: w1307 -> [_ w1321]
                      frame False {
                        w1317 = i32[] [0, 1, 0]  # OK
                        # "CT ST REPEAT NG & EMPTY"
                      }
                      frame True {
                        w1318 = i32[] [1, 0, 1]  # OK but repeat
                        w1320 = i32[] [1, 0, 0]  # OK and not repeat
                        # "CT ST REPEAT EMPTY"
                        n496 = Select(t=w1320, s=w1321, f=w1318) -> (s? t:f=w1319:i32[])
                      }
                    }
                  }
                  frame True {
                    w1326 = i32[] [0, 1, 0]  # Not Found
                    # "nO BARCODE FOUND"
                  }
                }
                "OP110 STATUS" <- w1289
                n497 = call "PADMINI_AUTO_BARCODE_STATUS 110.vi"("Enum"=enum16{"Read", "Write"}."Write", "error in (no error)"=w1288, "I/P"=w1289) -> ("error out"=w1303:errorcluster)  [unwired: 7 in, 1 out]
              }
              frame True {
                w1327 = i32[] [0, 0, 0, 0, 0]  # I/P
                n498 = call "PADMINI_AUTO_BARCODE_STATUS 100.vi"("Enum"=enum16{"Read", "Write"}."Write", "error in (no error)"=w1330, "I/P"=w1327) -> ("error out"=w1329:errorcluster)  [unwired: 7 in, 1 out]
              }
            }
            n499 = flat-sequence {
              tunnel: [w1333] -> w1267
              tunnel: w1268 -> [w1333]
              frame #0 {
                # "UPDATE op 100 SCAN sTATUS"
                n500 = global write "DATA LOG.vi" "OP 110 Outputs"(TRUE) -> ()
              }
            }
          }
          frame "DATALOG10" {
            w1347 = T17 2 items=["no dialog", "OK message", "continue or stop message", "OK message + warnings", "continue/stop + warnings"] ("type of dialog (OK msg:1)")
            # "datalog of OP 100"
            n501 = call "PADMINI_AUTO_BARCODE_STRING 100.vi"("Enum"=enum16{"Read", "Write"}."Read", "error in (no error)"=w1335) -> ("error out"=w1341:errorcluster, "Input 2"=w1337:string[])  [unwired: 8 in]
            n502 = call "PADMINI_AUTO_CYCLE VALUE 100.vi"("Enum"=enum16{"Read", "Write"}."Read", "error in (no error)"=w1335) -> ("Input 2"=w1336:sgl[])  [unwired: 8 in, 1 out]
            n503 = Number To Fractional String(number=w1336, precision (6)=i16 2) -> (F-format string=w1338:string[])  [unwired: 2 in]
            n504 = case shown="False" w1352 {
              tunnel: w1353 -> [w1381 w1406]
              tunnel: w1341 -> [w1382 w1405]
              tunnel: [w1384 w1404] -> w1350
              tunnel: [w1383 w1403] -> w1348
              tunnel: w1351 -> [w1380 _]
              tunnel: w1338 -> [w1376 w1388]
              tunnel: w1337 -> [w1373 w1389]
              frame False {
                # "DO TRACEBILITY"
                n505 = Index Array(array=w1373) -> (element #1=w1372:string, element #2=w1358:string, element #3=w1357:string)  [unwired: 3 in]
                n506 = call <vilib>:"Trim Whitespace.vi"("string"=w1372) -> ("trimmed string"=w1374:string)  [unwired: 1 in]
                n507 = Index Array(array=w1376) -> (element #1=w1369:string, element #2=w1368:string, element #3=w1367:string, element #4=w1366:string, element #5=w1365:string, element #6=w1364:string, element #7=w1363:string, element #8=w1362:string, element #9=w1361:string, element #10=w1360:string, element #11=w1359:string)  [unwired: 11 in]
                n508 = local read "SHIFT"() -> (w1371:string)
                n509 = call "PADMINI_SHIFT_DATE.vi"("SHIFT"=w1371) -> ("date/time string"=w1370:string)  [unwired: 10 in]
                n510 = Bundle("date/time string"=w1370, "Input 2"=w1369, "Input 2"=w1368, "Input 2"=w1367, "Input 2"=w1366, "Input 2"=w1365, "Input 2"=w1364, "Input 2"=w1363, "Input 2"=w1362, "Input 2"=w1361, "Input 2"=w1360, "Input 2"=w1359, "Input 2"=w1358, "Input 2"=w1357) -> (w1375:T27)  [unwired: 1 in]
                n511 = Format Into String(format string="Where BARCODE='%s' ", w1374) -> (resulting string=w1378:string)  [unwired: 2 in, 1 out]
                n512 = call <vilib>:"DB Tools Update Data.vi"("condition"=w1378, "data"=w1375, "error in (no error)"=w1382, "columns"=string[] ["OP100_DATE", "OP100_SENSOR_OP_OPEN_V", "OP100_SENSOR_OP_CLOSE_V", "OP100_SENSOR_OP_FULL_CLOSE_V", "OP100_SENSOR_INITIAL_V", "OP100_MOTOR_START_OF_CLOSE_V", "OP100_MOTOR_FULL_CLOSE_V", "OP100_MOTOR_START_BACK_V", "OP100_MOTOR_FULL_OPEN_V", "OP100_RESPONSE_TIME_FWD_msec", "OP100_RESPONSE_TIME_REV_msec", "OP100_MOTOR_PEAK_CURRENT_A", "OP100_FINAL_RESULT", "OP100_CONNECTOR_CAMERA_STATUS"], "table"=w1380, "connection reference"=w1381) -> ("error out"=w1383:errorcluster, "connection reference out"=w1384:T16)  [unwired: 4 in]
              }
              frame True {
                # "TRAC BYPASS"
                n513 = local read "SHIFT"() -> (w1386:string)
                n514 = Index Array(array=w1389) -> (element=w1393:string)  [unwired: 1 in]
                n515 = call "PADMINI_SHIFT_DATE.vi"("SHIFT"=w1386) -> ("date/time string"=w1387:string)  [unwired: 10 in]
                n516 = Index Array(array=w1388) -> (element #1=w1399:string, element #2=w1398:string, element #3=w1385:string, element #4=w1391:string, element #5=w1397:string, element #6=w1392:string, element #7=w1396:string, element #8=w1395:string, element #9=w1394:string)  [unwired: 9 in]
                n517 = Bundle("date/time string"=w1387, "SHIFT"=w1386, "Input 2"=w1399, "Input 2"=w1398, "Input 2"=w1385, "Input 2"=w1385, "Input 2"=w1385, "Input 2"=w1391, "Input 2"=w1397, "Input 2"=w1392, "Input 2"=w1396, "Input 2"=w1395, "Input 2"=w1394, "Input 2"=w1393) -> (w1390:T28)  [unwired: 1 in]
                n518 = To Variant(anything=w1390) -> (Variant=w1402:variant)
                n519 = call <vilib>:"DB Tools Insert Data.vi"("data"=w1402, "error in (no error)"=w1405, "columns"=string[] ["DATE", "SHIFT", "ST10_SENSOR_OP_OPEN_V", "ST10_START_OF_CLOSE_SENSOR_V", "ST10_SENSOR_OP_FULL_CLOSE_V", "ST10_RESPONSE_TIME_FWD", "ST10_RESPONSE_TIME_REV", "ST10_MOTOR_V_START_OF_CLOSE_A", "ST10_MOTOR_V_FULL_CLOSE_B", "ST10_MOTOR_V_START_BACK_C", "ST10_MOTOR_V_FULL_OPEN_D", "ST10_MOTOR_RMS_CURRENT_A", "ST10_FINAL_RST"], "table"="ST10_REPORT", "connection reference"=w1406) -> ("error out"=w1403:errorcluster, "connection reference out"=w1404:T16)  [unwired: 5 in]
              }
            }
            n520 = call <vilib>:"Simple Error Handler.vi"("type of dialog (OK msg:1)"=w1347, "error in (no error)"=w1348) -> ("error out"=w1346:errorcluster)  [unwired: 3 in, 4 out]
            n521 = call <vilib>:"Clear Errors.vi"("error in (no error)"=w1346) -> ("error out"=w1344:errorcluster)  [unwired: 5 in, 1 out]
            n522 = flat-sequence {
              tunnel: [w1356] -> w1334
              tunnel: w1344 -> [w1356]
              frame #0 {
                # "UPDATE op 20 save"
                n523 = global write "DATA LOG.vi" "OP 100 reset"(TRUE) -> ()
              }
            }
          }
          frame "DATALOG11" {
            (unwired) "WHERE BARCODE  ='%s'" ("format string")
            w1429 = T17 2 items=["no dialog", "OK message", "continue or stop message", "OK message + warnings", "continue/stop + warnings"] ("type of dialog (OK msg:1)")
            # "datalog of OP 110"
            n524 = call "PADMINI_AUTO_BARCODE_STRING 110.vi"("Enum"=enum16{"Read", "Write"}."Read", "error in (no error)"=w1420) -> ("error out"=w1419:errorcluster, "Input 2"=w1418:string[])  [unwired: 8 in]
            n525 = Index Array(array=w1418) -> (element=w1423:string)  [unwired: 1 in]
            n526 = call <vilib>:"Trim Whitespace.vi"("string"=w1423) -> ("trimmed string"=w1421:string)  [unwired: 1 in]
            n527 = call "String_Conversion_OP110.vi"("String in"=w1421) -> ("String out"=w1417:string)  [unwired: 9 in, 1 out]
            n528 = Index Array(array=w1418) -> (element #2=w1412:string, element #3=w1411:string)  [unwired: 3 in, 1 out]
            n529 = local read "SHIFT"() -> (w1408:string)
            n530 = call <vilib>:"Trim Whitespace.vi"("string"=w1411) -> ("trimmed string"=w1415:string)  [unwired: 1 in]
            n531 = call <vilib>:"Trim Whitespace.vi"("string"=w1412) -> ("trimmed string"=w1414:string)  [unwired: 1 in]
            n532 = call "PADMINI_SHIFT_DATE.vi"("SHIFT"=w1408) -> ("date/time string"=w1407:string)  [unwired: 10 in]
            n533 = Bundle("date/time string"=w1407, "trimmed string"=w1414, "trimmed string"=w1415) -> (w1410:T32)  [unwired: 1 in]
            n534 = Format Into String(format string="WHERE BARCODE  ='%s'", w1417) -> (resulting string=w1416:string)  [unwired: 2 in, 1 out]
            n535 = call <vilib>:"DB Tools Update Data.vi"("condition"=w1416, "data"=w1410, "error in (no error)"=w1419, "columns"=string[] ["OP110_DATE", "OP110_BIN_NO", "OP110_PALLET_NO"], "table"=w1433, "connection reference"=w1434) -> ("error out"=w1430:errorcluster, "connection reference out"=w1432:T16)  [unwired: 4 in]
            n536 = call <vilib>:"Simple Error Handler.vi"("type of dialog (OK msg:1)"=w1429, "error in (no error)"=w1430) -> ("error out"=w1428:errorcluster)  [unwired: 3 in, 4 out]
            n537 = call <vilib>:"Clear Errors.vi"("error in (no error)"=w1428) -> ("error out"=w1426:errorcluster)  [unwired: 5 in, 1 out]
            n538 = flat-sequence {
              tunnel: [w1437] -> w1424
              tunnel: w1426 -> [w1437]
              frame #0 {
                # "UPDATE op 20 save"
                n539 = global write "DATA LOG.vi" "OP 110 reset"(TRUE) -> ()
              }
            }
          }
          frame "EMERGENCY STOP" {
          }
          frame "STOP" {
            n540 = global read "Global 1.vi" "BARCODE RECIPE"() -> (w1448:string)
            n541 = Bundle("BARCODE RECIPE"=w1448) -> (w1447:cluster{"BARCODE RECIPE":string})  [unwired: 1 in]
            n542 = call <vilib>:"DB Tools Update Data.vi"("data"=w1447, "error in (no error)"=w1453, "columns"=string[] ["PREVIOUS_LOADED_RECIPE"], "table"="BARCODE_RECIPE", "connection reference"=w1451) -> ("error out"=w1452:errorcluster, "connection reference out"=w1450:T16)  [unwired: 5 in]
          }
        }
      }
      frame Error {
        # "Return true in any case that should stop the loop."
      }
    }
    n543 = Unbundle By Name(w130) -> ("OP - 90"=→"OP - 90":T33, "OP - 100"=→"OP - 100":T12, "OP - 110"=→"OP - 110":T9)
    n544 = Unbundle By Name(w130) -> ("OP - 10"=→"OP - 10":T34, "OP - 20"=→"OP - 20":T6, "OP - 30"=→"OP - 30":T35, "OP - 40"=→"OP - 40":T3)
    n545 = Unbundle By Name(w130) -> ("OP - 50"=→"OP - 50":T2, "OP - 60"=→"OP - 60":T36, "OP - 70"=→"OP - 70":T37, "OP - 80"=→"OP - 80":T38)
    n546 = Wait (ms)(milliseconds to wait=u32 100) -> ()  [unwired: 1 out]
    n547 = call <vilib>:"Simple Error Handler.vi"("error in (no error)"=w125) -> ("error out"=w124:errorcluster)  [unwired: 4 in, 4 out]
  }
  n548 = while {
    shift-right: [w1486] -> w72
    shift-left: w22 -> [w1480]
    shift-right: [w1487] -> w66
    shift-left: w70 -> [w1495]
    stop <- w1485 stop-if-true
    n549 = local read "Shift_change"() -> (w1493:bool)
    n550 = call <vilib>:"Clear Errors.vi"("error in (no error)"=w1480) -> ("error out"=w1471:errorcluster)  [unwired: 5 in, 1 out]
    n551 = call "READ EMERGENCY BIT.vi"("Enum"=enum16{"Read", "Write"}."Read", "error in (no error)"=w1471) -> ("Array Out"=w1483:dbl[])  [unwired: 8 in, 1 out]
    n552 = case shown="True" w1493 {
      tunnel: w1471 -> [w1512 w1525]
      tunnel: [w1513 w1524] -> w1492
      frame False {
        n553 = local read "SHIFT_DATA 2"() -> (w1515:string[])
        n554 = Get Date/Time In Seconds() -> (seconds since 1Jan1904=w1514:timestamp)
        n555 = call "String To Time_4.vi"("error in (no error)"=w1512, "String Array In"=w1515) -> ("error out"=w1511:errorcluster, "Time Stamp Out"=w1510:timestamp[])  [unwired: 8 in]
        "Time Stamp Out 4" <- w1510
        n556 = call "Shift Calculation_4.vi"("error in (no error)"=w1511, "Current Time"=w1514, "Time Stamp Out"=w1510) -> ("error out"=w1509:errorcluster, "Shift"=w1508:i32)  [unwired: 7 in]
        n557 = call <vilib>:"Clear Errors.vi"("error in (no error)"=w1509) -> ()  [unwired: 5 in, 2 out]
        n558 = case shown="4" w1508 {
          tunnel: ["A" "B" "C" "D"] -> w1513
          frame 1, Default {
          }
          frame 2 {
          }
          frame 3 {
          }
          frame 4 {
          }
        }
      }
      frame True {
        n559 = local read "SHIFT_DATA"() -> (w1523:string[])
        n560 = Get Date/Time In Seconds() -> (seconds since 1Jan1904=w1526:timestamp)
        n561 = call "String To Time.vi"("error in (no error)"=w1525, "String Array In"=w1523) -> ("error out"=w1522:errorcluster, "Time Stamp Out"=w1527:timestamp[])  [unwired: 8 in]
        "Time Stamp Out" <- w1527
        n562 = call "Shift Calculation.vi"("error in (no error)"=w1522, "Current Time"=w1526, "Time Stamp Out"=w1527) -> ("error out"=w1521:errorcluster, "Shift"=w1520:i32)  [unwired: 7 in]
        "Shift 4" <- w1520
        n563 = call <vilib>:"Clear Errors.vi"("error in (no error)"=w1521) -> ()  [unwired: 5 in, 2 out]
        n564 = case shown="3" w1520 {
          tunnel: ["A" "B" "C"] -> w1524
          frame 1, Default {
          }
          frame 2 {
          }
          frame 3 {
          }
        }
      }
    }
    "SHIFT" <- w1492
    n565 = Index Array(array=w1483) -> (element=w1482:dbl)  [unwired: 1 in]
    n566 = call "VALUE_CHANGE - ST1_RESULT.vi"("Numeric"=w1482) -> ("Boolean"=w1481:bool)  [unwired: 9 in, 1 out]
    n567 = global write "Global 1.vi" "EMERGENCY STOP"(w1481) -> ()
    n568 = call "Trigger_Loggic.vi"("error in (no error)"=w1471) -> ("error out"=w1476:errorcluster, "Array"=w1496:i32[])  [unwired: 9 in]
    n569 = global read "Global 1.vi" "PLC2 error"() -> (→"PLC2 error":errorcluster)
    n570 = global read "Global 1.vi" "PLC4 error"() -> (→"PLC4 error":errorcluster)
    n571 = global read "Global 1.vi" "PLC3 error"() -> (→"PLC3 error":errorcluster)
    n572 = global read "Global 1.vi" "PLC1 error"() -> (→"PLC1 error":errorcluster)
    n573 = for {
      tunnel: w1496 -> [w1531] mode=indexing
      shift-right: [w1535] -> w1489
      shift-left: w1495 -> [w1534]
      shift-right: [w1533] -> w1488
      shift-left: w1476 -> [w1532]
      n574 = case shown="21" w1531 {
        tunnel: [w1538 w1543 w1547 w1553 w1558 w1563 w1568 w1573 w1578 w1583 w1588 w1593 w1598 w1603 w1608 w1613 w1618 w1623 w1628 w1633 w1638 w1643 w1648] -> w1535
        tunnel: w1534 -> [w1540 w1545 w1548 w1555 w1560 w1565 w1570 w1575 w1580 w1585 w1590 w1595 w1600 w1605 w1610 w1615 w1620 w1625 w1630 w1635 w1640 w1645 w1650]
        tunnel: [w1537 w1542 w1549 w1552 w1557 w1562 w1567 w1572 w1577 w1582 w1587 w1592 w1597 w1602 w1607 w1612 w1617 w1622 w1627 w1632 w1637 w1642 w1647] -> w1533
        tunnel: w1532 -> [w1539 w1544 w1550 w1554 w1559 w1564 w1569 w1574 w1579 w1584 w1589 w1594 w1599 w1604 w1609 w1614 w1619 w1624 w1629 w1634 w1639 w1644 w1649]
        frame -1, Default {
          # "DEFAULT"
          n575 = Enqueue Element(queue=w1540, element=cluster{"CASE 2":T15} {"CASE 2"=enum."-1"}, error in (no error)=w1539) -> (queue out=w1538:refnum<queue>, error out=w1537:errorcluster)  [unwired: 1 in, 1 out]
        }
        frame 0 {
          # "SCAN BARCODE OP 10"
          n576 = Enqueue Element(queue=w1545, element=cluster{"CASE 2":T15} {"CASE 2"=enum."-1"}, error in (no error)=w1544) -> (queue out=w1543:refnum<queue>, error out=w1542:errorcluster)  [unwired: 1 in, 1 out]
        }
        frame 1 {
          # "DATALOG OF OP 10"
          n577 = Enqueue Element(queue=w1548, element=cluster{"CASE 2":T15} {"CASE 2"=enum."SCAN1"}, error in (no error)=w1550) -> (queue out=w1547:refnum<queue>, error out=w1549:errorcluster)  [unwired: 1 in, 1 out]
        }
        frame 2 {
          # "SCAN BARCODE OP 20"
          n578 = Enqueue Element(queue=w1555, element=cluster{"CASE 2":T15} {"CASE 2"=enum."SCAN2"}, error in (no error)=w1554) -> (queue out=w1553:refnum<queue>, error out=w1552:errorcluster)  [unwired: 1 in, 1 out]
        }
        frame 3 {
          # "DATALOG OF OP 20"
          n579 = Enqueue Element(queue=w1560, element=cluster{"CASE 2":T15} {"CASE 2"=enum."DATALOG2"}, error in (no error)=w1559) -> (queue out=w1558:refnum<queue>, error out=w1557:errorcluster)  [unwired: 1 in, 1 out]
        }
        frame 4 {
          # "SCAN BARCODE OP 30"
          n580 = Enqueue Element(queue=w1565, element=cluster{"CASE 2":T15} {"CASE 2"=enum."SCAN3"}, error in (no error)=w1564) -> (queue out=w1563:refnum<queue>, error out=w1562:errorcluster)  [unwired: 1 in, 1 out]
        }
        frame 5 {
          # "DATALOG OF OP 30"
          n581 = Enqueue Element(queue=w1570, element=cluster{"CASE 2":T15} {"CASE 2"=enum."DATALOG3"}, error in (no error)=w1569) -> (queue out=w1568:refnum<queue>, error out=w1567:errorcluster)  [unwired: 1 in, 1 out]
        }
        frame 6 {
          # "SCAN BARCODE OP 40"
          n582 = Enqueue Element(queue=w1575, element=cluster{"CASE 2":T15} {"CASE 2"=enum."SCAN4"}, error in (no error)=w1574) -> (queue out=w1573:refnum<queue>, error out=w1572:errorcluster)  [unwired: 1 in, 1 out]
        }
        frame 7 {
          # "DATALOG OF OP 40"
          n583 = Enqueue Element(queue=w1580, element=cluster{"CASE 2":T15} {"CASE 2"=enum."DATALOG4"}, error in (no error)=w1579) -> (queue out=w1578:refnum<queue>, error out=w1577:errorcluster)  [unwired: 1 in, 1 out]
        }
        frame 8 {
          # "SCAN BARCODE OP 50"
          n584 = Enqueue Element(queue=w1585, element=cluster{"CASE":T15} {"CASE"=enum."SCAN5"}, error in (no error)=w1584) -> (queue out=w1583:refnum<queue>, error out=w1582:errorcluster)  [unwired: 1 in, 1 out]
        }
        frame 9 {
          # "DATALOG OF OP 50"
          n585 = Enqueue Element(queue=w1590, element=cluster{"CASE":T15} {"CASE"=enum."DATALOG5"}, error in (no error)=w1589) -> (queue out=w1588:refnum<queue>, error out=w1587:errorcluster)  [unwired: 1 in, 1 out]
        }
        frame 10 {
          # "SCAN BARCODE OP 60"
          n586 = Enqueue Element(queue=w1595, element=cluster{"CASE 2":T15} {"CASE 2"=enum."SCAN6"}, error in (no error)=w1594) -> (queue out=w1593:refnum<queue>, error out=w1592:errorcluster)  [unwired: 1 in, 1 out]
        }
        frame 11 {
          # "DATALOG OF OP 60"
          n587 = Enqueue Element(queue=w1600, element=cluster{"CASE 2":T15} {"CASE 2"=enum."DATALOG6"}, error in (no error)=w1599) -> (queue out=w1598:refnum<queue>, error out=w1597:errorcluster)  [unwired: 1 in, 1 out]
        }
        frame 12 {
          # "SCAN BARCODE OP 70"
          n588 = Enqueue Element(queue=w1605, element=cluster{"CASE 2":T15} {"CASE 2"=enum."SCAN7"}, error in (no error)=w1604) -> (queue out=w1603:refnum<queue>, error out=w1602:errorcluster)  [unwired: 1 in, 1 out]
        }
        frame 13 {
          # "DATALOG OF OP 70"
          n589 = Enqueue Element(queue=w1610, element=cluster{"CASE 2":T15} {"CASE 2"=enum."DATALOG7"}, error in (no error)=w1609) -> (queue out=w1608:refnum<queue>, error out=w1607:errorcluster)  [unwired: 1 in, 1 out]
        }
        frame 14 {
          # "SCAN BARCODE 80"
          n590 = Enqueue Element(queue=w1615, element=cluster{"CASE 2":T15} {"CASE 2"=enum."SCAN8"}, error in (no error)=w1614) -> (queue out=w1613:refnum<queue>, error out=w1612:errorcluster)  [unwired: 1 in, 1 out]
        }
        frame 15 {
          # "DATALOG OF OP 80"
          n591 = Enqueue Element(queue=w1620, element=cluster{"CASE 2":T15} {"CASE 2"=enum."DATALOG8"}, error in (no error)=w1619) -> (queue out=w1618:refnum<queue>, error out=w1617:errorcluster)  [unwired: 1 in, 1 out]
        }
        frame 16 {
          # "SCAN BARCODE OP 90"
          n592 = Enqueue Element(queue=w1625, element=cluster{"CASE 2":T15} {"CASE 2"=enum."SCAN9"}, error in (no error)=w1624) -> (queue out=w1623:refnum<queue>, error out=w1622:errorcluster)  [unwired: 1 in, 1 out]
        }
        frame 17 {
          # "DATALOG OF OP 90"
          n593 = Enqueue Element(queue=w1630, element=cluster{"CASE 2":T15} {"CASE 2"=enum."DATALOG9"}, error in (no error)=w1629) -> (queue out=w1628:refnum<queue>, error out=w1627:errorcluster)  [unwired: 1 in, 1 out]
        }
        frame 18 {
          # "SCAN BARCODE OP 100"
          n594 = Enqueue Element(queue=w1635, element=cluster{"CASE 2":T15} {"CASE 2"=enum."SCAN10"}, error in (no error)=w1634) -> (queue out=w1633:refnum<queue>, error out=w1632:errorcluster)  [unwired: 1 in, 1 out]
        }
        frame 19 {
          # "DATALOG OF OP 100"
          n595 = Enqueue Element(queue=w1640, element=cluster{"CASE 2":T15} {"CASE 2"=enum."DATALOG10"}, error in (no error)=w1639) -> (queue out=w1638:refnum<queue>, error out=w1637:errorcluster)  [unwired: 1 in, 1 out]
        }
        frame 20 {
          # "SCAN BARCODE OP 110"
          n596 = Enqueue Element(queue=w1645, element=cluster{"CASE 2":T15} {"CASE 2"=enum."SCAN11"}, error in (no error)=w1644) -> (queue out=w1643:refnum<queue>, error out=w1642:errorcluster)  [unwired: 1 in, 1 out]
        }
        frame 21 {
          # "DATALOG OF OP 110"
          n597 = Enqueue Element(queue=w1650, element=cluster{"CASE 2":T15} {"CASE 2"=enum."DATALOG11"}, error in (no error)=w1649) -> (queue out=w1648:refnum<queue>, error out=w1647:errorcluster)  [unwired: 1 in, 1 out]
        }
      }
    }
    n598 = global read "Global 1.vi" "PLC5 error"() -> (→"PLC5 error":errorcluster)
    n599 = global read "Global 1.vi" "PLC6 error"() -> (→"PLC6 error":errorcluster)
    n600 = global read "Global 1.vi" "PLC7 error"() -> (→"PLC7 error":errorcluster)
    n601 = global read "Global 1.vi" "PLC8 error"() -> (→"PLC8 error":errorcluster)
    n602 = Wait (ms)(milliseconds to wait=u32 50) -> ()  [unwired: 1 out]
    n603 = global read "Global 1.vi" "PLC COMM"() -> (→"PLC COM.":bool)
    n604 = global read "Global 1.vi" "PLC 1"() -> (→"OP 10 & 20":bool)
    n605 = global read "Global 1.vi" "PLC 2"() -> (→"OP 30":bool)
    n606 = global read "Global 1.vi" "PLC 3"() -> (→"OP 40":bool)
    n607 = case shown="True" "stop 2" {
      tunnel: w1489 -> [w1499 w1505]
      tunnel: [w1499 w1504] -> w1487
      tunnel: w1488 -> [w1498 w1503]
      tunnel: [w1498 w1502] -> w1486
      tunnel: [FALSE TRUE] -> w1485
      frame False {
      }
      frame True {
        n608 = Flush Queue(queue=w1505, error in (no error)=w1503) -> (queue out=w1507:refnum<queue>, error out=w1506:errorcluster)  [unwired: 1 out]
        n609 = Enqueue Element(queue=w1507, element=cluster{"CASE 2":T15} {"CASE 2"=enum."STOP"}, error in (no error)=w1506) -> (queue out=w1504:refnum<queue>, error out=w1502:errorcluster)  [unwired: 1 in, 1 out]
      }
    }
    "stop" <- w1485
    n610 = global read "Global 1.vi" "PLC 4"() -> (→"OP 50":bool)
    n611 = global read "Global 1.vi" "PLC 5"() -> (→"OP 60":bool)
    n612 = global read "Global 1.vi" "PLC 6"() -> (→"OP 70 & 80":bool)
    n613 = global read "Global 1.vi" "PLC 7"() -> (→"OP 90 -100":bool)
    n614 = global read "Global 1.vi" "PLC 8"() -> (→"OP 110":bool)
  }
  n615 = Release Queue(queue=w66, error in (no error)=w72) -> (error out=w49:errorcluster)  [unwired: 1 in, 2 out]
  n616 = call <vilib>:"Clear Errors.vi"("error in (no error)"=w68) -> ("error out"=w53:errorcluster)  [unwired: 5 in, 1 out]
  n617 = call <vilib>:"DB Tools Close Connection.vi"("error in (no error)"=w53, "connection reference"=w67) -> ("error out"=w50:errorcluster)  [unwired: 5 in]
  n618 = Merge Errors(w49, w50) -> (w51:errorcluster)
  n619 = call <vilib>:"Simple Error Handler.vi"("error in (no error)"=w51) -> ("error out"=w46:errorcluster)  [unwired: 4 in, 4 out]
  n620 = call <vilib>:"Clear Errors.vi"("error in (no error)"=w46) -> ("error out"=w52:errorcluster)  [unwired: 5 in, 1 out]
  n621 = flat-sequence {
    tunnel: w52 -> [w1653]
    tunnel: [w1653] -> w54
    frame #0 {
      n622 = global write "Global 1.vi" "REMOVE VI"(TRUE ("remove_VI")) -> ()
      n623 = global write "DATA LOG.vi" "Auto Cycle On"(FALSE) -> ()
    }
  }
  n624 = property class="App"(error in=w54) -> (error out=w56:errorcluster, "App.Kind"=w55:T39)  [unwired: 1 in, 1 out]
  n625 = case shown="\"Run Time System\"" w55 {
    tunnel: [w1654 w1656] -> w57
    tunnel: w56 -> [w1654 w1655]
    frame "Development System", Default {
    }
    frame "Run Time System" {
      n626 = invoke class="VI" method="FP.Close"(error in=w1655) -> (error out=w1656:errorcluster)  [unwired: 2 in, 2 out]
    }
  }
  "error out 2" <- w57
